vi "UHR-Fleezers Control (host) -Leonardo 04-2018 V8_Redesign.vi"() -> ()   [LabVIEW 2013]
uses:
  <vilib>/Utility/miscctls.llb/LVMinMaxIncTypeDef.ctl
  <vilib>/Platform/TimedLoop/XDataNode/timing_clust.ctl
  <vilib>/Platform/TimedLoop/XDataNode/nitl_modes.ctl
  <vilib>/Platform/TimedLoop/XDataNode/wakeup.ctl
  <vilib>/userdefined/High Color/nirio_resource_hc.ctl
  <vilib>/Analysis/baseanly.llb/Mean (DBL).vi
  FPGA VIs Alex/Alex subVIs/Downsample1D.vi
  FPGA VIs Alex/Alex subVIs/Integrate1D.vi
  <vilib>/FPGAPlugInAG/PCIe-7852R/niLvFpga_Open_PCIe-7852R.vi
  <vilib>/FPGAPlugInAG/PCIe-7852R/niLvFpga_Reset_PCIe-7852R.vi
  <vilib>/FPGAPlugInAG/PCIe-7852R/niLvFpga_Run_PCIe-7852R.vi
  <vilib>/FPGAPlugInAG/PCIe-7852R/niLvFpga_Close_PCIe-7852R.vi
  <vilib>/Utility/error.llb/Error Cluster From Error Code.vi
  <vilib>/rvi/errors/niLvFpgaAdjustHostInterfaceError.vi
  <vilib>/rvi/interface/common/niFpgaWaitOnOcc.vi
  <vilib>/Utility/inputDevices.llb/mouseAcquire.vi
  downsample 1D array - double.vi
  <vilib>/express/express analysis/Spectral/Block/exnSpectralBlock spectral measurements PSD poly.vi
  <vilib>/express/express analysis/Spectral/Block/exnSpectralBlock spectral measurements PSD WFM.vi
  <vilib>/FPGAPlugInAG/PCIe-7852R/niLvFpga_Abort_PCIe-7852R.vi
  openfpgaref.8.6.ctl
  <vilib>/Platform/TimedLoop/XDataNode/XDataNode.xnode
  <vilib>/rvi/interface/nirviOpenFPGA/nirviOpenFPGA.xnode
  openfpgaref.initrf.ctl
  FPGA Bitfiles/UHR-FleezersInst_FPGATarget_intitializeRF201804.lvbitx
  <vilib>/rvi/interface/nirviMethod/nirviMethod.xnode
  <vilib>/rvi/interface/nirviCloseFPGA/nirviCloseFPGA.xnode
  FPGA Bitfiles/UHR-FleezersInst_FPGATarget_UHR-FleezersCont_IqK95Pvv9lYv5.3.lvbitx
  <vilib>/rvi/interface/nirviReadWriteControl/nirviReadWriteControl.xnode
  <vilib>/express/express analysis/Spectral/XNode/ExpressSpectralMeasurementsBlockNode.xnode
  <vilib>/Platform/TimedLoop/XDataNode/XDNodeRunTimeDep.lvlib
  <vilib>/Analysis/NI_AALBase.lvlib
  <vilib>/rvi/errors/niLvFpgaMergeErrorWithErrorCode.vi
  <vilib>/FPGAPlugInAG/PCIe-7852R/niLvFpga_ConfigureFifo_PCIe-7852R.vi
  NiFpgaLv.dll
  <vilib>/FPGAPlugInAG/PCIe-7852R/niLvFpga_ReadFifo_PCIe-7852R.vi
panel:
  in  "Tab Data Protocols":T1(tab)
  out "Extension":waveform(dbl)(graph)
  in  "Trap Pos. FB ON":bool
  in  "Set SP to Current Frc":bool
  out "Current Trap Delta":dbl=20.03845214843774
  in  "MCL Tracking":bool
  in  "Target Force (pN)":dbl=10.5
  in  "Save ave factor":dbl=1.0
  in  "Step Size (nm) 2":dbl=0.34
  in  "N Steps":dbl=20.0
  in  "Take Stepping Data":bool
  in  "APD 2 Offset":dbl
  in  "APD 1 Offset":dbl
  out "Mean":dbl=1.039039384389187 caption="Mean (pN)" format="%#_3g"
  in  "Calibration":u16(ring)=2 items=["None", "Position", "Force"]
  out "T1 X":dbl=-1.511158478291593 caption="T1 X (pN)" format="%0.2f"
  out "T2 X":dbl=0.5669202904867809 caption="T2 X (pN)" format="%0.2f"
  out "Difference":dbl=0.9442381878048121 caption="Difference (pN)" format="%.2g"
  out "Data Period (s)":dbl=1.4999999999999999e-05 caption="Trap Data Period (s)" format="%#_6p"
  in  "Tab Action Shortcuts":enum32{"Actions", "Calibration", "Fishing"}(tab)
  in  "Use Full Offset?":bool=TRUE
  in  "Cal/Data Acq. Spot":bool
  out "Fish Status":u16(ring) items=["Off", "Approach", "Wiggle", "Extend", "Tether Found"]
  in  "Toggle AFish":bool
  in  "Offset 2 Set":dbl=2.0
  in  "Offset 1 Set":dbl=1.0
  in  "Cal @ (MHz)":dbl=20.0
  in  "W/ Offset 1":bool=TRUE
  in  "Offset 1 Start (MHz)":dbl=13.0
  in  "W/ Offset 2":bool
  in  "Offset 2 Start (MHz)":dbl=16.0
  in  "Trap 2 Bead Size (nm)":dbl=1000.0
  in  "Trap 1 Bead Size (nm)":dbl=1000.0
  in  "Extend Min F":dbl=1.0
  in  "Extend Min TD":dbl=8.0
  in  "Extend dTD":dbl=5.0
  out "AF Time":u32
  in  "Wiggle time":dbl
  in  "Wiggle TD":dbl=1.0
  in  "Max TD":dbl=15.0
  in  "Min TD":dbl=8.0
  in  "Approach dTD":dbl=-5.0 format="%#_13g"
  in  "Stop All":bool=TRUE
  in  "Tab Control Display":enum32{"Main", "Imaging", "Display All", "FFT"}(tab)
  in  "Clear FX":bool
  out "Force-Extension":cluster{"x":dbl, "y":dbl}[](graph)
  out "Force":waveform(dbl)[](graph)
  out "APD Chart":waveform(dbl)[](graph)
  in  "Ext Offset (nm)":dbl
  in  "Take Green\nLaser Image":bool
  out "APD 2":T2(plugin-control) caption="APD 2 (Cy5)"
  in  "Flip Green Filter":bool
  in  "Set X Only":bool
  in  "Set Y Only":bool
  out "APD 1":T2(plugin-control) caption="APD 1 (Cy3)"
  out "Detection Laser Y":T2(plugin-control)
  out "Pointer Y (V)":dbl=4.0025870540482815 format="%_3g"
  out "Pointer X (V)":dbl=4.635613485356835 format="%_3g"
  in  "Set Confocal Spot":bool
  out "Detection Laser X":T2(plugin-control)
  out "All Signals":waveform(dbl)[](graph)=[{"t0"=timestamp(2751.0000000002074 s since 1904-01-01), "dt"=0.02, "Y"=[0.0, 0.0, 0.0, 0.0, 0.0, 0.0, 0.0, 0.0, 0.0, 0.0, 0.0, 0.0, 0.0, 0.0, 0.0], "attributes"=variant("NI_ChannelName"=variant(string "APD 1"))}, {"t0"=timestamp(2751.0000000002074 s since 1904-01-01), "dt"=0.02, "Y"=[0.0, 0.0, 0.0, 0.0, 0.0, 0.0, 0.0, 0.0, 0.0, 0.0, 0.0, 0.0, 0.0, 0.0, 0.0], "attributes"=variant("NI_ChannelName"=variant(string "APD 2"))}, {"t0"=timestamp(2751.0000000002074 s since 1904-01-01), "dt"=0.15, "Y"=[-0.020049210394969354, -0.02003592505550746], "attributes"=variant("NI_ChannelName"=variant(string "T1 Y"))}, {"t0"=timestamp(2751.0000000002074 s since 1904-01-01), "dt"=0.15, "Y"=[0.03074231675925172, 0.03074526419399293], "attributes"=variant("NI_ChannelName"=variant(string "T1 X"))}, {"t0"=timestamp(2751.0000000002074 s since 1904-01-01), "dt"=0.15, "Y"=[2.9160941496017294, 2.916128360850853], "attributes"=variant("NI_ChannelName"=variant(string "T1 Sum"))}, {"t0"=timestamp(2751.0000000002074 s since 1904-01-01), "dt"=0.15, "Y"=[-0.002644972968316131, -0.002638961391604115], "attributes"=variant("NI_ChannelName"=variant(string "T2 Y"))}, {"t0"=timestamp(2751.0000000002074 s since 1904-01-01), "dt"=0.15, "Y"=[-0.011335016186436862, -0.011341032214389745], "attributes"=variant("NI_ChannelName"=variant(string "T2 X"))}, {"t0"=timestamp(2751.0000000002074 s since 1904-01-01), "dt"=0.15, "Y"=[2.746599475081634, 2.746642933439132], "attributes"=variant("NI_ChannelName"=variant(string "T2 Sum"))}, {"t0"=timestamp(2751.0000000002074 s since 1904-01-01), "dt"=0.15, "Y"=[-0.526083166086966, -0.5261552546492463], "attributes"=variant("NI_ChannelName"=variant(string "T1 FB X"))}, {"t0"=timestamp(2751.0000000002074 s since 1904-01-01), "dt"=0.15, "Y"=[3.0920304879909737, 3.0920243537705665], "attributes"=variant("NI_ChannelName"=variant(string "T2 FB Sum"))}, {"t0"=timestamp(2751.0000000002074 s since 1904-01-01), "dt"=0.15, "Y"=[-0.7128125059590501, -0.7128388598091219], "attributes"=variant("NI_ChannelName"=variant(string "T2 FB X"))}, {"t0"=timestamp(2751.0000000002074 s since 1904-01-01), "dt"=0.15, "Y"=[2.9122738731040343, 2.91227808465834], "attributes"=variant("NI_ChannelName"=variant(string "T2 FB Sum"))}, {"t0"=timestamp(2751.0000000002074 s since 1904-01-01), "dt"=0.15, "Y"=[-0.0023344523453474137, -0.002339854121524665], "attributes"=variant("NI_ChannelName"=variant(string "PSD Y"))}, {"t0"=timestamp(2751.0000000002074 s since 1904-01-01), "dt"=0.15, "Y"=[-0.0026477858821374683, -0.002642139957884409], "attributes"=variant("NI_ChannelName"=variant(string "PSD X"))}, {"t0"=timestamp(2751.0000000002074 s since 1904-01-01), "dt"=0.15, "Y"=[0.014415417950986964, 0.014429639576402777], "attributes"=variant("NI_ChannelName"=variant(string "PSD Sum"))}]
  in  "Signals to Plot":i32(listbox)=9
  out "Trap Disp. Freq. (Hz)":dbl=6.666666666666667 caption="Freq. (Hz)" format="%#_6p"
  out "Display Period (s)":dbl=0.15 caption="Period (s)" format="%#_6p"
  in  "Trap Disp. Downsample":i32=10000 caption="Downsample" max=20000
  in  "APD Disp. Scale":dbl=0.1 caption="Scale (Divide,\nfor above plot only)"
  in  "APD Disp. dSamp":i32=2 caption="Integrate" min=1 max=30 step=1
  out "APD Display Freq. (Hz)":dbl=50.0 caption="Freq. (Hz)"
  out "APD Display Period (s)":dbl=0.02 caption="Period (s)"
  out "FFT 1":cluster{"f0":dbl, "df":dbl, "magnitude":dbl[]}[](graph)=[{"f0"=0.0, "df"=16.666666666666668, "magnitude"=[-331.1367572010275, -79.05506245821404, -86.61411242440559, -88.4728176091699, -90.3181253945935, -94.12566333707997, -92.52740723119955, -94.92192587982518, -99.60936585245742, -96.87568627870715, -94.02570383337763, -83.8058550151726, -97.57441397235512, -101.59968530846606, -101.523049255742, -103.35038532190343, -101.58594091014982, -102.96098031851216, -91.39759462745924, -103.75019963279499, -104.45030075054324, -103.04245334279298, -104.0720279134107, -106.06482372394834, -103.69131867828104, -104.40395035115309, -105.96420043276396, -107.6735556337804, -106.673030006608, -107.34889066208132, -108.05626565233933, -106.25659018850432, -105.29934513380842, -105.43096056709592, -108.3728498841465, -106.0555440144992, -105.78001282181421, -107.48741857324953, -108.67624970548897, -105.39976667156175, -105.91413119232612, -109.4222808198164, -107.0898971593174, -107.91164191890915, -108.26032038855709, -107.58332347164534, -108.23559688234297, -108.01271040303237, -107.66511723652701, -106.51901583170391, -109.27249501469946, -108.55647681594805, -107.93499259231463, -107.05068166453935, -109.13641475410455, -109.29679733781423, -108.19360835527803, -109.57747591546632, -109.58364591011674, -110.47061433372711, -109.8144340420426, -108.79067462293897, -107.54887553357234, -107.99559866705923, -108.85023923652685, -109.68733225238618, -108.51101278437793, -108.51620475114115, -108.22212402200637, -104.63726950302143, -110.2989919678048, -107.61796444414897, -108.68882962798736, -104.79193983043893, -103.59504263746938, -93.64633660288543, -101.9191640501395, -105.73717393151816, -108.92572458793902, -107.43962662800902, -107.79595323081325, -107.0923101993207, -108.17603277205289, -107.87074270713183, -109.20899066381877, -108.61832060412445, -109.10072003106593, -105.76480632823524, -108.60877649218978, -109.67541158970121, -110.2286232768028, -109.84952155309578, -109.33772024076384, -109.95251642394683, -110.14777282585466, -109.13825677905699, -110.05989365698167, -109.39359990189426, -110.56255614635295, -109.66477183197163, -108.9397158528824, -110.26529907650465, -109.20049464984628, -108.20183857013548, -109.09752250184418, -108.00440442238454, -108.35465963524055, -111.16774134451799, -110.34812550238405, -108.94506763426756, -108.72845542102493, -109.41512344014713, -112.44661664432377, -110.35437330889101, -111.32939440655925, -109.42989530434981, -110.98084669076195, -111.92160561143541, -108.57755551751093, -111.40042616180912, -110.15284955891853, -112.21455132279115, -111.40787773511747, -108.82949641635288, -110.13442122547907, -111.42229298204664, -112.06314940885191, -110.6015308813694, -109.51144097251623, -111.15989713761475, -110.25535755335385, -109.65868178057926, -110.51649885452997, -109.77194745285269, -108.4234206864394, -109.50892632093968, -109.46471287444389, -107.92241289271415, -109.72283805386196, -108.63426821579918, -110.37316681536255, -111.09713996884652, -110.32903619589223, -105.32012665515045, -107.36858557554393, -108.00382215905725, -110.06430686942338, -108.81666625979916, -110.01277074453823, -110.94194741225512, -109.65934609082873, -107.80979136006962, -112.81333866824724, -111.61474300955487, -109.83998277184975, -109.45953946904639, -109.79640584952526, -108.19172301667324, -109.28894656674316, -107.61471301278785, -108.83814006090513, -109.08866847726084, -108.20250571862371, -107.96222236861584, -107.03811197900873, -108.93533000393974, -107.74482548035408, -110.79811544577694, -111.1387476496877, -107.42970105883512, -109.18442281176472, -108.73546184641192, -108.71800246690864, -108.51945944378063, -108.06825856571285, -107.27210712368412, -108.12304695877637, -107.84933283677306, -109.73682373154998, -109.32284761503395, -109.31328817453769, -106.68762108642842, -109.79203616876461, -109.9020278896408, -110.27080024357275, -108.54152101558762, -111.00464391726017, -112.42244020766577, -110.82707315747889, -111.00344011890857, -109.90461839395674, -109.42877207451863, -109.73549298167016, -111.67494793393293, -108.85799077901427, -108.5348443278263, -109.803781083881, -108.30644755543659, -108.5079527456017, -111.2055351312823, -108.53089994340155, -108.01739789012176, -108.70360662855235, -107.95873456794631, -109.58297170693093, -108.9372401694271, -110.15921663527153, -109.22399119911955, -110.89883651739237, -108.92840112258382, -110.0545300523626, -109.05961065387005, -109.45831398589371, -108.61239387653227, -110.13001256174265, -108.80060224137931, -109.46327400696283, -108.0177965824709, -109.29727944627197, -110.3237255895986, -109.03258262543821, -110.97880178489321, -109.70034895077919, -111.16405638194153, -109.17324451464711, -109.65698250854277, -108.96750235822178, -112.00534231585624, -108.69274607723942, -108.98110446396657, -108.40723795464795, -111.44459094807324, -111.74799245277113, -111.1601960491512, -108.92048232753773, -110.30506377784799, -111.33145973979093, -110.91850998672503, -110.33684985776448, -108.90206518366908, -109.28458878227542, -108.98773986023751, -110.85813863075646, -109.00041591105906, -110.84543686681204, -109.84382395806176, -109.69722434763266, -108.50915601095721, -107.80829925826895, -110.59736107582401, -109.75377770317087, -109.3992084496136, -110.51151565846742, -112.49753959826434, -109.7299632589479, -109.54070743868353, -109.90314341132164, -111.05974202976806, -109.03766862152392, -109.46667095459878, -109.52800799036197, -111.3163121356807, -110.07817134522178, -108.69251657453547, -109.40472158898045, -109.71400709815576, -110.60534468715097, -109.46937396724682, -107.70342491418788, -109.86331122597839, -108.64971387994616, -110.90117371097081, -108.34928840565928, -110.04172889660904, -111.52979926554961, -110.34759300823305, -109.62712781837159, -109.24131154553284, -110.23196152450447, -108.68509612326807, -108.0246905483419, -106.61876139289784, -101.5519630114271, -80.57695480953835, -102.03744443354402, -107.1449217193017, -110.0695213407169, -106.61597783999268, -110.79221011808191, -109.58974545931426, -109.1149802216988, -109.20993813088597, -109.63768480465863, -110.10428394219181, -109.08445084271477, -108.83472375362581, -109.69508502050168, -108.05588796178941, -110.62586360101581, -109.95315261676905, -107.52208264977473, -108.80708007514875, -110.43484881098874, -110.45942171588936, -107.83804717866751, -109.98973910294193, -109.3496496054193, -108.425252911127, -110.94579264380809, -108.54181722177951, -108.67696070083541, -108.4150202151644, -109.24973583101504, -112.0454922608961, -111.29046597340738, -110.75018248960077, -109.38326363603683, -109.2033340336957, -109.45076170874889, -109.52878049853727, -109.32340869724774, -110.98123395128233, -110.75736340635505, -109.7218385823809, -107.97422606064993, -109.77313701758703, -110.95948744392717, -110.08996774172691, -108.51011830110778, -109.78063140243836, -110.65996628628228, -109.83684298615616, -110.33329049188029, -110.13755118968292, -110.3717925645783, -108.55302219178951, -106.86811628734195, -108.6302156589162, -108.75341391045045, -108.32589578384841, -108.70061474734084, -112.30742263527534, -109.16842570592085, -109.29767035534508, -108.87829025017463, -108.2255616391397, -108.4316108616088, -108.82995906929271, -110.40135575415563, -109.51623498946435, -109.79409808792403, -107.03832759632121, -108.36534528684132, -109.72010868372905, -107.90933028179892, -106.95643597294047, -111.29929166165778, -110.23001135794706, -108.98838015381585, -109.79115357104436, -108.18627479511115, -108.14988122174307, -109.12074063466532, -109.41904850488358, -111.40409873721113, -108.83156790193294, -108.77032248953847, -108.88363158686694, -108.47515048290681, -105.94172147874599, -109.38146940214403, -109.21277078848794, -108.11309390545507, -110.70840012427504, -109.5504457849329, -109.52330684534209, -110.06776026911132, -108.21949434182314, -111.21266686269992, -108.78581501170974, -108.43115799297222, -109.63260325780062, -109.84070220619535, -109.72041980780126, -110.29615941882527, -110.60316734262464, -108.79165446414692, -110.95840439895592, -109.64926233107009, -109.16526769544322, -108.65292362430982, -109.56113898129935, -109.85693046339026, -108.92316027325207, -109.79492493553914, -109.38157962945887, -110.24545136266825, -109.30031463492487, -109.0795429936869, -111.4091719525013, -108.63499083917162, -108.43863465339358, -109.23207864880891, -111.21947487191643, -109.24525201480154, -109.56842406077318, -109.46711940800672, -111.91389548262572, -108.15655736690546, -108.71882059966947, -111.26328503478568, -110.95027143873176, -108.4853106242357, -110.36902802777546, -109.9314203579182, -108.77686164101732, -108.71871020068312, -111.04829661168574, -109.95072655339462, -109.88221342875462, -109.53241732756136, -108.2625005404823, -108.00677030040697, -110.19659317581693, -108.93858924796267, -109.46817875483995, -110.78063992017232, -111.11066570318451, -110.78774336696706, -109.19199744617812, -108.54914256407436, -109.28414960420909, -110.64143585101183, -110.5855350821307, -109.47578632252726, -108.89705360836223, -109.89214013612292, -107.93271261027171, -109.32631601340563, -108.60274611341092, -109.40110159872573, -110.889237682208, -110.01391165813328, -109.99747108785071, -108.65542819213674, -110.37211847668736, -110.44656500845738, -110.8128133834973, -108.8909299260433, -110.19551227077532, -111.37647266643523, -110.83802189730321, -109.98519377913681, -110.52378970770522, -108.16970420057817, -110.70974729773344, -110.76836765494402, -110.26884275594577, -109.22041044268806, -109.87809744746195, -107.76823252107832, -109.12119474042969, -110.28066108731146, -108.55000033509207, -110.18152097767907, -110.73030521152278, -111.49470908029893, -110.2320929919509, -110.03370979233021, -109.79181668155233, -108.6673501209991, -109.86695766650877, -107.88926518046961, -110.95525003776572, -109.18130359755742, -110.42618009658618, -107.90341931158893, -111.44736855661769, -110.72634267386593, -109.29945988519303, -107.67889101961411, -108.81148059987765, -109.13375212757057, -109.8122873383549, -109.80176697684155, -109.96342275204768, -109.90406635707086, -108.75674342748256, -110.12362902701081, -109.82151095527837, -108.62543344241836, -110.09171852771195, -110.21434637862887, -109.97254504855631, -109.27043209093468, -111.35149588204125, -110.12399876776051, -111.65983675538546, -109.28788875768564, -110.86554069990251, -111.26990906470603, -108.60956517491746, -111.49613890850938, -111.79685722966795, -109.26269485364045, -110.38555615546439, -109.40641023162068, -110.966136593156, -108.78892524584494, -110.29340727375603, -111.44032043281035, -109.95212021173755, -109.79233511584334, -112.41184021118175, -109.73687851881148, -108.65493879781806, -110.76132988919045, -108.43230346094671, -110.32968175895853, -110.29890782023821, -108.77609076424456, -110.3298662333555, -109.47734504217333, -108.2677295732245, -109.21234363352882, -107.83278941978479, -108.85136784424789, -108.43241251530755, -109.76609391460555, -108.53204373005357, -110.9660641972934, -110.3152512161094, -110.72570499399905, -109.23877906286317, -111.72407743101837, -109.20311421918561, -108.06021800233717, -109.29288625761943, -108.78395253409145, -111.85250172876302, -108.78827588901797, -109.79775055719482, -109.12089297455859, -109.49896359356035, -110.34432647103819, -107.94700097960238, -109.30489238477631, -108.89170290869342, -108.82574563272509, -110.11024077194833, -107.37946433552314, -109.60167933458756, -107.80625057819019, -110.11489057210264, -107.35436859378505, -105.69819484613895, -109.11280625683739, -109.27770293057978, -107.7053735252589, -109.75022444894368, -109.3310543596577, -107.87683693707739, -108.19931495338068, -109.26462246191564, -106.71885779297867, -100.00018022217961, -92.54434511397295, -107.20472143807373, -107.39203415155283, -110.04461177268398, -108.48860496315312, -109.0057168110333, -108.37627790492552, -108.4108380728248, -109.65509454313073, -109.64243000632982, -97.04219069306761, -109.0928856629964, -107.9760697315632, -107.52611064047497, -108.87702814778996, -109.08437599027614, -110.70097118837974, -109.00969860961283, -110.38275386163214, -110.0699155421545, -106.91498895181175, -106.22178738309017, -109.36827866896039, -107.59953130968307, -109.19516217272808, -108.31502495393616, -109.384158926223, -107.11670654202719, -108.09436312738853, -110.14559230873704, -109.84997663447679, -107.83465335309926, -108.60947100624459, -108.9932479423645, -109.17174810371898, -108.79457339828916, -109.40909327982367, -109.6328723628302, -109.51081854476179, -107.63054408568418, -109.63728404010122, -108.51163794839918, -107.55002282725216, -108.97796212764939, -107.24648164623483, -112.21470452291085, -108.74294024554423, -109.62070777514892, -108.05768666239368, -109.8224946685739, -109.34575507446003, -108.53536952609525, -109.60789300457671, -107.56681538208278, -109.22777325016398, -108.79047910308894, -110.10332477250668, -108.00206387955672, -108.45604004720035, -109.00645795765472, -109.81039564269616, -108.92785144634745, -108.3978471520567, -107.94411095685999, -110.53486519304262, -108.8773780319227, -109.03345093296107, -107.30746693745031, -108.54277704832029, -108.77629108166091, -108.91111762599647, -107.74965195880401, -109.97375370738439, -109.76326492689246, -107.91717581777407, -109.0730556927617, -107.66804873204664, -110.40438871064791, -108.05794247751498, -108.80206615156494, -107.51329354700796, -108.83687012994949, -107.57713176895379, -107.94774159581414, -109.41894615439651, -107.10869425078764, -110.51480854078629, -108.92221367099775, -109.91358786461535, -110.1744263092835, -109.30795472883494, -107.91359710691006, -109.77888185049835, -109.52060975706438, -108.66686651982212, -108.71041801553639, -110.13619546359467, -108.87957097273856, -109.72150387215271, -109.00776068810654, -109.70251113927438, -110.75769213896399, -108.53234896741436, -109.69439526582246, -110.15412541604617, -108.25183374628219, -107.97402569656481, -110.34920156998648, -108.45106995186384, -108.82031145748209, -111.38690005057539, -107.01968459818563, -110.3044500039584, -110.8755481852125, -111.08915057663255, -107.94824988655199, -110.21669144934839, -109.90539774633154, -109.58985438756767, -110.12258796623348, -109.41689951612143, -109.31128210476795, -109.00258476567323, -109.11093063041056, -108.83347064311234, -108.32685287566952, -109.44770946560935, -108.40145063144861, -109.68448193892085, -108.76525439243828, -107.62837139034596, -107.39300298848994, -109.36993934990318, -109.2465218489418, -106.66307369796812, -110.15891092764934, -109.57151745419041, -108.92425698310808, -109.8036704717834, -108.79751146756549, -109.25926431818017, -108.46260574057584, -109.1967554647261, -110.63319560262356, -109.02343067385144, -111.22073171487528, -109.4731095097105, -109.69335000085164, -109.48782989577005, -107.95204227683271, -108.19468255763758, -111.36195112053247, -109.55696116543685, -110.3130767640534, -108.9621824253354, -109.99735074896789, -109.20198058456344, -108.12100614259485, -111.27227490807289, -110.09248554008288, -109.14395535060149, -110.80882692379708, -109.22632926901655, -108.64497210802793, -111.00030482190711, -111.1317849358033, -107.43140429257826, -107.9783302193555, -109.2639893652291, -108.97008485446163, -108.66556668859064, -108.12995785876932, -109.73001061107855, -108.09691302413727, -110.68391499215569, -112.78583642012705, -108.7093037763389, -110.67868795924797, -109.0190959349128, -108.36247198231372, -109.82829353258869, -108.24916379311045, -109.84154533905823, -108.55470160833775, -109.75438989348815, -108.82865632118325, -107.63622268162582, -111.00943492886312, -110.81824358463759, -109.46028423652966, -107.52479398900992, -108.99087806823736, -109.94494831750349, -110.26788355564504, -109.8954055022304, -106.9478122391182, -108.91705388158901, -107.76095584490312, -109.28456723055147, -109.7982307261767, -108.98552661346622, -109.98937979783426, -110.57907422426224, -108.68113463944836, -108.06257240208589, -110.0707224529617, -109.19515280354733, -109.35868842818849, -110.37311467065695, -109.0404734478992, -108.16686395270187, -108.61859220485148, -109.19986437876149, -108.19707189725302, -110.06564239663074, -108.87850403465154, -110.63824157544798, -107.36918104067212, -108.7008736325543, -110.9359398265406, -111.08529123080929, -108.44209934821818, -109.79529621208783, -108.38917887958179, -108.169117639508, -109.24332926356216, -110.50584058811704, -109.63592524002665, -109.32261039377495, -109.16720880524552, -109.3084314664462, -109.5812223978583, -107.70213196487856, -108.0557884982431, -110.67058020007828, -111.68459781023608, -109.66270627185824, -110.52536245663693, -109.70208409132103, -108.78645420809342, -109.23122088059863, -109.24601474121832, -111.25604763816514, -109.50225851581177, -107.32434217163818, -109.28548556764925, -107.59972621660836, -110.46928774723048, -109.25950101547609, -110.32016453935465, -107.78482761561703, -107.89462895091089, -107.51366154391481, -108.08036891159172, -109.53371809947035, -101.2452927166745, -109.32763325689056, -107.52166868423687, -109.89648659445174, -109.11350200980485, -109.81336712738089, -110.02799517445062, -108.02767143538516, -107.97850220501483, -109.50772934896838, -109.31069875721964, -108.49991657749598, -105.60880911233095, -109.79128597340213, -106.91084537903113, -107.84880087118997, -109.63628170511824, -109.03203967193224, -110.64186113413658, -110.98027990365594, -112.33841002907062, -111.01793075565425, -108.58025797022215, -110.4259296883756, -110.38643255981424, -108.93051671115133, -110.97544177116494, -108.63883100482677, -108.37581711765226, -108.90240163126536, -107.94688047875466, -109.9482937437732, -110.09097112364414, -110.09805032265376, -111.44307114024532, -109.15483789122554, -110.9713708217832, -107.8548737634672, -111.41418477109195, -109.45699779859628, -97.03595099331734, -109.16746744169623, -109.66209204485918, -112.57048704774604, -109.73989735035725, -108.16252575067017, -110.7546980664636, -108.91536673403449, -109.20509151422344, -111.0260632167785, -109.62924582406518, -110.45466277291722, -110.2973970018937, -109.67550222925419, -108.84481022020094, -107.23686414357573, -111.79004633370906, -109.85453094194085, -109.45617270081004, -110.73920606732504, -108.90879956851099, -109.67774425528265, -109.4745715721361, -110.18080454693559, -109.26079184315502, -109.41692499885505, -109.02240975088358, -107.80833423058168, -109.32657361431549, -107.87138278655101, -110.910364670719, -109.70067156846706, -108.55301754282077, -109.4243252157005, -109.77567725161107, -107.83737232063925, -110.36509412773016, -109.6371048811367, -109.49430894422814, -108.55509251499753, -108.03996302911446, -110.4385715838736, -110.08864436068788, -109.48922484379962, -109.90865554258562, -109.7491963238264, -110.04796094537969, -107.413043439116, -108.54229076126079, -108.2522516728666, -109.75464941327974, -110.26795832300996, -109.28073673851144, -108.62990200974927, -109.89408067552287, -109.09160284731726, -109.90740624925795, -109.92534708896517, -109.79578862362752, -109.97278346890566, -107.80679350393824, -112.81728446281548, -108.09689504419987, -109.89549991422173, -108.43930976031248, -109.95153099843282, -108.18277483720716, -111.89607792605433, -109.52567003805, -109.17125106979698, -109.64300739407085, -108.21045178846524, -109.64036472149706, -109.02324448538845, -109.039163008889, -110.41006510134076, -109.50289952116489, -110.4732620447796, -110.08777181504614, -110.15589511434341, -109.55705089158471, -109.2547682932589, -110.86823885471617, -109.96330502176939, -109.85995369810554, -110.63211290903473, -112.08007783432191, -110.24725218052279, -107.62861148917592, -110.08691795849435, -108.89793794632287, -111.07702220466341, -109.46946126482341, -109.19747345337464, -110.70018609416007, -109.66366205691908, -110.78032312133551, -108.05724200456513, -108.195661625627, -110.90724508408255, -110.08307674771669, -110.76863516643007, -110.46620425061583, -109.16986788877276, -109.61921294239114, -108.51159432329543, -109.96308336765689, -107.38178944242856, -111.95930944846394, -109.3329826827624, -109.59119636368249, -108.83148571828912, -110.46194288788257, -105.87694286145472, -107.985886302892, -109.2975019660806, -111.05138725716857, -109.60005889204612, -110.92871351729086, -110.73480546964537, -108.41587420326718, -109.84275465824477, -108.8249071047676, -107.65358887817105, -108.3254150042995, -111.47362100321767, -112.7287536850025, -108.8217125660507, -109.50232320231771, -110.29587061625348, -109.30644535112089, -107.69178032077258, -110.84522325672016, -109.3735891463141, -109.12506388923123, -109.65582307934665, -111.11427272192576, -112.19827973435466, -109.11306367925813, -108.19203577968261, -107.89831568266465, -108.85805249169313, -109.51100049661844, -111.71546684086955, -109.53880495724334, -107.07739286222231, -110.66836728754211, -111.5415170557177, -110.16051267940297, -110.6107546662698, -111.36389129556191, -107.77888179117923, -110.34160392509817, -109.61287125994414, -110.23791773883013, -111.00669159903549, -110.97165069538953, -109.43965413392434, -110.6813161690388, -110.31441293654314, -111.96129906273796, -108.15998218707462, -110.08095912053633, -109.41084567452768, -109.28774416263552, -110.80159950384204, -110.41956747809755, -108.85005186267244, -107.9069227847757, -108.84249369063123, -109.92569208845894, -109.34109797584448, -109.41334788055491, -108.76462023086997, -108.22069272136177, -107.0786679601274, -108.30206755098202, -108.57613406368954, -110.83330887636482, -111.93966942736989, -109.76373713473264, -108.25782074884941, -108.16490627215555, -109.93351470267982, -110.75525684428368, -108.22814762283093, -109.73442331991602, -107.53145627482685, -108.27195221226805, -110.33032779278457, -109.48951857415828, -108.12599093700939, -107.97627415508097, -108.81426859968796, -111.21764717894752, -109.80856212352333, -110.92658779118501, -109.71551885834796, -110.38682741010847, -108.87671328341361, -109.68368600774755, -108.35359806351899, -111.7519400010676, -109.89407081573103, -108.24301180922755, -110.00646944788126, -108.6685299083706, -107.52856885980722, -111.7622363038509, -111.0025144494897, -108.64719599357296, -110.62968467177518, -108.821509935539, -107.94915453463719, -111.53070432277694, -109.87282048586256, -110.71167589371663, -109.79225006081626, -109.96203471712074, -110.29921092232489, -110.10644439440416, -111.28815007382043, -111.19165661703703, -108.46024117100558, -110.22528296512183, -110.32184972386672, -110.05120383416072, -109.78792549362107, -109.00355659956696, -108.85989369286315, -113.00899556732638, -110.91756826567867, -111.25016866167897, -111.84225040552181, -110.54451635944174, -110.72722829912917, -109.60759702177283, -110.49362602516815, -108.74419542915284, -110.3379671069179, -109.66259088220754, -110.45956400953156, -109.13956157147233, -109.27130155486806, -110.83015602667983, -109.17970724944131, -109.09662765889193, -108.0447366108107, -108.9536269357457, -110.35663108940085, -108.73418835472056, -113.42965806805827, -111.81270536656905, -110.06155590173537, -108.76582224646269, -106.7488061675813, -108.5700320158723, -111.11038264410035, -110.41435767488723, -109.12763443489911, -109.30517580756394, -111.61251165371237, -109.8116632664339, -109.36845864976851, -109.00390009629231, -110.54359197165573, -109.52629258465976, -110.75932197632896, -109.50903215359567, -107.42652056246085, -107.81146496533543, -103.22224383145215, -108.53803076819163, -109.78623360072066, -109.66306634612869, -110.80245829141279, -111.87835085452016, -102.27372781471168, -111.27763038431458, -108.45838423437681, -108.79077917058028, -109.31951755762685, -110.05415097017186, -109.5535934823387, -111.62732254641111, -110.73478247119641, -109.9468722686683, -110.39698367573979, -109.30612942398305, -109.7578384694043, -109.34817295524313, -105.56944757301993, -110.1940418750125, -109.27076023513962, -111.03491935225027, -112.2980497521063, -110.65725497955563, -109.0567530102422, -110.31700596563523, -109.64508026365678, -109.6190471404421, -110.52566833759428, -109.68595899227789, -109.7431160985074, -110.4798230300751, -109.45506977604765, -110.69504157940786, -110.63067849573177, -108.06456949500138, -107.99354148885966, -108.11349194720599, -109.15944121207349, -110.61766925164031, -110.14145801314527, -110.67420842201165, -111.91532881806512, -112.15901550030345, -109.94774413630104, -109.2819568305201, -110.94623189179737, -110.17685430287735, -110.39082916961016, -109.53953238698966, -110.76940623620611, -109.89327922318515, -109.10275695043765, -110.21445972656734, -110.58968777252528, -110.57016757660259, -109.59208496373341, -109.07946946465374, -109.10762003745964, -110.36892993974607, -109.81864495218393, -112.12972189864566, -109.26185849434863, -111.56305819991357, -111.36019621828058, -110.3397604159226, -109.58675612753163, -110.58041217474447, -106.34739062044932, -108.6722699609389, -110.03906060709869, -109.16794717548382, -109.65012481802809, -109.35377624077988, -110.51889143862303, -110.03397458059777, -110.7981307056636, -110.56653507062292, -107.61367005067231, -109.99279736988825, -111.79875182878175, -108.60382315996031, -109.71381533228038, -108.60388131505613, -107.0933685540362, -107.86037690830757, -108.40980028847238, -108.83869602763895, -110.76921375395764, -109.96766364716046, -110.8256171465781, -110.13805084291067, -108.5349140035878, -110.57158437465219, -110.8920694413417, -108.71646695477324, -108.33274238445665, -108.96152108305608, -111.03750932994224, -109.48915027983756, -110.29725207211165, -110.79527247268442, -109.47969936716117, -109.79306701834035, -110.16840035577498, -110.29840230783668, -109.15306387075587, -110.72651274964761, -109.08881658764956, -110.8349724030761, -110.64653625576447, -111.40392562616867, -109.94581588927414, -108.85136340231294, -109.77228546607624, -111.48297395390018, -109.7334001251941, -109.30537415590783, -109.63937411233408, -109.69785848648013, -109.3523781030017, -112.04667421182404, -111.56311816195343, -108.18548447362308, -110.63388993686104, -111.39768634137992, -109.87157345395542, -108.6734208287271, -109.46213300216168, -111.75774769437145, -110.10245994173216, -109.52385139033495, -110.96513097775451, -111.8709319163154, -111.54948269614047, -110.29760900080463, -108.52168175904663, -111.09033925738258, -111.14752744054172, -108.83074523709202, -109.05704141259113, -111.74377805749482, -109.57200906899736, -108.84121318623825, -110.86657990204343, -109.54363603755047, -110.89448416316372, -109.58965570570145, -110.21012263847972, -110.4063470702923, -109.5021950342969, -110.33648801598177, -110.90551031296536, -109.69205870504638, -109.8648503154861, -110.28183391384131, -109.65970942950766, -108.43615680946908, -111.11790511866548, -110.89043476451553, -113.64898442872548, -113.08004494963895, -110.81525412051718, -113.91009875719509, -110.95802128672312, -110.40944585634135, -110.33464695414992, -109.98984645778987, -110.18795067005652, -110.62364351231234, -110.44029833291248, -109.01598585569788, -110.95430216511514, -109.77987141110621, -108.54452361812068, -111.41780266439777, -110.47172771858405, -109.06084635984516, -109.30794593246578, -108.8764083815745, -108.18222749506985, -110.31330487887435, -109.04176821738014, -108.8558386035048, -109.47888284507395, -110.01459604573937, -110.48596659065309, -112.6781342298378, -109.85522803775775, -109.0569534499285, -109.08991286548698, -110.89485727880403, -109.18715778948663, -111.50381433568144, -111.3545424730884, -110.07710926239977, -111.99977850157067, -109.47444853853723, -109.81605328527645, -110.74995213151195, -112.56834665925544, -108.52052472391404, -110.89121213995557, -112.02004142355113, -108.66413739656008, -111.10053848695652, -110.41241079991636, -111.80152991764473, -110.21746151515111, -110.63265128607344, -109.483042128511, -112.78639954059729, -109.47114195846122, -109.23309637902875, -108.97133643967169, -110.08909147812822, -111.01105271457081, -111.18602432128249, -110.04633990216801, -109.53453538673071, -108.81939452082017, -111.13486114285661, -111.65877073200598, -111.63763706753498, -112.14107810664572, -113.6231865196724, -109.31743865878806, -109.18551713085722, -108.74951309653638, -109.28206426212142, -112.36687029711229, -110.10933061193728, -111.29501093502684, -108.19021080564794, -109.34497312126749, -110.37228033937312, -108.63277512903049, -110.61033993911002, -111.2975761598062, -111.49780004751436, -109.91019436685814, -109.32789992989028, -111.4482538110117, -110.1538439123475, -110.66347034043578, -110.05055133068794, -108.53002033538341, -111.7522199783972, -113.49108651193104, -108.03793940563418, -110.07108694011555, -110.83958739865201, -109.62805629409038, -112.69637731014087, -109.57996950503268, -110.104850643722, -108.83376203949506, -108.69400304840181, -110.59434352922563, -110.69121011800921, -110.18694553784364, -111.90598571547098, -110.30230802494223, -109.66810649416752, -112.6017099000434, -111.00296745333219, -110.64462650261785, -111.4775358707403, -111.98753241268494, -112.26574909791167, -112.04796822399412, -110.65853064447325, -109.6623218025264, -109.40559579075378, -110.42174451813142, -109.18991987957241, -111.02050178263048, -112.77950487440032, -110.42443751566815, -111.35440372400903, -108.5263524245987, -105.07498063939795, -107.15444425741984, -110.4508720018025, -110.25163264819463, -111.1383261104107, -109.91171620173931, -110.52200560606038, -110.5299174299573, -109.34628087255733, -110.26101817411786, -109.65071853372183, -109.66953335961068, -110.83590602054682, -110.980546313788, -109.4110066989163, -111.47223607390256, -110.00281523859483, -109.4088722967626, -109.00401922839337, -109.59655302543185, -109.7359970854586, -111.46016206343049, -110.23478747568004, -109.29441275295858, -109.82941912510167, -110.43088525283673, -108.21649744751299, -108.70220592702613, -105.2334473604296, -110.60620657984927, -107.97533820921146, -110.7664079806058, -110.56406610911355, -111.76465470250328, -108.84172809688911, -111.03661078143631, -109.85351980370237, -110.70091167176791, -109.52380717508088, -108.4356492672842, -112.25498760397127, -110.69648730540193, -110.36748838594507, -109.99090797924349, -111.2678642544111, -110.42541694325627, -111.4575545259775, -109.3211175669008, -112.7465573314208, -109.56208667784249, -111.59733497772172, -109.42295730962105, -108.55804089331346, -108.71397903286748, -110.09188290952392, -108.90810063278326, -110.31333217069538, -109.69794714542728, -109.06210020835357, -112.42465112160288, -111.74630553904855, -109.99304310093493, -108.93867687355595, -113.1669287525049, -109.09193568851137, -109.27500368450697, -108.99643325722404, -110.53962759110647, -111.2052088429852, -110.05855563908841, -110.30763723153481, -110.03411001268613, -109.6161415052669, -110.6304714466923, -110.17116005754627, -109.0753171640551, -110.92564270851628, -109.60831770517053, -110.25913363817017, -107.76644895378317, -109.2619309023068, -107.64198246311884, -107.37056168314048, -107.31978563121643, -107.68171928702894, -104.57515288104209, -104.75187637758803, -105.27246893266054, -106.96524396060869, -105.93920355631757, -103.66449995825586, -104.08476660009461, -104.53081578265315, -103.0148493379086, -106.74751670818362, -104.92309629919443, -103.98320340724693, -104.81633219413234, -105.77996356028235, -107.12559309216644, -107.28196039053535, -108.84583578337953, -109.4494696919565, -109.15525441177898, -109.7634811359225, -110.79433338587495, -108.44440079452527, -108.79597700117748, -109.98590735173822, -110.72144284267539, -109.30550753718086, -109.70072152916897, -109.65801130162137, -109.65949265997646, -109.82238573025273, -110.30669821947491, -109.83394128869384, -108.90433312205332, -110.664046708231, -110.39926453734134, -110.37725911098757, -112.12508639032839, -110.26795666332589, -108.98741993218054, -107.76168841100478, -109.82334992872889, -110.83516363498563, -112.60649745671253, -111.1960726449926, -111.03919163866381, -112.05129034965563, -108.83187987662883, -109.57240688505179, -109.32857861150738, -109.54934849013647, -108.29359879300195, -111.5179112931669, -109.52702486426027, -109.95429980789645, -110.7011078611564, -109.43204524997455, -105.56031249677113, -107.70609254346495, -108.78303653454363, -108.11457060956113, -110.44215460317537, -110.78267897406572, -110.33119812901934, -109.34449539666907, -108.82636558484161, -107.1834151347969, -108.83808254322192, -108.2542825327446, -108.80298057862501, -107.59922121598055, -108.9131916496929, -109.51519107961856, -107.7704986323755, -108.79678029009878, -111.13791068210752, -110.402746275919, -111.31702623823912, -108.49812727557243, -110.63723264798182, -109.32890666586829, -110.29721723278237, -111.66560929315017, -111.04227698307153, -111.36927505376269, -112.5203298417673, -109.93967930487354, -110.14533835678606, -110.3868348991775, -110.85413569165249, -108.44519725537315, -107.93391978795047, -109.82778679299085, -109.79311153223738, -109.25261055399044, -111.47738679135526, -111.11775495397512, -108.65898844492045, -110.26505495390529, -111.02017977446526, -110.34817965403467, -107.55161094495372, -110.21667403085983, -112.43970497917284, -110.70535338255132, -110.79438078890512, -109.81809822502822, -108.99167960596515, -106.5556893069368, -97.51736665041192, -105.29926513345109, -108.72453297392224, -108.23203912463346, -109.50324111400698, -110.9939986929772, -108.05367524487318, -108.37339392211176, -109.8553291283933, -110.46179639493138, -112.48795697163695, -111.88145079973545, -110.8678969738583, -110.62677605624849, -111.83824818603244, -109.76798658735359, -109.6654742351465, -112.58543522753767, -110.3406716250781, -109.55013159400883, -108.00481229232405, -109.90793236599207, -111.28597960985334, -110.54144527494444, -110.14704702870655, -111.2652554338908, -110.97520848958668, -108.63647576273343, -110.52472680617548, -113.16137826273847, -109.62457037485827, -109.53869420402964, -110.71399284283449, -108.55435337782664, -108.09492728294455, -112.2373886856363, -110.3693019226993, -111.65116752865308, -111.3223986412311, -109.67734725401074, -111.36420709226297, -109.14293108556625, -110.5982939020188, -110.29596476096043, -112.69847120697035, -108.39052787054206, -109.06205229490357, -110.00045399262885, -110.71775009467346, -110.69530760167493, -112.54144940754935, -109.55755373438097, -107.88943697845929, -109.98578587243783, -110.14202980613851, -110.80051915904802, -109.11327182471621, -109.50637030500913, -109.77023677605327, -109.98552825925917, -110.40235854896, -109.37603004890141, -111.36989177909379, -110.8399811877331, -109.30394670937987, -112.2769814990538, -109.10893172594731, -109.17733972841754, -108.35968166480572, -112.64492569586005, -110.13779257328873, -110.64439690778532, -108.45446935516622, -108.97325006911116, -110.54637968933774, -110.66412364132371, -111.38627695224784, -109.8942998516069, -110.36392017322382, -109.92355133054227, -109.61886697310419, -109.71969465343778, -109.85627196259388, -112.1407808286419, -111.1013489416651, -110.70428953307596, -109.3454280179969, -110.22984684615578, -109.53826801613613, -107.83673208330934, -108.72742563398342, -109.5745872123195, -108.83031823548816, -110.89059911076627, -109.87842545384129, -109.21980161063786, -109.07140273870678, -109.04628915564135, -108.79255665097845, -105.20875397856382, -110.0838008881032, -109.68293832806683, -111.24644641302518, -110.01257579497496, -110.99281477454484, -108.99296184719546, -110.96495665514604, -110.70404386182749, -108.25078498739035, -100.77667501455139, -107.61479263900088, -110.06600976399395, -110.02035637581871, -111.45524052052504, -109.975541184397, -111.07333860975358, -108.4808974233161, -109.59513524582242, -110.74711589861774, -109.50005300854993, -105.23071652566294, -111.81094849223531, -109.0168079712372, -111.89029991620679, -109.90672274216391, -109.30959446424889, -108.23718655264584, -110.10868108588909, -109.21139771899594, -110.33333323577992, -110.25792318324204, -110.67825932924109, -112.33148517950511, -108.9724848367048, -110.78371843797613, -111.40913868573313, -110.2930522718577, -111.9538408094371, -108.63639312641844, -112.4462941079034, -110.40266356498321, -108.66617580940074, -109.44306834729083, -111.08962916641603, -110.52132608161017, -110.53757698855654, -111.5587344449704, -109.77722315102946, -110.40060629757771, -109.45395807961631, -108.77558572395142, -109.0151938598724, -109.80739619986889, -108.9332873172888, -112.49933978358132, -111.28667321897437, -110.40629082858706, -109.9829216820938, -108.85102919990373, -110.84179127037925, -110.27309817549309, -109.88857884367955, -112.24517967927224, -110.23377125710859, -111.26951227953063, -110.09782138347559, -109.77508406986834, -110.55359722398646, -110.09534729906368, -109.96333904888587, -110.29372855476366, -111.36651812163072, -109.97141184588116, -110.16701683369045, -112.8562627359291, -110.66651146857079, -108.78873821095968, -108.59208174618087, -110.31784275318834, -109.43177042415276, -112.80272887161644, -111.79874205007107, -111.08216899537892, -110.73699224045636, -111.04738767291953, -110.43395896705012, -111.62106163510778, -111.32599933330843, -110.29360981749807, -109.66562228449096, -109.21316193790335, -110.06363162177448, -110.54480468587292, -109.31791670875509, -112.65386492377107, -109.91857609999171, -110.57233605624137, -110.7597333064856, -111.49767138733276, -109.36548654843229, -112.34145274183716, -110.52831153822652, -111.55802243871352, -111.81399803046556, -110.17680125962372, -111.23811621944807, -110.48042049674514, -112.43786993562033, -109.56507357271987, -110.67030752598993, -110.86377249100713, -109.06001892813467, -111.37023727930494, -109.52881096984436, -112.95107295160436, -110.49467818026214, -109.29804210589607, -109.89270706931751, -109.46354468058833, -112.10350702955014, -111.06083529077077, -110.49996587015904, -111.1617248913634, -108.84725633199014, -111.42852695852422, -110.01433866707184, -109.11616968390972, -110.76961079765468, -111.80403513904453, -109.84442686379181, -109.65447921666167, -111.3378640555306, -110.8882647652338, -112.58014202075226, -109.67128881545659, -111.73429980763389, -110.82258070774773, -110.71895931098041, -112.5117489008152, -109.16182299471309, -109.71651258790612, -109.7770618808562, -111.94294809571427, -111.1629115541574, -109.57489224865171, -109.8402445779754, -111.17931450307283, -110.09045865447595, -109.23658206733491, -112.54929616847242, -110.5150381158864, -111.32296447909377, -111.64472156295191, -111.65832771066007, -111.03359562742956, -110.85303206770837, -110.80655337650862, -109.3712696310075, -110.57313454785879, -111.18525355670417, -111.67423695430561, -112.00829831274282, -111.08915434609605, -110.3298290221436, -108.68552957386795, -112.11377370993225, -110.80288297661977, -110.33640536217185, -109.5907971201988, -107.9195263775506, -108.50223113159429, -111.91191347156142, -110.29585599512956, -109.50902788911351, -110.76819145749467, -108.86899533416589, -112.09963049260891, -110.13374376572433, -110.15881393584463, -110.87392107947531, -109.18658540731009, -109.72734703956934, -110.18732487568724, -108.76554115185057, -109.94122289815374, -110.39583285609643, -111.09540935727229, -110.6618176357367, -111.6281345666718, -109.69686483639367, -110.31633402076315, -110.61246951748903, -111.73300235294965, -111.34221378834899, -109.46708370903485, -110.70412671997354, -110.7007891485379, -110.31685483435038, -111.03016917417074, -110.94517365625376, -109.46580797053619, -111.20935248224806, -109.20661126636224, -109.50147037097533, -110.14241781654353, -109.8510950344643, -111.3794198224028, -111.28966889207122, -110.43347441663424, -109.86759980279523, -111.92101892013198, -109.31594011390644, -112.92253433794441, -110.74000829597605, -110.3690783911604, -111.9386136764295, -111.04196305034188, -110.41800427558245, -110.94287511448232, -111.66035388807579, -107.53723747644062, -110.68014818358719, -111.86628806511304, -110.12097497430523, -109.69880468221378, -111.4312783987915, -109.18240866486639, -111.45649839248873, -110.1242345454651, -113.75911576151633, -112.71747598882953, -110.9614554157337, -110.92294419716129, -110.87229098694876, -111.09943759113875, -109.48107247947176, -108.62783006742795, -110.8108025857779, -111.63342408317932, -112.0221522906341, -109.96411229549527, -111.29821085030613, -110.04566676239914, -108.41674583097112, -107.50256474992416, -108.68086611003493, -110.3738906060137, -108.86763212826641, -109.81681043446049, -111.04539822346567, -111.73290882980949, -109.75238769150758, -110.55268275367449, -110.48423701377924, -112.1116140908134, -109.53952175199518, -108.538611608547, -111.3788321484912, -110.36378736224961, -110.37712171023523, -109.82150687920334, -109.17046632238393, -105.1169578108227, -110.84067642540583, -112.91626789016587, -111.32030958133453, -108.93375913686056, -112.44450956563915, -111.1596840012794, -110.17380444915341, -109.634859036508, -110.68819277718731, -110.0648098825346, -108.87385575091399, -111.99676414571755, -111.32585405719519, -110.59892045991457, -110.32589048340424, -111.1172696292077, -109.79946399891651, -110.10030723919304, -110.71841081343656, -112.23013150012054, -108.94400401141407, -109.71044551701596, -111.77560214164039, -109.68779520039777, -110.96119601299907, -113.66477058855787, -110.17794649102234, -110.30159876509862, -110.11953836266514]}, ...(2 in all)]
  out "FFT 2":cluster{"f0":dbl, "df":dbl, "magnitude":dbl[]}[](graph)=[{"f0"=0.0, "df"=16.666666666666668, "magnitude"=[-324.19011195451765, -78.1272953812706, -85.85545438627958, -89.30587144190069, -92.90590394398903, -93.63083388385274, -91.8644929119412, -95.26924857401164, -97.0710469181336, -98.01148078956652, -99.33043660296804, -95.58776817681839, -99.9570097527269, -101.45494093095093, -101.51838334751548, -101.00386616525799, -103.01963069818913, -103.20223925731209, -103.53783076500916, -103.48065647812659, -103.97797518531912, -104.58942778240602, -104.46991277190502, -104.59813972158683, -104.56685024229951, -104.69893799348945, -105.05669000016238, -106.17061117835001, -106.43303821862656, -107.39468286383597, -106.2899368267905, -105.7863846168199, -105.17170638885071, -104.53818172761852, -106.70340956723133, -106.55444321137247, -106.67654843051936, -107.79888413750199, -107.86424326005849, -106.09722609215336, -107.71648639013972, -107.79500725395155, -106.17330953637067, -105.43663624517525, -108.04970689199158, -109.92106271611999, -106.2505251183406, -110.60221373795562, -107.11377887451098, -108.4126937286195, -108.37794745021417, -113.22457316369011, -106.38281814065472, -107.55385617652075, -108.93026538982782, -106.19334142366085, -108.90462602264525, -107.63084712174981, -109.12192537022624, -107.90627042480016, -109.44472079190832, -108.91731458372392, -105.74102972706788, -105.74407510394178, -107.5989477192235, -106.2838630137392, -107.46190542725505, -107.38881299750702, -109.08024783239452, -104.97871836903269, -106.65424712290651, -107.04966019632134, -106.16202578092883, -102.98374199247179, -99.1568704142098, -87.07383781389657, -96.41471411313154, -102.65176579899618, -107.65674867775193, -102.85397890306213, -107.58658613411464, -104.79044898833125, -106.65282019869865, -108.65027966345534, -109.46169054950127, -108.69969979291741, -110.4048706652988, -108.81020193837274, -109.42808902484134, -108.85398463561398, -108.3849716744813, -109.1844457168716, -109.32787859535676, -111.01992124870878, -106.64843449415699, -108.9926343573667, -111.59837822080355, -110.57121677672183, -111.17280164669164, -110.68901970586144, -111.69013245592781, -109.90200577018311, -109.3554172126163, -110.7515368822992, -109.2863324212524, -109.66209701262974, -108.50795548698007, -110.58126481096504, -112.36093896766921, -109.78612141282203, -108.85120530917233, -109.91424431080952, -109.84698632196245, -110.93960894966105, -109.77214706089354, -110.30762971422381, -108.77791302937449, -110.79522659679036, -108.47242514643455, -111.20629758187835, -109.05996769621125, -111.13574821570619, -107.79388178889101, -111.5768481279296, -110.52058839597171, -111.58729762739313, -108.99000864386126, -111.6585121505227, -110.50715371958135, -108.87151956974363, -110.30486244367107, -108.32392040018144, -108.1769507919999, -110.43198471512189, -109.81454097966842, -110.26717009815644, -110.82924135076777, -110.34103661156989, -110.0692667126265, -109.34555682020833, -109.1694484721415, -109.9940980324044, -110.81940616215803, -108.21162003366862, -107.97087538330561, -107.55312461506225, -110.60339321606872, -110.09004629292225, -109.05860430198882, -113.1412749514818, -109.81628200948371, -108.62343219429849, -109.48172424209761, -110.85978755785311, -109.47778611557064, -108.81728552967951, -107.47864241666747, -107.61735128422292, -109.62511618983821, -110.32417726356636, -108.24287897478176, -108.60460879530194, -110.2181558494026, -107.95550802888957, -110.80234484950323, -111.09955733353904, -109.43923052503506, -108.98949130235951, -110.05778199870154, -110.36224432927585, -108.13523430027999, -110.681114579241, -110.49106131529867, -108.73493328004297, -110.07663907252234, -109.9968931372618, -112.10715231091008, -108.80994125105168, -111.63774865669372, -111.54355694032755, -111.64024217585788, -109.34986300492378, -108.88053713185408, -111.14370830146245, -111.17327416167232, -110.36311492990576, -109.99414559884396, -112.96912007380595, -111.43191437097785, -111.71327312809349, -108.77202323682606, -110.25970374932486, -112.59574277180732, -109.77247894866957, -110.09219852365874, -111.7197662726775, -109.85454092697009, -110.06789440397942, -110.38055758638309, -111.04251386932805, -111.54279434240568, -109.74385329575985, -110.98924544863415, -111.17898077762852, -110.98364252730245, -110.75024385843372, -109.24766708578407, -109.67753987004863, -110.6537235844391, -111.84436313010086, -109.12654337292446, -109.65519521121124, -111.1845162935778, -110.5009101465602, -110.22980642268818, -110.88540043278346, -110.29249073109453, -108.80459864528464, -107.49372141121728, -108.50353962704821, -110.00730069533373, -112.012876492648, -109.01283702976382, -109.07442203290057, -108.2961442983685, -111.60962842680907, -108.84312815413224, -108.6276642979969, -108.75132871638827, -109.30004903844721, -107.20359872252604, -109.12175943862074, -110.43914247337625, -109.55954680842791, -110.37116786618797, -108.55907813251434, -110.19249995041955, -106.95269845697632, -111.07027929458712, -110.1073996792702, -110.61729280468039, -109.6419175310234, -109.47995019876329, -109.66602827275211, -110.01953864498805, -108.45989120418268, -109.79778555296474, -109.94663827736616, -109.52410616839379, -110.58014441463794, -110.09182359045897, -111.0487262011397, -110.49609187214915, -110.6114701312941, -111.17752423063314, -109.74965389041003, -108.58973724447526, -108.84292130035902, -108.90689510645983, -110.69840140049361, -111.30494362640982, -111.00224390075273, -110.50848328538423, -111.59232911931113, -109.30826761863756, -108.44510893127558, -109.63744704504391, -108.95037574307332, -111.36486409910674, -112.74508631930381, -111.03952454593811, -110.57133212903979, -110.59969855145111, -108.25570461975128, -110.44617635200193, -110.32190307214704, -110.95204704643322, -112.0595421753479, -110.45342552693265, -112.50183987758867, -110.08217804938009, -108.90353583389084, -107.02032313792242, -88.3334978919524, -107.92027625495886, -109.83148570028482, -110.30427997450572, -110.92855407802753, -109.67404674397338, -111.03606345823586, -110.58277018943096, -109.77692362669393, -109.39170901729935, -110.20711662408928, -109.41601946806779, -110.34213214925832, -111.2283900972803, -111.51682597931386, -110.47069117801351, -110.93808974285523, -111.11277478000933, -112.50698886748012, -112.12918507523611, -110.46316790252011, -109.9387334819968, -109.78723249688426, -107.13037722044297, -108.16132376075751, -109.07255491017162, -108.85068428558272, -110.28038153100799, -107.77611023481016, -110.69754506886444, -110.09495581837979, -109.21214884561816, -112.62718526248648, -109.22048725312992, -109.17793923163308, -110.87372121410577, -109.71902632604333, -112.61041177225496, -109.6374750969677, -110.74738952366951, -108.93404661877067, -109.84938675700889, -112.25316361679832, -110.30788094875312, -109.26929069321925, -111.20853536783942, -110.05212566057608, -111.72448131932816, -111.55474439772887, -111.81988954424324, -108.44452452934028, -109.21897824914645, -109.55634869894358, -111.36318572800242, -110.05777399011298, -109.64458567712875, -108.73315084760529, -108.93332091319675, -108.4816455312154, -108.80120578498936, -108.1804470361839, -109.7177707524778, -109.31977709844544, -109.33603116022124, -111.46120546572519, -111.7480378245176, -109.17907150677627, -110.47970652472505, -109.73718750984082, -109.7935026884937, -110.40458408612054, -110.91781389491092, -108.39352075861481, -108.27512197925346, -109.59155075404814, -110.40183121737397, -109.25423373270381, -108.37769008625712, -107.91335995938509, -109.5576520703013, -107.27392145737491, -110.98592762117059, -108.41809950647861, -111.48163889400448, -109.70961684769624, -109.22952568656495, -109.76504719131209, -108.86928627177666, -107.97855299877004, -109.8412204399902, -109.6690048999326, -112.28329030175193, -111.54977099314607, -109.55689540119126, -107.93716711232997, -109.84247640855929, -111.5098351445789, -109.14317615215809, -110.28319116384824, -110.57901069942578, -107.2890252845352, -109.66754569546274, -110.15708115946433, -108.83782190109405, -111.60783857760667, -111.46884385151185, -109.21985333366634, -109.63605494317056, -110.87999187262697, -112.26992029775087, -111.05491095860552, -109.22795442529183, -108.99135781712076, -110.46475190704264, -109.35746113713218, -109.29125989270668, -107.40922407684049, -109.24391685563656, -110.41554602144217, -110.68952735085914, -110.62457364102458, -110.39856310555466, -108.84256124354566, -110.01614601335088, -109.8071306678428, -110.2804500736802, -108.76205061238203, -110.3962440297242, -108.98253716257014, -109.32990745926702, -111.17276766165281, -110.41113652364085, -110.36616199963426, -112.09767002991742, -108.43599666470733, -110.91876588140981, -109.05329272502944, -107.07198690769708, -108.72934463903034, -108.6666471996132, -108.97529973794413, -109.68895260146817, -109.2658844652487, -109.75690097249196, -109.38585024123027, -110.17593039468063, -107.87223111061134, -108.15261097418302, -110.09277437980633, -110.8665497655964, -108.43061614348413, -110.3052458526819, -109.22446919161898, -110.51909692711594, -110.06620699121913, -109.53439413051383, -110.31952463872884, -111.4732125902982, -110.41443606663168, -109.9579358088152, -109.930778061577, -108.5473214465574, -109.34719220288939, -109.16964653934396, -110.04824158176345, -109.42616539603762, -108.3556027482992, -110.62331917617789, -111.3652147859356, -110.12362012120938, -110.13175448595814, -111.20110099151856, -111.50643914621541, -108.11659117128028, -111.06037600347967, -109.03822892917451, -108.25678204604324, -110.82608024151122, -109.15887945314851, -109.88255674562845, -111.18322672526185, -110.95836040044516, -107.91535345885436, -110.66285812468733, -109.61906549925033, -109.58059721670746, -109.65198009505977, -109.65950565672951, -108.95264505276342, -109.23343669003113, -110.74308548011575, -106.39170014998685, -109.61471203101753, -108.24258770956924, -109.84609566640096, -107.83834185503922, -108.93052854090027, -107.55568820082641, -109.758551082242, -110.65892780872205, -111.99907420485852, -110.71043004141137, -110.62257237494617, -109.15610413532767, -106.87403836327807, -108.19175324576331, -110.27819583792918, -110.23918003777561, -108.29703377268754, -110.07182881114713, -109.60256111108491, -111.00394752430006, -110.30750337485472, -108.78309624082331, -109.24103013025798, -108.76979253891403, -109.91618737478264, -108.83915940855513, -110.92536150834754, -109.72250903746432, -108.96533939688658, -111.08949280651164, -109.20335070860871, -109.37826578362439, -109.77953166722301, -110.1867310744785, -110.07114559821346, -110.7003631567182, -107.86455899696074, -108.94113264174617, -109.35999427135138, -109.33627364788704, -108.96588828808375, -109.08716536982254, -108.73575375369026, -109.47770132070654, -109.83726171472907, -110.73516506891792, -110.56827134787686, -107.65667508354096, -109.30200115708924, -109.28406803847896, -110.55374624323233, -111.2017766725333, -108.50851279608973, -109.79494403619485, -109.08320018013063, -110.21850624918747, -108.4652936555984, -108.74837610538873, -108.81326140648238, -108.83830180036702, -108.785270477003, -110.01845876259073, -108.76030368637825, -108.57879884880157, -110.6610608456059, -108.74669367794318, -111.55956030460833, -110.22906685783455, -110.48411613865359, -109.48060880085136, -112.77556331479562, -108.2676071206087, -108.8571136162698, -108.56944905160177, -109.16406757131058, -111.42259299295839, -108.25216316582294, -110.48487127684025, -109.69532331373831, -108.13992755196784, -109.2987762526628, -109.82536192480795, -111.28650061088359, -109.12820736404241, -109.37960655471406, -108.96014976926716, -107.97535047619023, -112.31953123574708, -109.06198330523004, -107.52722515967098, -107.31555373665437, -99.89671790804692, -107.44442600896275, -110.6549218761941, -108.02265794322076, -109.63582761762919, -110.00574746987859, -109.51565124961209, -109.3550083591902, -110.4541529175301, -107.85799722437162, -105.1197113090786, -110.25038075579738, -110.39710812865657, -109.3618876098789, -107.6131301952152, -109.21529527621463, -108.7995754403799, -108.48347353145697, -106.45678488065816, -109.60427918561142, -110.81194387812535, -109.52215044127382, -109.88751598659705, -109.30205143590227, -110.74984456751768, -109.03952092986351, -110.69170786328897, -110.39236248162467, -108.65456161733339, -107.60439764386904, -109.97367926606955, -110.2754359970249, -108.81546418006434, -106.99691398176165, -108.42047325825182, -107.24499915944605, -109.28116135603187, -108.70650358781573, -108.05516916105047, -107.20893100196241, -112.07029265690055, -109.38099990478445, -111.53461820465232, -108.11312509555277, -108.76714028655223, -109.89565008459624, -107.71879172001115, -108.08434857420214, -108.79142773619792, -107.25153085963885, -110.05595039449301, -109.31604222314259, -109.94405791565286, -109.04715370361387, -108.89278831045846, -108.84682466376424, -110.0067927716526, -107.63768959294084, -108.98109382020348, -111.4720219575084, -110.76023788797733, -108.78599647633777, -106.59726674064618, -108.66715709719243, -107.99134359630926, -110.11396713841884, -107.21091759882775, -108.08576824949941, -108.80217666857972, -111.72949572713338, -107.33126296136014, -107.33731660097102, -108.04470462977443, -109.42963925921418, -111.03517778720736, -109.55293581015796, -107.99948151285162, -106.59480934999681, -107.63777243313498, -108.96490626068824, -108.8948210299064, -108.30870516747477, -109.13612869658097, -109.59971429402015, -110.2571461001396, -108.7655464686992, -109.81144209568883, -109.80796806645141, -109.20948481699544, -108.68653880881129, -109.26329796696166, -109.22428132233863, -110.12571678351438, -109.14615461144786, -107.08261621308327, -109.11338327144382, -107.75421565039201, -107.45291780756361, -109.00477000647248, -107.41031480478154, -109.98948062864928, -107.45953654921264, -106.37522884807879, -107.7786128523167, -108.03610987358499, -108.05926797128022, -108.59400205554164, -109.89620453365603, -109.03811240487515, -109.96909236705363, -109.28212981785472, -109.6772152101994, -108.26493868190678, -110.55558039199732, -106.6252818398841, -110.19075011176416, -109.56520012524705, -109.8023423576176, -111.2697570480663, -108.26752571816566, -112.00337375484828, -109.85709226796116, -109.36922081321148, -108.8424844298318, -111.2512302139209, -110.61775974680471, -110.22501328999012, -107.76874906708105, -110.71023653476604, -109.4025656165291, -107.66667684986125, -107.59759854092948, -107.94763263251238, -107.3888591871119, -108.62692803125044, -109.18012867988286, -107.78662871481455, -108.5072814073944, -109.50348958982907, -109.95177634938378, -107.78756251182895, -108.03865042797304, -110.1814993556385, -109.34937567548833, -109.52162025123161, -109.50819015441117, -108.20953105254624, -110.52154040214435, -109.3324404469266, -109.2696617050831, -109.54675609195674, -108.5940367000989, -109.40184828664549, -108.2518305610941, -108.55972691669434, -109.03647225394408, -108.48166656251695, -107.42023429066523, -109.42453054302521, -110.09532345960083, -108.78315822119662, -109.97508586102265, -108.22687406536997, -109.17110028890058, -110.15390449992647, -107.88577458651508, -108.28851074361447, -108.52030295163331, -110.03496861709483, -109.40014319167584, -107.73048113044877, -108.17571683963915, -110.34839852994926, -108.55894048192191, -108.74107339998285, -111.17734138993401, -110.22946440841412, -109.45511941802884, -108.0657300641843, -109.33797363184166, -106.95974095511333, -107.93068343723691, -109.78867669512647, -107.2087297624043, -109.542665021243, -110.05035859052961, -110.30235238883523, -109.20586170783808, -109.2796396673401, -109.14260673746566, -108.22019460542734, -109.99011886871159, -109.89103038547285, -110.36964772493243, -108.62340319923602, -109.06779821699769, -109.21830861066148, -107.7402395759509, -107.7178850938205, -113.45665085929117, -109.24039191621704, -109.30387033426037, -107.61849760982835, -109.41430582703529, -109.11482836392241, -111.89328423764577, -111.84653367963301, -109.00674896486915, -109.84488648739638, -109.41914760797953, -108.53442910169935, -109.66883322968232, -107.68762956301386, -109.82583101109167, -107.83405397804887, -108.78052031141966, -107.37842078941692, -105.40843158543845, -108.81430898189338, -109.57374640194516, -109.41111270322058, -108.82621700188898, -110.2552502368822, -110.23903890097205, -110.52171662278697, -108.21249857906324, -109.97268479379733, -108.20088823960992, -108.85682002802234, -110.11642849164285, -109.94087886999255, -111.63180946270296, -108.20899499456195, -106.73341567332112, -109.90003508676807, -110.14688274481229, -109.62259307329889, -107.57811196819495, -106.88584597822792, -109.16132624528932, -109.78677836397806, -108.59319344451784, -108.55877448618652, -109.46883711353044, -108.47309455543844, -108.09487065732198, -109.82219079158135, -109.63780237877428, -109.28348848877269, -107.62893405379826, -109.46986737961593, -108.03089712610223, -110.3931917410696, -106.06970126043262, -109.41866550703786, -105.31710372440419, -109.20218082282653, -108.28467118008108, -108.80026326744611, -107.40729224715713, -111.07322915141532, -107.1057186510818, -107.98286374205958, -108.51298722989311, -108.69632670891366, -107.96509231988331, -108.15882223414738, -106.85862416470376, -109.70705792539056, -108.64519930633055, -106.78708421443504, -109.43552377900174, -109.4474526498122, -109.10135248755788, -111.43316642580763, -109.33457343739448, -110.23547887071898, -108.95690647379442, -109.21159903769149, -108.12969562680841, -110.82751409340537, -108.55724349027832, -109.8796329603075, -108.50369978374582, -107.43145467247209, -108.60003323209516, -108.77155705999647, -109.33806063660796, -108.37500858898439, -109.65641721611547, -109.81905873737344, -108.03483220769625, -110.48028107566635, -108.60527372219985, -109.28768201151478, -99.8804125587218, -108.8913334544964, -108.23534920737794, -111.07646463287153, -108.59029790589766, -110.3405916586831, -107.66387718565608, -108.73793152614131, -110.61440166477816, -108.76211382544581, -110.23236978486065, -109.10669297094852, -109.15247609779597, -109.00539004923506, -110.14424353412238, -110.55445060661157, -109.48721312920799, -108.17040942305823, -108.77592227268228, -108.77130256578067, -107.82494496098512, -109.57266989523707, -108.75767497229612, -108.13688624150026, -107.8280716764963, -105.676279602552, -107.6370316684844, -109.73508547021689, -109.25365178573009, -108.86767843317584, -109.70969944273735, -108.91917504090888, -109.97734866522867, -112.17308993943783, -110.28356299479682, -110.7927103729386, -110.30837645846702, -107.56364161860179, -109.50188349731121, -109.36065627483853, -109.75389877587511, -109.81713476007774, -108.14524057525358, -109.43832376796216, -110.89342891210596, -108.15657882822792, -106.84106061627887, -107.83091759905821, -108.61794662682962, -109.57142366843581, -109.85402645528154, -110.12877022469837, -109.19414429724044, -110.56168468006764, -108.74720588273881, -107.90448559921305, -108.54421401507743, -105.06700039841249, -109.17937358052484, -108.94317576365822, -107.79410219455083, -109.24955437598658, -108.23334395173994, -108.98759227946937, -107.05986359444529, -107.20956512998849, -109.00295831471958, -109.43119556916457, -108.93348410522628, -108.99932477701081, -106.6448790859128, -109.06877251308666, -107.67053918439544, -109.15052780608639, -110.16878033319385, -106.55101141640301, -108.02811045752685, -111.52173447126572, -110.16854119242062, -110.93164036911654, -111.25979320890855, -108.82629030379024, -108.52004501839738, -107.09697056562636, -108.94233383169858, -107.37962568194772, -109.1239201710643, -108.93949898577122, -110.62573772949195, -110.09592372075662, -107.56136391005947, -110.45600430869621, -108.79481000016084, -109.41462449554598, -109.30248158488335, -108.70735295493108, -109.9174743694956, -109.94232543385962, -110.71725446170196, -110.0346196158573, -110.34814317845934, -110.6651078322521, -107.55409880424479, -108.71734776861287, -109.50902203986271, -110.40207542979611, -108.7847687630861, -111.10599488129682, -109.30824728923263, -108.20134064331717, -110.55959112431609, -107.77099734327174, -110.23862843385446, -108.48520797666865, -108.54205896654946, -107.79288769037599, -109.84022250170581, -108.02758364115576, -109.35132492327935, -108.87009749667932, -109.86905123364855, -109.19826752168308, -106.835240323691, -109.37910022114056, -110.80633973102931, -109.12703823829597, -111.07432699570984, -111.8064506085314, -110.09349947650527, -108.66467295777367, -108.75119108236053, -112.63983351316729, -110.90940743670113, -110.27973159222081, -109.57141664526549, -108.61645363771719, -109.31742355616147, -109.5839599160637, -110.01188998365383, -110.01923429741011, -108.94779759137936, -108.26169431000017, -109.24553201026085, -109.95709526422822, -110.68677343596859, -108.7678734483002, -110.47090469179284, -110.31604700116512, -110.10256600741997, -109.76634647265719, -110.8830805828562, -109.94609564072982, -109.20662382740542, -108.12492970530919, -110.5274435478767, -108.02351960398035, -110.6264936805739, -107.14559226383577, -109.13821777857531, -111.05324489472586, -110.15190797512811, -107.96366234783144, -110.03950681967147, -109.17476300510336, -110.41251816187909, -111.39219865477246, -111.32530426869943, -109.97369363558423, -108.98666403063845, -109.62049358645565, -109.58130494498671, -111.72738873188874, -110.39825891106616, -108.57430325757545, -111.28625510212446, -108.77421250595326, -109.75025415031793, -109.51948456745635, -108.82129398637998, -109.81362137198361, -107.86292494316123, -107.49318292857053, -109.66948564589373, -109.54288390056654, -107.99912445612077, -110.3497559614379, -108.00549349666127, -110.01361420523357, -108.4977916421456, -109.67078387286976, -109.85678367732866, -112.01237658746248, -108.4855625950998, -110.84880875737286, -110.9178674382154, -110.44187536727453, -108.75076921971127, -110.04946286646651, -109.99780941000827, -110.14242932305507, -109.56343773672316, -109.6278993388131, -108.77419573790174, -109.10543670530926, -109.7801848627463, -110.30733124104881, -113.13440550301436, -109.32709134514755, -109.74136656933283, -110.01525283266193, -109.43924662938396, -110.25325289253, -107.75460576671303, -110.60057027395933, -110.71458404922404, -110.15788509050662, -110.69167485018224, -110.96006652476157, -111.01156633983031, -111.6058448010008, -109.51364005052672, -109.76058205940885, -108.43421621088261, -109.47973949170208, -109.25533250208288, -109.47422603921065, -111.36411644613841, -107.27566171102698, -110.45098686173688, -109.93589296291184, -109.03803734663714, -110.53118128434016, -110.2408872254969, -110.0532234862915, -109.94185495614619, -110.2662004220774, -109.51094016962288, -108.5210104215432, -108.13691752270934, -110.18460088390265, -108.32609309150783, -109.89652230508281, -109.80923900768477, -109.01917388968883, -110.01248300968739, -109.43415605440147, -108.09823485138017, -107.40637725320931, -109.40632232658412, -111.97981999127656, -111.16609811629485, -111.64500793960192, -110.99793748693381, -109.55531276386903, -110.2535662621666, -108.17429802469516, -109.09425673355422, -110.23187110421917, -110.55358397926925, -109.93461124753053, -109.55604345832225, -109.44569510408274, -109.72185151080762, -109.52963702944834, -109.2303630328152, -109.74819502244243, -109.3932530349457, -109.17096788339686, -110.46153727064616, -113.1073731246639, -109.43753070459397, -108.13332547768168, -109.42294574929969, -108.45798401969856, -110.29453435046327, -112.66249403705643, -108.78314667434937, -105.9634478773668, -109.14327524669528, -108.50645190860273, -100.81571594994128, -104.4482859840643, -110.68926237051092, -109.12362553230196, -109.45234390564677, -107.91461416156068, -110.67788819353727, -110.05744935668449, -111.78333392154664, -106.83628914455993, -110.11115457346548, -109.13434608275826, -110.80006861194663, -110.35323502651462, -112.29149906501372, -109.01656376530778, -109.30871662948859, -109.79736315392456, -109.17848983603582, -108.09752397056482, -111.6039030763455, -109.27008844877828, -110.84475733314184, -109.72393917557073, -111.31060762894991, -110.78858793807466, -107.12841545099752, -109.54510865218204, -105.2805426080281, -106.28514149354733, -109.50656759582803, -110.14700878401054, -110.49737016725709, -109.19811547071924, -109.92527399676051, -110.7961615015146, -109.7447227818197, -109.49432012009893, -108.714081576733, -110.09766801550917, -109.08448507943001, -110.36154838733857, -109.86328656267403, -109.21144237434696, -112.4145136888034, -108.57567151011159, -109.66748589540896, -109.72985837578446, -109.29989238126763, -109.85868902806475, -111.01778182304162, -111.23625326328558, -110.01270868104203, -109.27067928081415, -109.71171312410247, -109.28697459293629, -110.67868067201007, -110.91353786857455, -111.21479955051575, -109.11315965407708, -109.40418681804496, -107.80511819596003, -107.37201025889816, -111.81969609169838, -109.89875624306032, -110.29328043898657, -109.74853280072202, -111.39527865400605, -109.47746221101964, -111.75141177452517, -109.31325306583483, -109.30117448911659, -109.3997781364162, -109.45356931295724, -109.60585285774386, -111.33951689512735, -107.74187210470228, -109.62706021606415, -108.72139655505221, -109.79552836110567, -110.64354037499807, -110.96138240913136, -110.02215059889615, -110.92978442698893, -110.0620778287114, -110.85019647293322, -111.77397403227091, -109.81257196800128, -109.15643451383403, -110.72777566469594, -108.7463769025616, -109.80959395914073, -111.24500986151126, -110.48863498350322, -110.30863780110901, -109.79331354195703, -110.34087081762074, -109.45183222569266, -109.6440990067103, -111.15034876658994, -112.14912485578341, -111.8886180186196, -110.57054820211916, -111.07556239924551, -110.5872832735073, -110.28912501038172, -108.91501133754849, -111.44575118962761, -109.90799859177967, -109.74421995550023, -108.70941446115883, -110.28822893097275, -109.70039554000401, -110.33701797570251, -110.79445894683306, -109.57694314608153, -108.816904416038, -109.66517126767175, -109.39501469321644, -110.85775022889956, -109.3689402795614, -112.09107318723095, -110.67985626248422, -110.32971146814747, -112.08166943494875, -109.93955548712543, -109.31722953035252, -110.2062913031861, -108.22565380081006, -110.680898028151, -111.95386604441454, -110.83354130587097, -108.5873626748948, -111.97536144124408, -109.23944159551515, -111.57859477689586, -110.80135186615524, -110.4800953731021, -110.14040729648133, -109.25873050390551, -108.87000960474569, -110.97091597211167, -110.15787270199012, -111.62434537618091, -108.5421625277294, -110.42258666403919, -110.96896115868603, -108.98253068925274, -109.54245055160168, -110.28051096122468, -109.48060498658319, -109.77618362117276, -111.64513838754992, -111.13945484239875, -110.18094280356001, -110.43757222770748, -110.81588360154201, -110.11656805555333, -108.47936291282355, -109.16476249859961, -109.3549985917136, -110.77753190334253, -111.46065694661178, -110.40387985996301, -109.95673803226478, -111.58660981285446, -108.59894875229345, -109.37333363882607, -110.26849699991793, -109.30500469266264, -109.23789020998296, -110.82000706486865, -109.25927538839868, -111.03285659417519, -111.08899832832414, -110.69361682858042, -109.45187168573815, -109.9614018482838, -109.70209527974106, -112.11903952100165, -109.59713611623246, -110.70292028698111, -110.12743849746808, -110.63315585514292, -108.60450276298175, -109.32832664986026, -109.99753023477764, -109.46644696130294, -109.1781290160558, -111.58830180575129, -111.67229040267557, -111.3750024136205, -108.33616679452298, -109.99797067800029, -110.50892429124391, -108.66074740829372, -111.17094662568759, -109.87538933985836, -109.152526628291, -110.44623159817101, -110.21603106403009, -110.64376935639365, -109.36897426842583, -108.67303022227141, -109.89327693080823, -111.50442955563923, -111.37532237834381, -109.38132821290205, -109.73509680539144, -110.53918379735906, -111.22869870340647, -109.39977573957616, -110.3674665334106, -110.5366125953241, -109.99025356764304, -109.97300035646616, -109.87631077033762, -109.64608829594286, -113.02486102973394, -108.26250283140733, -109.62234918138763, -111.18766216512655, -110.33666026406992, -110.5808115327039, -108.2971671321189, -110.10964334161903, -110.61254021379767, -109.89852549557533, -110.16562049054073, -109.41433790018287, -111.2453823439446, -110.45554802599901, -113.11454453784393, -110.7333866145056, -110.00858191882439, -108.54745315874294, -110.08430415376903, -111.9006972727596, -110.3031506154679, -110.26331790366497, -109.36797925566673, -109.04860552478912, -111.83514212681175, -111.38960737633833, -109.01429665187288, -110.96404839103826, -108.95488871107163, -109.09652004914592, -111.884304581971, -110.57566691021339, -111.95113404442795, -110.13677174050159, -108.10078686353354, -107.69442565416006, -112.42676605669463, -109.12681161784135, -109.23120766087519, -110.57649395555585, -110.22143082743162, -108.40065951773644, -109.46923168308618, -111.39095086729745, -110.46375658526013, -111.45145283328486, -112.22610823637353, -110.61090190564383, -112.22250292674809, -111.7379343196361, -110.18530386733481, -108.93867365671692, -111.89304844956082, -109.06146134986984, -110.98405731832798, -109.76366821333497, -108.08326795663608, -109.95041147835065, -112.94140614324155, -111.79814935135965, -108.07337559063119, -109.13733403265212, -111.74906646037496, -111.12228668433455, -110.02899450462209, -110.22237716929811, -109.0224776891049, -110.18135850497721, -113.32516073881047, -111.3576490243877, -110.60510094465171, -109.6935518470342, -110.36313473154901, -111.95933240129618, -109.49625308071019, -109.18827910216122, -110.54311407822692, -108.4811035913567, -112.81280225723607, -108.86530665787413, -110.85796435061886, -110.40059714639627, -108.19250716343407, -108.96956521802292, -108.61281798886506, -109.78061525370413, -111.58885511891798, -109.06279169160345, -111.43043988466789, -111.63169336321079, -109.54702536206447, -109.62860636296405, -109.47865811135546, -108.02265793654806, -109.97461304995515, -110.72549884050886, -111.57309413919933, -110.03317891949746, -110.39570411598524, -110.27606115470397, -110.63294457306095, -110.71821689302902, -110.38076268941819, -111.51223508887897, -110.40703572670697, -112.24933273737743, -109.74954300082398, -108.46020292937696, -111.05315219575881, -110.38635148390118, -109.58268303790976, -112.34211536832117, -108.45894118755307, -108.96463982695337, -110.56040438523046, -110.67803313671729, -111.07349872375121, -110.42184162876096, -111.82081126435692, -108.85923651136297, -112.57723799596502, -113.65690874668172, -112.62314325834605, -110.70357529341362, -110.959925221544, -111.26336183001875, -108.1350700630152, -107.94545932312926, -111.17610778209841, -110.20386728310686, -108.55646511121591, -109.8400922569145, -111.73466587035968, -110.47272877573613, -108.33011124048193, -107.93042857580332, -108.60928277989103, -109.25240966798974, -108.96403833602028, -106.94222615757475, -109.37086694261907, -106.72743097285155, -109.03160193412796, -107.3549903889451, -106.8543848510082, -107.83503929060929, -106.30745467433752, -108.36915807168845, -107.13065938379303, -107.84769200880969, -106.08004345082777, -108.15244601930225, -108.37254117816573, -106.57863034819223, -108.1283698227614, -108.19776505569902, -107.58283412238643, -108.17365133196301, -108.6794309781181, -107.91552140588759, -111.60122989270022, -107.04360635941174, -111.55535949001795, -109.39870426166594, -109.55937904851662, -111.81389508925734, -109.88957041098786, -110.84764586896561, -110.59130246272693, -111.15944135223884, -110.19496154041607, -111.51861903129362, -110.74798816525838, -111.37312965175558, -110.10842817220238, -110.73198099204856, -111.36708667993291, -110.30840247819665, -110.11744489669044, -110.55237850846444, -108.2073528237766, -112.70750856801911, -110.99917956040802, -109.84949484779976, -111.3403161887679, -110.08924435263565, -110.17749213365616, -112.10849123224503, -110.94270741299202, -109.29350963424746, -110.33477486966507, -112.19620157705627, -111.45484078395934, -111.86858843505124, -110.22491147345858, -108.96177661263177, -108.67862820579893, -107.55155410582937, -108.27984439169573, -108.72682528077233, -110.64231212183269, -109.32873093119183, -112.98564364754564, -110.78933114228725, -108.50921025910479, -107.91087245586935, -112.57350030929283, -111.75871577457525, -108.42095298945462, -112.31266064114303, -110.1295657579673, -109.67444664474456, -110.33749884929306, -109.16098218724147, -109.63554874360221, -109.15892392675141, -111.90580809179818, -108.81196712336858, -111.42223552606656, -109.90571484965518, -109.99739812086352, -111.64103850263211, -111.31463957090885, -110.61247447444549, -110.20960333715526, -110.1707327818923, -109.70412636554525, -110.97278093107532, -110.24386747740314, -109.81378546061525, -110.83784085086458, -109.77357954318757, -111.22663832948885, -111.14563050139252, -110.87152231402447, -110.34246044319893, -109.97174570657546, -110.23599592972218, -111.08206161770731, -110.0073315341242, -111.11748366902188, -112.04005964728601, -109.81290191679287, -109.68543639040858, -112.01143296194752, -110.13641850530031, -108.19348942447623, -109.7534468948808, -109.36697824644176, -97.56454580435337, -104.97829040517887, -108.1539132982256, -110.048991273122, -107.46172505860011, -110.49269280640675, -109.94209901400029, -109.38576869679022, -111.43699124347364, -110.89973083498887, -111.2994445418276, -109.25144782032437, -113.25676258473536, -110.82078737428088, -109.97779571182073, -113.36294799183014, -111.38584551238931, -112.17267897274873, -108.56430946159155, -112.06841286528645, -110.36822473102735, -109.54758527532016, -110.48190506674653, -110.03535695860182, -109.3951469796576, -112.41910682256774, -111.38124138857238, -109.37850389100952, -111.65544568836181, -111.55876881606889, -109.3029209617236, -109.20030046194076, -108.82610577621037, -110.53329453526098, -109.96090595542142, -109.67834229432077, -110.62303603007352, -109.8388817181171, -109.22430039793213, -108.92749786663613, -110.05794249283548, -109.58534943218437, -110.50493887507297, -109.96373022997366, -111.0645036323456, -111.28501675364454, -109.77386932343008, -108.8952247140968, -110.09242801628717, -112.90943444063141, -110.72299296247249, -109.39094335967056, -110.95165384057718, -109.59809519359453, -110.4978602309597, -109.67109981692639, -111.2489619905986, -110.0937750887109, -109.76771021128954, -108.32976315018955, -111.3058145792439, -111.09464974601362, -110.99797900696136, -109.174315000222, -109.630351559617, -110.26289147175856, -110.22688407202517, -109.96748050100612, -112.13247633583758, -110.59994952890855, -110.93023020153811, -109.22457750926695, -110.26162558926984, -110.09713110375579, -111.73858994918328, -109.78183160058515, -109.7603471824367, -110.96016892586911, -111.23309626937036, -109.83093663960678, -114.05354944347246, -111.58202863059464, -110.42281828744524, -110.9521484732059, -112.5120328206343, -111.614891937737, -109.84428787405484, -111.61119567831453, -110.43095563229411, -111.71833448430398, -110.01132196809407, -109.37558169247951, -109.14091380022785, -110.42663661754088, -110.3598013572826, -109.78207135281417, -109.94058843992468, -109.88210328447205, -108.6217811850147, -107.17834387173707, -110.6447226986756, -111.10704778101115, -111.24396771977769, -110.47849395539598, -110.75150631628034, -109.67662689396347, -109.23145032835053, -108.83780193265358, -109.43468321661163, -102.22521103859944, -106.90009867479111, -108.91580608784525, -109.58671397003187, -110.56692028436989, -108.75103142680105, -111.00795573084157, -110.75039085328763, -109.48222099288613, -111.8621134816908, -110.26507966786443, -108.885924716389, -109.30841399453053, -112.3188631425597, -111.05677697153163, -108.8268571902449, -109.63028152237679, -114.82339015806369, -107.03435216376964, -111.34847692589166, -109.61354114874855, -112.32687758049907, -109.59816404231358, -111.64248480241805, -111.84075757907273, -110.44017657636552, -110.15181635726277, -111.93813663582833, -109.11826378836209, -109.99779889778326, -109.927119030584, -109.4389650887841, -111.52448814187727, -111.38736268499642, -110.51920914917922, -108.64230614681055, -108.90307263595304, -110.57246891832371, -109.65575340646116, -109.80359672370373, -108.83368585528197, -111.09385004343437, -108.83430005497769, -112.37784208819113, -109.50005381621696, -109.67421750136593, -111.39664088797532, -109.70867599669316, -109.52498993629875, -111.12341349673187, -110.0484037026941, -109.55138667646308, -111.06614422098669, -109.4785941493091, -110.25724082617013, -110.93950616855716, -110.53487953881397, -111.45722057988401, -110.32393446412904, -110.34361936710438, -108.6610336097813, -109.53631603696368, -108.06930707969195, -107.68056561368934, -108.73860971027449, -108.87111384617579, -108.40433837098611, -110.55999576884835, -106.83832061167207, -108.28786975902513, -109.18482905697472, -107.81071696594883, -107.91047268802457, -108.79613111673706, -111.05361322310213, -109.97897453479862, -109.12920563729425, -111.20538391490288, -109.26286135293664, -111.31400407177502, -109.92167984752287, -110.70854322826071, -108.59406515713611, -109.69371333227458, -109.36664873267313, -110.35521729513704, -110.40667924006368, -112.0181844636846, -111.01529188207431, -110.59246505728431, -109.95068312717868, -110.75807466894047, -109.58596443762707, -111.12127793384956, -109.59041634463125, -111.56255571372793, -110.43405578864342, -108.39660324329928, -111.1420710307505, -113.64788483868595, -111.67645688353934, -111.36878760365944, -109.68523694561108, -110.11608766310304, -109.25670490330123, -110.73546181099229, -111.77855039399805, -107.9662794718261, -109.67483334602832, -109.891258579519, -110.24757768183042, -109.50202895993814, -110.07763831916637, -109.96891925839451, -110.97268925927641, -109.31698133827767, -112.27933593506792, -110.36206721075725, -109.47379463718867, -110.27836850941338, -110.63738280998388, -111.3611682777485, -110.72689155959884, -111.55480904927032, -111.16689658479412, -110.35555645743601, -111.56609319131051, -110.88279459952174, -114.73607246523177, -109.95813757295693, -107.64639932425493, -111.26486783320321, -112.03946356928121, -111.8915972448334, -110.35245920812773, -110.83155104803564, -110.67437747473863, -110.9959682920065, -110.7815352345103, -111.13722283763049, -112.54797265493127, -110.06894780898469, -111.65186554925783, -111.83545188116254, -110.65894756123697, -108.48458025065264, -112.43760714427981, -114.1368408201927, -110.40065777895025, -110.1066998945526, -108.60654239598591, -110.5716060205154, -110.74257357180736, -111.1136089342442, -111.53539811075092, -113.2559601458872, -109.2003227548348, -110.42285840441025, -111.4086884998834, -111.61503050693868, -110.8194303494779, -108.9701587059964, -112.58521089509063, -110.10873915265242, -112.43440038319561, -110.03468788439882, -111.57896603236308, -110.21939233582523, -109.03614470500777, -110.11738923539659, -109.55359574898291, -110.416473622654, -109.4626868574157, -111.17164025076731, -110.3579689035081, -109.04338716157822, -112.36157114517567, -109.32125615922843, -112.71105693789394, -110.11019129547768, -108.96439402555632, -111.107663418839, -111.48306369859839, -110.9317530461794, -107.98628540532181, -111.1636972328743, -110.47837837583148, -109.04649309175733, -110.27110334963734, -111.35803630614352, -110.77259078859605, -111.46352820533895, -111.16789261049541, -109.2376344776325, -111.6795794983659, -111.74292205167644, -109.40835022991612, -111.02163652600731, -108.79482078001607, -110.6718658416566, -111.08747067599332, -112.15383726791498, -109.47049126158717, -109.061574046483, -111.23993049318979, -111.02521156588335, -109.46012868444186, -110.13918914826291, -112.08180381836377, -110.61929875223015, -111.4424805369965, -111.43420275069585, -109.71347556238717, -110.24726273025648, -109.7860268673935, -109.94126895018422, -111.41948668868926, -108.90555991781676, -110.81242861886172, -109.65007052722677, -112.12672329335953, -110.01123170946096, -111.13980448279096, -113.92013682657084, -108.6000853867411, -110.66793592761913, -110.61237681642844, -110.00839105230496, -109.38083187034974, -109.46119372195675, -110.3708067287448, -108.55518656223285, -113.33935987443276, -111.92184778392033, -111.80820718236087, -107.36852757311246, -109.51077803361602, -110.066791721019, -108.756710558672, -107.91391289865918, -110.72851430959301, -111.39074956442978, -112.928843679455, -109.87348280521556, -112.21371750380071, -110.82495902297394, -109.94006136010094, -110.58757785050143, -110.2790091349881, -111.43884888223081, -108.09540986530712, -109.63783244641691, -110.19577975613292, -110.01690033746098, -112.75938920157155, -109.27158857362184, -111.19519821680541, -110.14381902425255, -110.45955291199236, -111.55660330002316, -110.75604254261134, -111.02122553784838, -111.6490091060193, -110.93362819419399, -110.49033159684308, -110.70789549836027, -110.41991882034145, -110.0264093421208, -109.18432746063652, -110.15292268755287, -112.40733942236504, -111.32869665965416, -110.95418667871114, -111.14291568823575, -111.75555369152653, -112.98146297069803, -109.73870744292117, -111.33806139459435, -110.18838799491355, -112.60408243005732, -110.26112648646833, -110.58257045107274, -109.75155437454112]}, ...(2 in all)]
  in  "FFT 1 Choice 1":u16(ring) items=["T1 Y", "T1 X", "T1 Sum", "T2 Y", "T2 X", "T2 Sum", "T1 FB X", "T1 FB Sum", "T2 FB X", "T2 FB Sum", "PSD Y", "PSD X", "PSD Y Sum", "none"]
  in  "FFT 2 Choice 1":u16(ring)=3 items=["T1 Y", "T1 X", "T1 Sum", "T2 Y", "T2 X", "T2 Sum", "T1 FB X", "T1 FB Sum", "T2 FB X", "T2 FB Sum", "PSD Y", "PSD X", "PSD Y Sum", "none"]
  in  "FFT 1 Choice 2":u16(ring)=1 items=["T1 Y", "T1 X", "T1 Sum", "T2 Y", "T2 X", "T2 Sum", "T1 FB X", "T1 FB Sum", "T2 FB X", "T2 FB Sum", "PSD Y", "PSD X", "PSD Y Sum", "none"]
  in  "FFT 2 Choice 2":u16(ring)=4 items=["T1 Y", "T1 X", "T1 Sum", "T2 Y", "T2 X", "T2 Sum", "T1 FB X", "T1 FB Sum", "T2 FB X", "T2 FB Sum", "PSD Y", "PSD X", "PSD Y Sum", "none"]
  in  "Reset FFT":bool
  in  "# Spectra to Ave.":dbl=25.0
  out "Ave. Time (s)":dbl=1.5
  in  "Tab Green FB":T3(tab)
  in  "Feedback \noverload":bool
  in  "Shunt 2":bool
  in  "Capture Exp":bool
  in  "Capture Bottom":bool
  in  "VISA Clear":bool
  in  "Scale factor":dbl=0.5
  in  "Scale intensities (Q)":bool
  in  "Read Cal":bool
  in  "Confocal Linescan":bool
  in  "Confocal Image":bool
  in  "T1 offX (V)":dbl=0.044 format="%#_2g"
  in  "T1 kaX (pN/nm)":dbl=0.1608167093260824 min=0.0 step=0.001 format="%#_2g"
  out "Time (s)":dbl=40.5
  out "Total Time (s)":dbl=60.0
  in  "Start Saving":bool
  in  "Cal sets":u32=50 min=1 step=1
  in  "Comment":string="testing confocal setup"
  out "Calibrating...":bool
  in  "Trap 2 (R)":bool=TRUE
  in  "Trap 1 (E)":bool=TRUE
  in  "Save Calibration":bool
  in  "N sets to save":u32=200 caption="N Sets"
  in  "Save N Sets":bool
  out "Save file name":path=path "I:/Data/160525/160525_043.dat"
  in  "Save ave N":i32=500 caption="Avg N"
  out "Saving...":bool
  in  "Stop Saving":bool
  out "Progress":u16(slide) scale=0.0..100.0
  out "MouseMove Trap":bool
  out "Buffer Status":dbl(slide) scale=0.0..1.0
  out "Overflow (data lost)":bool
  in  "Reset":bool
  out "Data Rate (Hz)":dbl=66666.66666666667 caption="Trap Data Rate (Hz)" format="%#_3p"
  out "Save Data Rate (Hz)":dbl=133.33333333333334 caption="Rate (Hz)" format="%#_3p"
  in  "T1 alX (nm/V)":dbl=701.8425766517444 step=10.0 format="%#_3g"
  in  "T2 alX (nm/V)":dbl=806.869454518421 step=10.0 format="%#_3g"
  in  "T2 kaX (pN/nm)":dbl=0.13871102209446912 min=0.0 step=0.001 format="%#_2g"
  in  "T2 offX (V)":dbl=-0.016 format="%#_2g"
  in  "BD 1 Frq 2 (MHz)":dbl=90.0 caption="T2 X (MHz)" min=60.0 max=90.0 step=1.0 format="%#_6p"
  in  "MCL Y":dbl(slide)=4.669617603076266 caption="Confocal Y (V)" min=0.0 max=10.0 step=0.01 scale=0.0..10.0 scale format="%_1f"
  in  "MCL X":dbl(slide)=3.742542191839351 caption="Confocal X (V)" min=0.0 max=10.0 step=0.01 scale=0.0..10.0 scale format="%_1f"
  in  "Trap Raster":bool
  out "Raster Scanning...":bool
  in  "Trap Delta (MHz)":dbl(slide)=20.0 step=1.0 scale=8.0..20.0
  in  "Trap Powers (V)":cluster{"Set 1":dbl, "Set 2":dbl}={"Set 1"=5.0, "Set 2"=5.0}
  in  "Index":dbl=43.0 caption="Save File Index" min=1.0 step=1.0
  in  "BD 1 Frq 1 (MHz)":dbl=70.0 caption="T1 X (MHz)" min=60.0 max=90.0 step=1.0 format="%#_6p"
  in  "Goto Top":bool
  in  "Capture Top":bool
  out "X Pos":string="-0.85624\r\n"
  out "Y Pos":string="0.27735\r\n"
  out "Z Pos Pos":string="0.05734\r\n"
  out "X Motion":string="1\r\n"
  out "Y Motion":string="1\r\n"
  out "Z motion":string="1\r\n"
  in  "Goto Bottom (F7)":bool
  in  "Goto Exp (F8)":bool
  in  "Inject Main":bool caption="Inject Pump 3"
  in  "Shunt 1":bool
  in  "Inject Bottom":bool
  in  "Scan Range (nm)":dbl=1683.3000000000002
  in  "Green Laser":bool
  in  "Current (%)":dbl=10.0 min=0.0 max=100.0 step=1.0
  in  "Green laser mode":enum32{"Laser ON", "Laser OFF", "Interlace"}(radio)
  in  "Symmetric?":bool
  in  "Locations":string[][](array[string])=[["N.D.\r\n", "N.D.\r\n", "N.D.\r\n"], ["N.D.\r\n", "N.D.\r\n", "N.D.\r\n"], ["N.D.\r\n", "N.D.\r\n", "N.D.\r\n"], ["N.D.\r\n", "N.D.\r\n", "N.D.\r\n"]]
  out "PD Sum":dbl
  in  "Inject Top":bool caption="Inject Pump 1"
  in  "APD Integration Time (s)":dbl=0.01 caption="APD Int. Time (s)"
  in  "APD Gate":enum32{"ON", "OFF", "Interlace"}(radio)=enum."Interlace"
  in  "ESP ZR-Limit":string="0.09900"
  in  "ESP ZL-Limit":string="-0.09900"
  in  "Sym. Mid (MHz)":dbl=78.0
  in  "Asym. T2 (MHz)":dbl=85.0
  in  "MouseMove Speed":cluster{"Horizontal":dbl, "Vertical":dbl}={"Horizontal"=-0.075, "Vertical"=0.01}
  out "MouseX":i32
  in  "Load parameters":bool
  in  "Saved AOD Raster Scan Parameter Sets":T4(array[cluster])=[{"Scan Range AOD (nm) 2"=500.0, "Step Size AOD (nm) 2"=1.0, "Scan Speed AOD (nm/s) 2"=100.0, "Number of scans (AOD) 2"=1, "Label"="offset curve"}, {"Scan Range AOD (nm) 2"=1000.0, "Step Size AOD (nm) 2"=1.0, "Scan Speed AOD (nm/s) 2"=100.0, "Number of scans (AOD) 2"=1, "Label"="hp raster check"}, {"Scan Range AOD (nm) 2"=6.8, "Step Size AOD (nm) 2"=0.34, "Scan Speed AOD (nm/s) 2"=0.34, "Number of scans (AOD) 2"=1, "Label"="3.4 kbp - 1 bp steps"}]
  in  "Start MCL Scan":bool
  out "MCL Scanning":bool
  out "MCL Scan I":u64=2
  in  "Abort MCL Scan":bool
  out "Actual MCL Inc (V)":dbl=0.14099551377910702
  out "Cycles/step (MCL)":u64=2000 caption="Cycles/step" format="%.0p"
  out "Data points/scans (MCL)":dbl=4800.0 caption="Data points/scan"
  out "MCL Scan N Sets":dbl=160.0 caption="MCL Scan N sets"
  out "Desired Scan Incr (V)":dbl=0.14102564102564102
  out "Desired incr (int)":dbl=462.098717948718
  in  "Save Data (MCL)":bool=TRUE caption="Save Data"
  in  "Center Scan":bool=TRUE
  in  "Continuous MCL Scanning":bool caption="Cont. Scanning"
  in  "Restart DMA? (MCL)":bool=TRUE caption="Restart DMA?"
  in  "Scan Range (V)":dbl=3.5
  in  "N APD Samp/step":i32=3
  in  "Scan steps (x)":u64=40
  in  "Number of scans (MCL)":u64=1 caption="Scans"
  out "Initial Y":dbl=2.5691326639606933
  out "Initial X":dbl=1.6310662274449115
  in  "2D or 1D Scan":bool=TRUE
  in  "Fast Scan Dir":bool=TRUE
  in  "Scan lines (y)":u64=20
  out "MCL Scan Time (s)":dbl=48.0
  out "Reset MCL after scan":bool
  out "Zero MCL x position":dbl=5.6547922360429315
  out "Zero T1 position":dbl=70.0
  in  "Tracking factor":dbl=-0.45
  out "Current MCL (V)":dbl=5.657514378627918
  in  "Tab IR Control":T5(tab)=enum."Trap Raster"
  out "Total Counts (ticks)":u32=600
  in  "Trap ON/OFF X or Y Amp?":bool=TRUE
  in  "Trap 1 ON":bool=TRUE
  in  "Number Interlace Sets":u8=3 min=1 max=3
  in  "DIO count 3 (ticks)":u32=200
  in  "DIO count 2 (ticks)":u32=200
  in  "DIO count 1 (ticks)":u32=200
  in  "BD 2 Amp 3 (%)":dbl min=0.0 max=75.0 step=1.0
  in  "BD 2 Amp 2 (%)":dbl min=0.0 max=75.0 step=1.0
  in  "BD 2 Amp 1 (%)":dbl min=0.0 max=75.0 step=1.0
  in  "BD 1 Amp 3 (%)":dbl min=0.0 max=75.0 step=1.0
  in  "BD 1 Amp 2 (%)":dbl=42.0 min=0.0 max=75.0 step=1.0
  in  "BD 1 Amp 1 (%)":dbl=40.0 min=0.0 max=75.0 step=1.0
  in  "BD 2 Frq 3 (MHz)":dbl=26.0 min=60.0 max=90.0 step=1.0 format="%#_6p"
  in  "BD 1 Frq 3 (MHz)":dbl=70.0 min=60.0 max=90.0 step=1.0 format="%#_6p"
  in  "BD 2 Frq 2 (MHz)":dbl=26.0 min=60.0 max=90.0 step=1.0 format="%#_6p"
  in  "BD 2 Frq 1 (MHz)":dbl=26.0 min=60.0 max=90.0 step=1.0 format="%#_6p"
  in  "Not-Interlacing Set":enum32{"Set 1", "Set 2", "Set 3"}(radio)
  in  "Interlace":bool=TRUE
  in  "Trap 2 ON":bool=TRUE
  in  "Trap 3 ON":bool
  in  "Freq or Amp switch first":bool=TRUE
  in  "Swap F1 and F2":bool
  in  "Amp switch delay":u16=4
  in  "Freq switch delay":u16=9
  in  "Next trap write delay (ticks)":u16
  in  "Phase offset method":u8=3
  in  "Phase increment trap 1":fxp<+/-,64,32>
  in  "Phase increment trap 2":fxp<+/-,64,32>
  in  "RF phase reset before cycles":bool
  in  "Raster to target force?":bool
  in  "Raster target force (pN)":dbl=10.0
  in  "MCL Step Increment (V_int)":dbl=3.0
  out "Time to Finish All (min)":dbl=0.666 format="%#_2p"
  in  "Scan Speed (nm/s)":dbl=100.0
  in  "Step Size (nm)":dbl=1.0
  in  "MCL/AOM Scale Tweak":dbl=1.0
  in  "MCL Step Position Ratio":dbl=0.5
  in  "Move MCL Also?":bool
  out "Save index":dbl=43.0
  out "Final delta (MHz)":dbl=30.0
  out "Initial delta (MHz)":dbl=20.0
  out "Scan Range (MHz)":dbl=-10.0
  in  "Restart DMA? (AOD)":bool=TRUE caption="Restart DMA?"
  out "Time/Scan (s) (AOD)":dbl=19.98 format="%#_2p"
  in  "Save scans":bool=TRUE
  out "AOD Scan I":u64=2 caption="Scan I"
  in  "Continuous AOD Scanning":bool caption="Continuous Scanning"
  in  "Abort AOD Scan":bool caption="Abort Scan"
  in  "Scan BD":bool=TRUE
  out "Cycles/step (AOD)":u64=666 format="%.3p"
  in  "N F/B Scans (AOD)":u16=1 min=1
  out "Scan steps (AOD)":u64=2000
  out "Scan Step (MHz)":dbl=-0.0050025012506253125
  out "AOD Scanning":bool caption="Scanning"
  in  "Start AOD Scan":bool caption="Start Scan"
  out "Trap Raster N Sets":dbl=133.2
  out "Progress 2":u16(slide) caption="Progress" scale=0.0..100.0
  in  "Abort save 2":bool caption="Abort save"
  out "Trap 2 amp.":dbl
  out "Trap 1 amp.":dbl
  in  "PID gains":T6={"proportional gain (Kc)"=0, "integral gain (Kc*Ts/Ti)"=5, "derivative gain (Kc*Td/Ts)"=0}
  in  "All FB On/Off":bool
  in  "AI2 to Setpoint":cluster{"Set 1":bool, "Set 2":bool}
  out "AI2 (V)":cluster{"Set 1":dbl, "Set 2":dbl}={"Set 1"=3.087557603686636, "Set 2"=2.914212469862972}
  in  "Reset Feedback":cluster{"Set 1":bool, "Set 2":bool}
  in  "Feedback On/Off":cluster{"Set 1":bool, "Set 2":bool}={"Set 1"=TRUE, "Set 2"=TRUE}
  in  "Auto read offset\ncorrection":bool=TRUE
  in  "Negate Diff?":bool
  in  "Diff. FB.":bool=TRUE
  in  "Dynamic Force FB":bool=TRUE
  in  "Reset Trap Pos. FB":bool
  in  "Tab FFB Settings":enum32{"Main Setting", "Details"}(tab)
  in  "Use Offset in FFB?":bool=TRUE
  in  "Setpoint correction\noffset file":path
  in  "Negate offset difference":bool
  out "B factor":dbl=0.9916156324677038
  in  "Trap Pos FB Int Count":u16=100
  in  "Trap Pos. FB Gains":T7={"proportional gain (Kc)"=20.0, "integral gain (Kc*Ts/Ti)"=3.0, "derivative gain (Kc*Td/Ts)"=0.0} {"proportional gain (Kc)" format="%.11g"; "integral gain (Kc*Ts/Ti)" format="%.11g"; "derivative gain (Kc*Td/Ts)" format="%.11g"}
  in  "Read setpoint correction":bool
  in  "Trap Pos. FB Offset Factor":i64
  in  "Trap Pos FB Negate Action":bool=TRUE
  in  "Trap Pos. FB Mult Factor":i64=8388608
  in  "Trap Pos. AI1 X Pre-scale":u16
  in  "Trap Pos. FB Range":T8={"output high"=0.999969482421875, "output low"=-1.0}
  out "Trap Pos FB Int Signal":fxp<+/-,24,9>=42.09515380859375 format="%.18g"
  out "Trap Pos FB Int-Norm Signal":fxp<+/-,16,1>=0.042083740234375 format="%.16g"
  in  "Set SP Using...":bool
  in  "Trap Pos FB Monitor\nT1 or T2":bool
  out "Trap X AI1 (DMA)":T9={"Set 1"=0.030731201171875, "Set 2"=-0.0113525390625}
  out "Trap Pos FB Action":i64=-32767
  in  "Setpoint offset\nCorrection values":dbl[](array[numeric])=[0.024496601698410773, 0.024671186719617436, 0.024845771740824106, 0.025020356762030765, 0.02519494178323743, 0.025369526804444095, 0.025544111825650764, 0.025718696846857424, 0.025893281868064093, 0.026067866889270756, 0.026242451910477423, 0.026417036931684082, 0.02659162195289075, 0.026766206974097418, 0.02694079199530408, 0.027115377016510744, 0.027289962037717407, 0.027464547058924076, 0.02763913208013074, 0.027813717101337402, 0.027988302122544065, 0.02816288714375073, 0.028337472164957394, 0.02851205718616406, 0.028686642207370723, 0.028861227228577393, 0.02903581224978405, 0.029210397270990722, 0.029384982292197385, 0.02955956731340405, 0.02973415233461071, 0.029908737355817377, 0.030083322377024047, 0.03025790739823071, 0.030432492419437372, 0.030607077440644035, 0.0307816624618507, 0.030956247483057368, 0.03113083250426403, 0.0313054175254707, 0.03148000254667736, 0.03165458756788402, 0.03182917258909068, 0.03200375761029735, 0.032178342631504014, 0.03235292765271068, 0.03252751267391735, 0.03270209769512401, 0.03287668271633068, 0.033051267737537346, 0.033225852758744005, 0.03340043777995067, 0.03357502280115733, 0.033749607822364, 0.033924192843570664, 0.03409877786477733, 0.034273362885983996, 0.034447947907190656, 0.03462253292839732, 0.03479711794960398, 0.03497170297081065, 0.035146287992017314, 0.03532087301322398, 0.035495458034430646, 0.035670043055637306, 0.03584462807684397, 0.036019213098050645, 0.036193798119257305, 0.03636838314046397, 0.03654296816167063, 0.0367175531828773, 0.03689213820408396, 0.03706672322529063, 0.037241308246497296, 0.037415893267703955, 0.03759047828891062, 0.03776506331011729, 0.03793964833132395, 0.03811423335253061, 0.03828881837373728, 0.038463403394943946, 0.038637988416150605, 0.03881257343735727, 0.03898715845856393, 0.0391617434797706, 0.03933632850097726, 0.03951091352218393, 0.039685498543390596, 0.03986008356459726, 0.04003466858580393, 0.040209253607010595, 0.040383838628217254, 0.04055842364942392, 0.04073300867063058, 0.040907593691837246, 0.04108217871304391, 0.04125676373425058, 0.041431348755457245, 0.0416059337766639, 0.041780518797870564, 0.04195510381907723, 0.042129688840283896, 0.04230427386149057, 0.04247885888269723, 0.042653443903903895, 0.04282802892511056, 0.04300261394631722, 0.04317719896752389, 0.043351783988730554, 0.04352636900993721, 0.04370095403114388, 0.043875539052350546, 0.04405012407355721, 0.04422470909476388, 0.04439929411597054, 0.044573879137177204, 0.04474846415838387, 0.044923049179590537, 0.045097634200797196, 0.04527221922200386, 0.04544680424321053, 0.045621389264417195, 0.04579597428562386, 0.04597055930683052, 0.04614514432803718, 0.046319729349243846, 0.04649431437045051, 0.04666889939165718, 0.046843484412863845, 0.04701806943407051, 0.04719256456184452, 0.04736536676840916, 0.04753446267808822, 0.047696991448649737, 0.04784953848765512, 0.04799284096907562, 0.048127712917801824, 0.048257934523222495, 0.04838705366421733, 0.04851995197559876, 0.04865949840047511, 0.04880178465045004, 0.0489357994772595, 0.04905304538798107, 0.0491519464532862, 0.049234486275402736, 0.04930263064515607, 0.04935733149089569, 0.04939552771001872, 0.04941451823245213, 0.04941830757306315, 0.049410747020732684, 0.049392795273013504, 0.049367258833286985, 0.049339629147657244, 0.049311849604908836, 0.04928407006216041, 0.049256290519411994, 0.04922851097666357, 0.04920073143391515, 0.04917295189116673, 0.04914517234841831, 0.049117392805669895, 0.049089613262921473, 0.04906183372017306, 0.04903405417742463, 0.04900627463467622, 0.0489784950919278, 0.048950715549179374, 0.04892293600643097, 0.04889515646368254, 0.048867376920934125, 0.0488395973781857, 0.04881181783543728, 0.04878403829268886, 0.04875625874994044, 0.048728479207192026, 0.0487006996644436, 0.04867292012169519, 0.04864514057894676, 0.04861736103619835, 0.048589581493449926, 0.048561801950701505, 0.04853402240795309, 0.04850624286520466, 0.04847846332245625, 0.04845068377970783, 0.04842290423695941, 0.048395124694210985, 0.04836734515146257, 0.04833956560871415, 0.04831178606596573, 0.048284006523217314, 0.048256226980468886, 0.04822844743772048, 0.04820066789497206, 0.048172888352223636, 0.048145108809475215, 0.048117329266726794, 0.04808954972397837, 0.04806177018122996, 0.048033990638481544, 0.048006211095733116, 0.0479784315529847, 0.04795065201023628, 0.04792287246748786, 0.04789509292473944, 0.04786731338199102, 0.0478395338392426, 0.04781175429649418, 0.04778397475374576, 0.047756195210997346, 0.047728415668248925, 0.047700636125500503, 0.04767285658275208, 0.04764507704000366, 0.04761729749725524, 0.047589517954506826, 0.047561738411758404, 0.04753395886900998, 0.04750617932626157, 0.04747839978351315, 0.047450620240764727, 0.047422840698016305, 0.047395061155267884, 0.04736728161251948, 0.047339502069771056, 0.047311722527022634, 0.04728394298427421, 0.04725616344152579, 0.04722838389877737, 0.047200604356028956, 0.047172824813280535, 0.047145045270532114, 0.0471172657277837, 0.04708948618503528, 0.04706170664228686, 0.047033927099538436, 0.047006147556790015, 0.0469783680140416, 0.04695058847129318, 0.04692280892854476, 0.046895029385796344, 0.04686724984304792, 0.0468394703002995, 0.04681169075755108, 0.04678391121480266, 0.04675613167205424, 0.046728352129305824, 0.0467005725865574, 0.04667279304380899, 0.04664501350106057, 0.046617233958312146, 0.046589454415563725, 0.046561674872815303, 0.04653389533006689, 0.046506115787318475, 0.046478336244570054, 0.04645055670182163, 0.04642277715907321, 0.04639499761632479, 0.04636721807357637, 0.046339438530827955, 0.04631165898807953, 0.04628387944533112, 0.0462560999025827, 0.04622832035983428, 0.046200540817085856, 0.046172761274337434, 0.04614498173158901, 0.04611720218884059, 0.04608942264609218, 0.046061643103343757, 0.04603386356059534, 0.04600608401784692, 0.0459783044750985, 0.04595052493235008, 0.04592274538960166, 0.045894965846853236, 0.045867186304104815, 0.0458394067613564, 0.045811627218607986, 0.045783847675859565, 0.045756068133111144, 0.04572828859036272, 0.0457005090476143, 0.04567272950486588, 0.04564494996211747, 0.04561717041936905, 0.04558939087662063, 0.04556161133387221, 0.04553383179112379, 0.04550605224837537, 0.045478272705626946, 0.045450493162878525, 0.04542271362013011, 0.045394934077381696, 0.045367154534633275, 0.045339374991884854, 0.04531159544913643, 0.04528381590638801, 0.04525603636363959, 0.04522825682089117, 0.045200477278142755, 0.045172697735394333, 0.04514491819264592, 0.0451171386498975, 0.04508935910714908, 0.045061579564400656, 0.045033800021652234, 0.04500602047890381, 0.04497824093615539, 0.044950461393406985, 0.04492268185065856, 0.04489490230791014, 0.04486712276516172, 0.0448393432224133, 0.04481156367966488, 0.044783784136916464, 0.04475600459416805, 0.04472822505141963, 0.04470044550867121, 0.044672665965922786, 0.044644886423174365, 0.044617106880425944, 0.04458932733767752, 0.04456154779492911, 0.044533768252180694, 0.04450598870943227, 0.04447820916668385, 0.04445042962393543, 0.04442265008118701, 0.04439487053843859, 0.04436709099569017, 0.04433931145294175, 0.04431153191019333, 0.04428375236744492, 0.044255972824696496, 0.044228193281948075, 0.044200413739199654, 0.04417263419645123, 0.04414485465370281, 0.0441170751109544, 0.04408929556820598, 0.04406151602545756, 0.04403373648270914, 0.04400595693996072, 0.0439781773972123, 0.043950397854463884, 0.04392261831171546, 0.04389483876896704, 0.04386705922621863, 0.043839279683470206, 0.043811500140721785, 0.04378372059797336, 0.04375594105522494, 0.04372816151247652, 0.04370038196972811, 0.04367260242697968, 0.043644822884231264, 0.04361704334148285, 0.04358926379873443, 0.04356148425598601, 0.043533704713237587, 0.043505925170489165, 0.04347814562774075, 0.04345036608499233, 0.043422586542243916, 0.043394806999495494, 0.04336702745674707, 0.04333924791399865, 0.04331146837125023, 0.043283688828501816, 0.0432559092857534, 0.04322812974300498, 0.04320035020025656, 0.04317257065750814, 0.04314479111475972, 0.043117011572011296, 0.04308923202926288, 0.04306145248651446, 0.04303367294376604, 0.043005893401017625, 0.0429781138582692, 0.04295033431552078, 0.04292255477277236, 0.04289477523002394, 0.04286699568727552, 0.0428392161445271, 0.042811436601778684, 0.04278365705903027, 0.04275587751628185, 0.04272809797353343, 0.042700318430785006, 0.042672538888036585, 0.042644759345288163, 0.04261697980253975, 0.04258920025979133, 0.04256142071704291, 0.04253364117429449, 0.04250586163154607, 0.04247808208879765, 0.04245030254604923, 0.04242252300330081, 0.042394743460552387, 0.04236696391780398, 0.04233918437505556, 0.04231140483230714, 0.042283625289558716, 0.042255845746810294, 0.04222806620406188, 0.04220028666131346, 0.04217250711856504, 0.042144727575816616, 0.0421169480330682, 0.04208916849031978, 0.04206138894757136, 0.04203360940482294, 0.04200582986207452, 0.0419780503193261, 0.041950270776577675, 0.04192249123382926, 0.041894711691080846, 0.041866932148332425, 0.041839152605584004, 0.04181137306283558, 0.04178359352008716, 0.04175581397733874, 0.04172803443459032, 0.0417002548918419, 0.04167247534909349, 0.04164469580634507, 0.04161691626359665, 0.04158913672084823, 0.041561357178099806, 0.0415335776353514, 0.04150579809260298, 0.041478018549854556, 0.041450239007106135, 0.041422459464357714, 0.04139467992160929, 0.04136690037886087, 0.04133912083611246, 0.04131134129336403, 0.04128356175061562, 0.04125578220786719, 0.04122800266511878, 0.04120022312237036, 0.04117244357962194, 0.041144664036873516, 0.041116884494125094, 0.04108910495137668, 0.04106132540862826, 0.04103354586587984, 0.041005766323131417, 0.040977986780383, 0.04095020723763458, 0.04092242769488616, 0.04089464815213774, 0.04086686860938932, 0.0408390890666409, 0.04081130952389249, 0.04078352998114407, 0.040755750438395646, 0.040727970895647225, 0.040700191352898804, 0.04067241181015039, 0.040644632267401976, 0.04061685272465355, 0.04058907318190513, 0.04056129363915671, 0.04053351409640829, 0.04050573455365987, 0.04047795501091145, 0.040450175468163034, 0.04042239592541461, 0.0403946163826662, 0.04036683683991778, 0.04033905729716935, 0.040311277754420935, 0.040283498211672514, 0.0402557186689241, 0.04022793912617567, 0.04020015958342725, 0.040172380040678836, 0.04014460049793042, 0.040116820955182, 0.04008904141243358, 0.04006126186968516, 0.04003348232693674, 0.04000570278418832, 0.03997792324143991, 0.03995014369869149, 0.039922364155943066, 0.039894584613194645, 0.03986680507044622, 0.0398390255276978, 0.03981124598494939, 0.03978346644220096, 0.039755686899452546]
  out "Offset file step size":dbl=0.1
  in  "N El. to Ave.":i32=10000
  in  "Trap Pos. FB Out Scale 2^n":u8=23 caption="Action Scale"
  out "FFB AvgX":T10={"Trap 1"=0.030792236328125, "Trap 2"=-0.011322021484375}
  in  "Trap Pos FB SP":fxp<+/-,16,1>=0.231353759765625 caption="Manual FFB Setpoint"
  out "Actual setpoint":fxp<+/-,16,1> format="%.16g"
  in  "Tab Control":T11(tab)
  in  "- phase (AI1)":bool
  in  "+ phase (AI1)":bool
  out "Counts/DMA":dbl=12000000.0 format="%#_6p"
  out "Trap Sets":u32=2
  out "FPGA Averaging":bool
  out "DMA Update Period (s)":dbl=0.3
  out "Ave. Period (s)":dbl=5e-06 format="%#_6p"
  in  "FPGA Ave.":dbl=1.0 min=1.0 step=1.0
  in  "Sets to FIFO (Traps)":T12={"Set 1"=TRUE, "Set 2"=TRUE, "Set 3"=FALSE}
  in  "N Acq Sets (Traps + Fl.)":i16=3
  in  "Detector Type":string(combo)="UCB Fleezers 052511"
  in  "Trap AI FIFO Depth":u32=340000 format="%.0p"
  out "# Samples/channel":u32=40000 format="%.0p"
  in  "AI Count (ticks)":u32=200
  out "AI rate (Hz)":dbl=200000.0 format="%#_6p"
  in  "Initial Phase Adjustment (AI1)":i16=185
  out "Late Counter (AI1)":u8
  out "Relative phase (AI1)":i16
  in  "Phase adj. (AI1)":i16
  out "Trap FIFO El. Left":u32 format="%.0p"
  out "Trap FIFO El/Read":u32=320000 format="%.0p"
  in  "# Samples/trap":u32=20000 format="%.0p"
  out "AI labels":string[](array[string])=["T1 Y", "T1 X", "T1 Sum", "T2 Y", "T2 X", "T2 Sum", "T1 FB X", "T2 FB Sum", "T2 FB X", "T2 FB Sum", "PSD Y", "PSD X", "PSD Sum"]
  in  "Green int current ON count adj":u32=150
  in  "GI Frequency, OFF count":u32=450 min=1 step=1
  in  "GI Frequency, ON count":u32=150 min=1 step=1
  out "GI Late Counter 2":u16
  in  "Phase adj. (GI) 2":i16=20
  out "GI relative phase 2":i16
  in  "+ phase (GI) 2":bool
  in  "Initial Phase Adjustment (GI) 2":i16=-100
  in  "- phase (GI) 2":bool
  in  "- phase (GI)":bool
  in  "Initial Phase Adjustment (GI)":i16=4
  in  "+ phase (GI)":bool
  out "GI relative phase":i16
  in  "Phase adj. (GI)":i16=5
  out "GI Late Counter":u8
  in  "Invert GI":bool
  out "MCL Late Counter":u8
  in  "- phase (MCL)":bool
  in  "+ phase (MCL)":bool
  in  "Update Count (MCL)":u32=600
  in  "Initial Phase Adj. (MCL)":i16 caption="Initial Phase Adj."
  out "Relative Phase (MCL)":i16 caption="Relative Phase"
  in  "Phase adjust (MCL)":i16 caption="Phase adjust"
  in  "Green FB On/Off":bool
  in  "Green FB Gains":T6={"proportional gain (Kc)"=10, "integral gain (Kc*Ts/Ti)"=5, "derivative gain (Kc*Td/Ts)"=0}
  in  "Initial Phase Adjustment (Green FB)":i16=50
  in  "Phase adj. (Green FB)":i16=10
  in  "- phase (Green FB)":bool
  in  "+ phase (Green FB)":bool
  out "Relative phase (Green FB)":i16
  out "Green FB Signals (V)":cluster{"Y":dbl, "X":dbl, "Sum":dbl}={"Y"=-0.999969482421875, "X"=1.0, "Sum"=-10.00030518509476}
  in  "Green FB Setpoint (mV)":dbl=100.0
  in  "Green FB Count":u32=600
  in  "Trap Position FIFO Depth":u32=300000 format="%.0p"
  out "TPos FIFO El Left":u32=171
  out "TPos FIFO El/Read":u32=120000 format="%.0p"
  out "Trap AI FIFO Timeout":u16
  out "Trap Pos FIFO Timeout":u16
  in  "APD FIFO Depth (requires restart)":u32=300000 format="%.0p"
  in  "- phase (APD 2 Gate)":bool
  in  "+ phase (APD 2 Gate)":bool
  out "APD FIFO El/Read":u32=60
  out "APD Samples/FIFO Acq.":dbl=30.0
  in  "APD Gate ON Count":u32=150 caption="Gate ON Count"
  in  "APD Gate OFF Count":u32=450 caption="Gate OFF Count"
  in  "Invert APD Gate":bool caption="Invert Gate"
  in  "Initial Phase Adjustment (APD Acq)":i16
  in  "Phase Adj. (APD Acq)":i16=20
  out "APD Acq Relative Phase":i16
  out "APD Acq Late Counter":u16
  in  "+ phase (APD Acq)":bool
  in  "- phase (APD Acq)":bool
  out "APD FIFO El Left":u32
  in  "Initial Phase Adjustment (APD 1 Gate)":i16=50
  in  "Phase Adj. (APD 1 Gate)":i16=20
  out "APD 1 Gate Relative Phase":i16
  in  "+ phase (APD 1 Gate)":bool
  in  "- phase (APD 1 Gate)":bool
  out "APD 1 Gate Late Counter":u8
  in  "Initial Phase Adjustment (APD 2 Gate)":i16=45
  in  "Phase Adj. (APD 2 Gate)":i16=20
  out "APD 2 Gate Relative Phase":i16
  out "APD 2 Gate Late Counter":u8
  in  "Read Lateness and Rel Phase":bool
  in  "AOM X Cal (nm/MHz)":dbl=160.0
  in  "MCL X Cal (nm/V)":dbl=1174.0
  out "X RF Amp Limits (%)":T13={"Minimum"=0.0, "Maximum"=75.0, "Increment"=1.0}
  out "X RF Freq Limits (MHz)":T13={"Minimum"=60.0, "Maximum"=90.0, "Increment"=1.0}
  out "Y RF Frequency Limits (MHz)":T13={"Minimum"=60.0, "Maximum"=90.0, "Increment"=1.0}
  out "Y RF Amplitude Limits (%)":T13={"Minimum"=0.0, "Maximum"=75.0, "Increment"=1.0}
  in  "Delay to Interlace (s)":dbl
  in  "Delayed Interlace Start":bool
  in  "Cal read wait (s)":u32=5
  in  "Save TPos":bool=TRUE
  in  "Save APD":bool=TRUE
  in  "Activate Joystick":bool
  in  "ESP Port":refnum<visa-resource-name>="COM4"
  in  "APD 2 AO Mult.":i16=1 min=1
  in  "APD 1 AO Mult.":i16=1 min=1
  in  "Offset Values":T14={"Trap 1X offset"=array[500 elements], "Trap 2X offset"=array[500 elements]}
  in  "Init Valve?":bool=TRUE
  in  "NoStage?":bool
  out "Error Events":errorcluster
  out "Error Stage":errorcluster
  out "FPGA error out":errorcluster
  out "Read cal error":errorcluster
  # "Hidden Controls"
  # "Trap Display:"
  # "APD Display:"
  # "originally 10k"
  # "Select the chamber to go to"
  # "MCL Tracking Options"
  # "X"
  # "2D"
  # "Y"
  # "1D"
  # "X"
  # "Y"
  # "Trap interlacing RF phase control\n\n0 = no phase control\n1 = offset increments each trap cycle by values below\n2 = offset increment increases by increment factor each cycle\n3 = random phase (no parameters set)"
  # "X"
  # "Y"
  # "DON'T TURN ON\nUNTIL YOU CLOSE\nTHE LOOP"
  # "FPGA\nreading"
  # "DMA\ntransfer"
  # "(Samples/trap x Trap Sets)"
  # "(Samples/channel x\n8 if averaging (8 channels)\n4 if no averaging)"
  # "Trap 1"
  # "Trap 2"
  # "Flour./Trap 3"
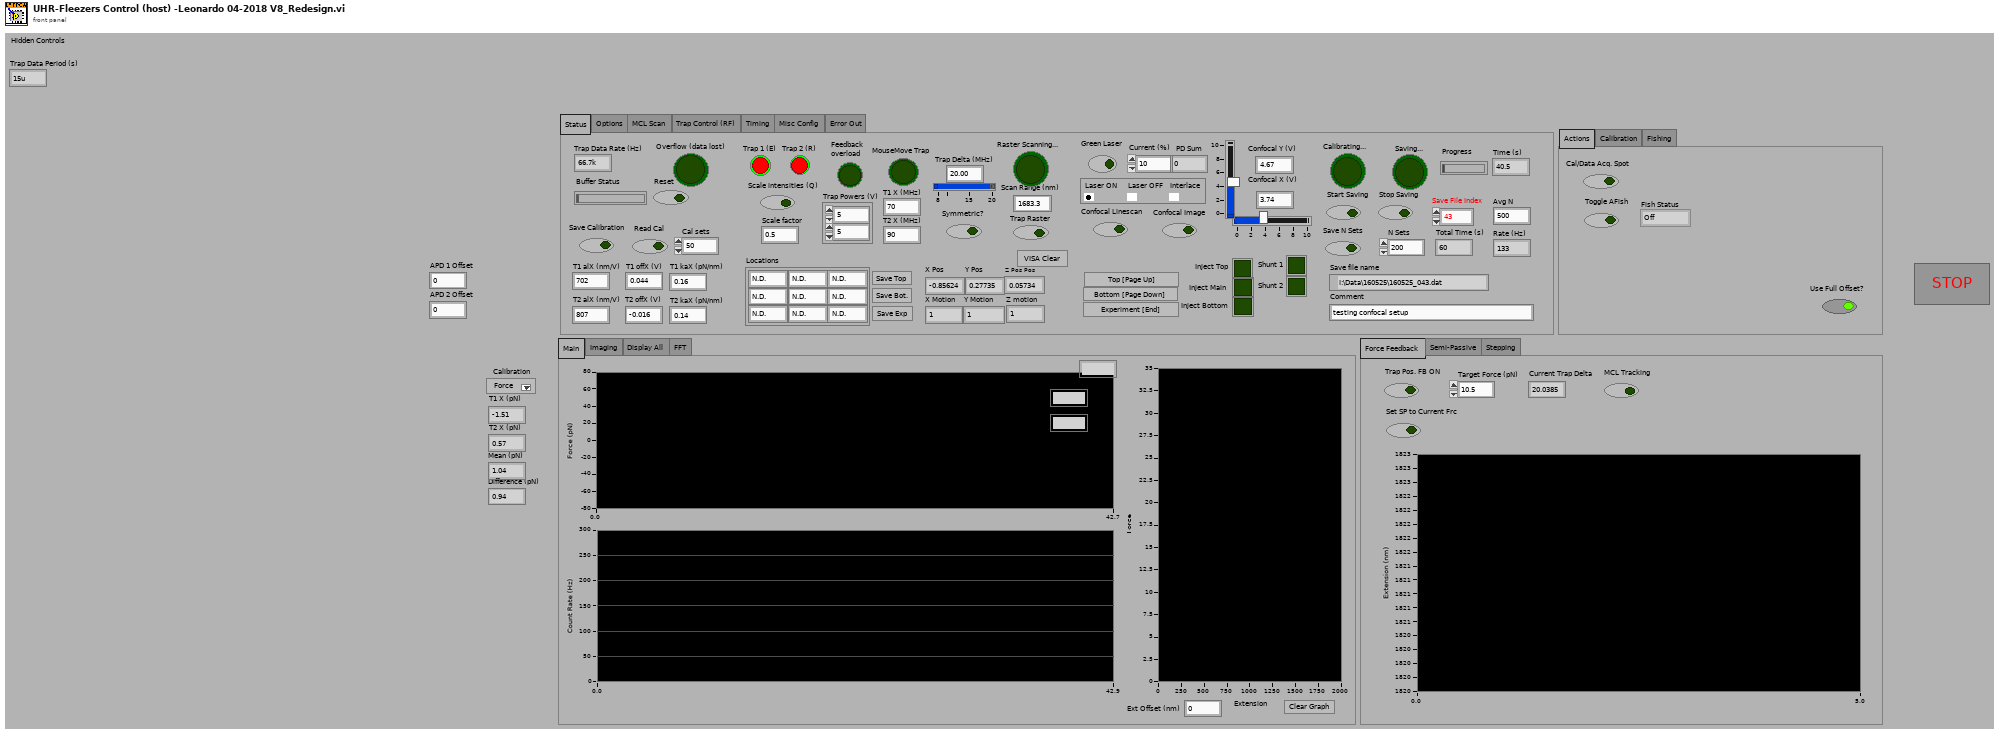
[diagram p1: front panel]
types:
  T1 = enum32{"Force Feedback", "Semi-Passive", "Stepping"}
  T2 = typedef "IMAQ Image.ctl" = refnum<image>
  T3 = enum32{"Status", "Options", "MCL Scan", "Trap Control (RF)", "Timing", "Misc Config", "Error Out"}
  T4 = cluster{"Scan Range AOD (nm) 2":dbl, "Step Size AOD (nm) 2":dbl, "Scan Speed AOD (nm/s) 2":dbl, "Number of scans (AOD) 2":u16, "Label":string}[]
  T5 = enum32{"RF Amp/Frq", "RF Phase", "Trap Raster", "Intensity Feedback", "Force Feedback"}
  T6 = cluster{"proportional gain (Kc)":i16, "integral gain (Kc*Ts/Ti)":i16, "derivative gain (Kc*Td/Ts)":i16}
  T7 = cluster{"proportional gain (Kc)":fxp<+/-,16,8>, "integral gain (Kc*Ts/Ti)":fxp<+/-,16,8>, "derivative gain (Kc*Td/Ts)":fxp<+/-,16,8>}
  T8 = cluster{"output high":fxp<+/-,16,1>, "output low":fxp<+/-,16,1>}
  T9 = cluster{"Set 1":fxp<+/-,16,1>, "Set 2":fxp<+/-,16,1>}
  T10 = cluster{"Trap 1":fxp<+/-,16,1>, "Trap 2":fxp<+/-,16,1>}
  T11 = enum32{"Trap", "Green", "Green FB", "TPos", "APD"}
  T12 = cluster{"Set 1":bool, "Set 2":bool, "Set 3":bool}
  T13 = typedef "LVMinMaxIncTypeDef.ctl" = cluster{"Minimum":dbl, "Maximum":dbl, "Increment":dbl}
  T14 = cluster{"Trap 1X offset":dbl[], "Trap 2X offset":dbl[]}
  T15 = typedef "Image Type" = u32
  T16 = typedef "nirio_resource_hc.ctl" = tag
  T17 = typedef "openfpgaref.initrf.ctl" = refnum<k20>
  T18 = typedef "openfpgaref.8.6.ctl" = refnum<k20>
  T19 = enum16{"CONNECT", "INITIALIZE VALVES", "DISCONNECT", "MOVE VALVE"}
  T20 = cluster{"New Image":T2, "New Image":T2, "New Image":T2, "New Image":T2}
  T21 = typedef "XDNodeRunTimeDep.lvlib/timing_clust.ctl" = cluster{"Expected End [f-1]":u64, "Actual End [f-1]":u64, "Finished Late? [f-1]":bool, "Expected End [i-1]":u64, "Actual End [i-1]":u64, "Finished Late? [i-1]":bool, "Expected Start [i]":u64, "Actual Start [i]":u64, "Expected Start [f]":u64, "Actual Start [f]":u64, "Source Name":string, "Structure Name":string, "Period":i64, "Deadline":i64, "Offset":i64, "Start":i64, "Priority":i32, "Timeout":i32, "Mode":T22, "Wakeup Reason":T23, "Error":errorcluster, "Source Type":string, "Secondary Source Type":string, "Global End Time":u64, "Global Start Time":u64, "Frame Duration":u64, "Iteration Duration":u64, "Assigned CPU":i32, "I/O Scan Engine Mode":u32}
  T22 = typedef "XDNodeRunTimeDep.lvlib/nitl_modes.ctl" = enum32{"No Change", "Process missed periods, maintain original phase", "Discard missed periods, maintain original phase", "Process missed periods, ignore original phase", "Discard missed periods, ignore original phase"}
  T23 = typedef "XDNodeRunTimeDep.lvlib/wakeup.ctl" = enum32{"Normal", "Aborted", "Asynchronous wakeup", "Timing source error", "Timed loop error", "Timeout"}
  T24 = enum16{"open", "replace", "create", "open or create", "replace or create", "replace or create with confirmation"}
  T25 = enum16{"big-endian, network order", "native, host order", "little-endian"}
  T26 = cluster{"Scan Range AOD (nm) 2":dbl, "Step Size AOD (nm) 2":dbl, "Scan Speed AOD (nm/s) 2":dbl, "Number of scans (AOD) 2":u16, "Label":string}
  T27 = cluster{"[0]":dbl, "[1]":dbl, "[2]":dbl, "[3]":dbl, "[4]":dbl, "[5]":dbl}
  T28 = cluster{"Diameter (mm)":dbl, "Units":dbl, "Volume":dbl, "Rate":dbl}
  T29 = enum32{"Dual Display (Trap + Fluor.)", "Imaging", "Display All", "FFT"}
  T30 = cluster{"averaging mode":u16, "weighting mode":u16, "number of averages":u32}
  T31 = cluster{"dB On (F)":bool, "unwrap phase (F)":bool, "convert to degree (F)":bool}
  T32 = cluster{"Green FB Ch 0":i16, "Green FB Ch 1":i16, "Green FB Ch 2":i16}
  T33 = cluster{"f0":dbl, "df":dbl, "magnitude":dbl[]}[][]
  T34 = cluster{"Green FB Ch 0":dbl, "Green FB Ch 1":dbl, "Green FB Ch 2":dbl}
  T35 = cluster{"Label.Text":string, "Label.Text":string, "Label.Text":string, "Label.Text":string, "Label.Text":string}
  T36 = cluster{"Horizontal":i32, "Vertical":i32, "Scrolling":i32}
  T37 = typedef "LVPoint32TypeDef.ctl" = cluster{"Horizontal":i32, "Vertical":i32}
  T38 = cluster{"Left":i32, "Top":i32, "Width":u32, "Height":u32}
  T39 = cluster{"Left":i32, "Top":i32, "Width":u32, "Height":u32}[]
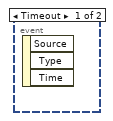
[diagram p2: hidden frame]
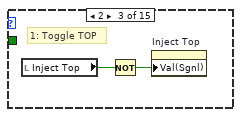
[diagram p6: hidden frame]
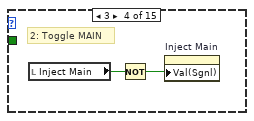
[diagram p7: hidden frame]
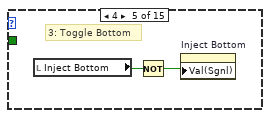
[diagram p8: hidden frame]
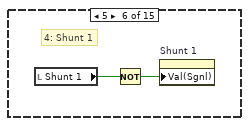
[diagram p9: hidden frame]
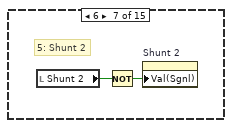
[diagram p10: hidden frame]
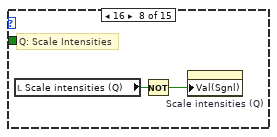
[diagram p11: hidden frame]
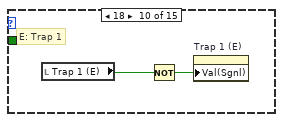
[diagram p13: hidden frame]
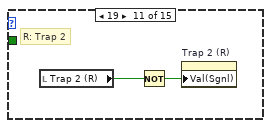
[diagram p14: hidden frame]
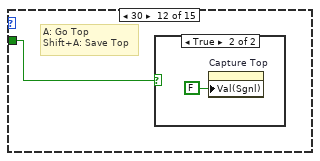
[diagram p15: hidden frame]
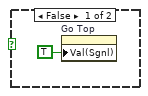
[diagram p16: hidden frame]
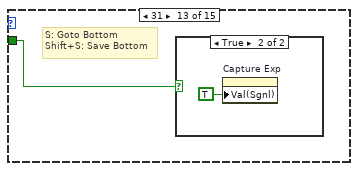
[diagram p17: hidden frame]
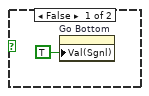
[diagram p18: hidden frame]
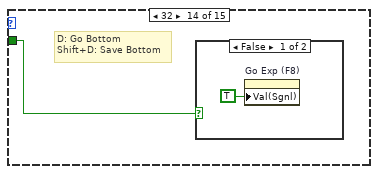
[diagram p19: hidden frame]
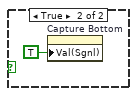
[diagram p20: hidden frame]
diagram:
  w10 = u16 0 items=["Off", "Approach", "Wiggle", "Extend", "Tether Found"] ("Fish Status")
  w74 = T15 2 items=["Grayscale (U8)", "Grayscale (I16)", "Grayscale (SGL)", "Complex (CSG)", "RGB (U32)", "HSL (U32)", "RGB (U64)", "Grayscale (U16)"] ("Image Type")
  w193 = 10.0 ("y")
  w192 = 32767.0 ("y")
  w208 = 6.0  # clock mult.
  w209 = 49152000.0  # TCXO frequ.
  # "~Do stuff on close~\nMove stage to 000\nCollect, display errors\nTurn off FPGA\nFlip green filter\nSave Locations"
  # "Orphaned Controls"
  n1 = flat-sequence "FPGA bitfile init" {
    tunnel: [w244] -> w30
    tunnel: w30 -> [w255]
    tunnel: [w249] -> w140
    tunnel: [w248] -> w124
    frame #0 {
      w244 = T16 "RIO0" ("resource name")
      n2 = xnode "Open FPGA VI Reference"("resource name"=w244) -> ("FPGA VI Reference Out"=w247:T17)  [unwired: 1 in, 1 out]
      n3 = xnode "Invoke Method"("FPGA VI Reference In"=w247) -> ("FPGA VI Reference Out"=w246:T17, "error out"=w245:errorcluster)  [unwired: 1 in]
      n4 = xnode "Invoke Method"("FPGA VI Reference In"=w246, "error in"=w245) -> ("FPGA VI Reference Out"=w243:T17, "error out"=w240:errorcluster)  [unwired: 1 in]
      n5 = call "Initialize RF boards - with FPGA init only vi v1_debugalex.vi"("error in"=w240, "FPGA Interface"=w243) -> ("error out"=w241:errorcluster, "FPGA Interface 2"=w242:T17)
      n6 = xnode "Close FPGA VI Reference"("FPGA VI Reference In"=w242, "error in"=w241) -> ()  [unwired: 1 out]
    }
    frame #1 {
      w250 = TRUE
      n7 = xnode "Open FPGA VI Reference"("resource name"=w255) -> ("FPGA VI Reference Out"=w254:T18, "error out"=w253:errorcluster)  [unwired: 1 in]
      n8 = xnode "Invoke Method"("FPGA VI Reference In"=w254, "error in"=w253) -> ("FPGA VI Reference Out"=w252:T18, "error out"=w251:errorcluster)
      n9 = xnode "Read/Write Control"("FPGA VI Reference In"=w252, "error in"=w251, "PMODE"=w250, "RD"=w250) -> ("FPGA VI Reference Out"=w248:T18, "error out"=w249:errorcluster)
      "FPGA error out" <- w249
    }
  }
  n10 = Build Array("DIO count 1 (ticks)", "DIO count 2 (ticks)", "DIO count 3 (ticks)") -> (w116:u32[])
  n11 = Multiply(x="APD Integration Time (s)", y=40000000.0) -> (x*y=w131:dbl)
  n12 = local read "MCL Y"() -> (w187:dbl)
  n13 = local read "MCL X"() -> (w186:dbl)
  n14 = To Unsigned Long Integer(number=w131) -> (unsigned 32bit integer=w130:u32)
  n15 = local read "Dynamic Force FB"() -> (w32:bool)
  n16 = local read "Negate Diff?"() -> (w31:bool)
  n17 = local read "Diff. FB."() -> (w33:bool)
  n18 = local read "Continuous MCL Scanning"() -> (w174:bool)
  n19 = local read "Scan Step (MHz)"() -> (w204:dbl)
  n20 = local read "Fast Scan Dir"() -> (w173:bool)
  n21 = local read "Number of scans (MCL)"() -> (w175:u64)
  n22 = Multiply(x=w187, y=w192) -> (x*y=w189:dbl)
  n23 = Multiply(x=w186, y=w192) -> (x*y=w191:dbl)
  n24 = local read "Trap Powers (V)"() -> (w218:cluster{"Set 1":dbl, "Set 2":dbl})
  n25 = Divide(x=w189, y=w193) -> (x/y=w188:dbl)
  n26 = Divide(x=w191, y=w193) -> (x/y=w190:dbl)
  n27 = flat-sequence "Set RF Freq/Amp Limits" {
    tunnel: w124 -> [w260]
    tunnel: [w260] -> w123
    tunnel: [w257] -> w34
    tunnel: [w259] -> w122
    tunnel: [w256] -> w120
    tunnel: [w258] -> w121
    frame #0 {
      w258 = T13 {"Minimum"=60.0, "Maximum"=90.0, "Increment"=1.0} ("Min Max Inc")
      w256 = T13 {"Minimum"=0.0, "Maximum"=75.0, "Increment"=1.0} ("Data Entry Limits")
      w257 = T13 {"Minimum"=60.0, "Maximum"=90.0, "Increment"=1.0} ("Min Max Inc")
      w259 = T13 {"Minimum"=0.0, "Maximum"=75.0, "Increment"=1.0} ("Data Entry Limits")
      n28 = property on="BD 1 Frq 1 (MHz)" class="DigNum (strict)"("Data Range"=w257) -> ()  [unwired: 2 in, 2 out]
      n29 = property on="BD 1 Frq 2 (MHz)" class="DigNum (strict)"("Data Range"=w257) -> ()  [unwired: 2 in, 2 out]
      n30 = property on="BD 1 Frq 3 (MHz)" class="DigNum (strict)"("Data Range"=w257) -> ()  [unwired: 2 in, 2 out]
      n31 = property on="BD 2 Frq 1 (MHz)" class="DigNum (strict)"("Data Range"=w258) -> ()  [unwired: 2 in, 2 out]
      n32 = property on="BD 2 Frq 2 (MHz)" class="DigNum (strict)"("Data Range"=w258) -> ()  [unwired: 2 in, 2 out]
      n33 = property on="BD 2 Frq 3 (MHz)" class="DigNum (strict)"("Data Range"=w258) -> ()  [unwired: 2 in, 2 out]
      n34 = property on="BD 1 Amp 1 (%)" class="DigNum (strict)"("Data Range"=w259) -> ()  [unwired: 2 in, 2 out]
      n35 = property on="BD 1 Amp 2 (%)" class="DigNum (strict)"("Data Range"=w259) -> ()  [unwired: 2 in, 2 out]
      n36 = property on="BD 1 Amp 3 (%)" class="DigNum (strict)"("Data Range"=w259) -> ()  [unwired: 2 in, 2 out]
      n37 = property on="BD 2 Amp 1 (%)" class="DigNum (strict)"("Data Range"=w256) -> ()  [unwired: 2 in, 2 out]
      n38 = property on="BD 2 Amp 2 (%)" class="DigNum (strict)"("Data Range"=w256) -> ()  [unwired: 2 in, 2 out]
      n39 = property on="BD 2 Amp 3 (%)" class="DigNum (strict)"("Data Range"=w256) -> ()  [unwired: 2 in, 2 out]
      "X RF Freq Limits (MHz)" <- w257
      "X RF Amp Limits (%)" <- w259
      "Y RF Amplitude Limits (%)" <- w256
      "Y RF Frequency Limits (MHz)" <- w258
    }
  }
  n40 = To Word Integer(number=w188) -> (16bit integer=w185:i16)
  n41 = To Word Integer(number=w190) -> (16bit integer=w184:i16)
  n42 = Not(x=w173) -> (.not. x?=w169:bool)
  n43 = local read "Cycles/step (MCL)"() -> (w176:u64)
  n44 = Multiply(x=w204, y=1000.0) -> (x*y=w211:dbl)
  n45 = local write "Trap Pos FIFO Timeout"(u16 0 ("Trap Pos FIFO Timeout")) -> ()
  n46 = local read "Scan steps (x)"() -> (w177:u64)
  n47 = local read "Desired Scan Incr (V)"() -> (w179:dbl)
  n48 = Scale By Power Of 2(n=48, x=w211) -> (x*2^n=w212:dbl)
  n49 = local read "Sets to FIFO (Traps)"() -> (w29:T12)
  n50 = Multiply(x=w209, y=w208) -> (x*y=w207:dbl)
  n51 = Divide(x=w212, y=w207) -> (x/y=w206:dbl)
  n52 = local read "Number Interlace Sets"() -> (w109:u8)
  n53 = Split 1D Array(array=w116, index=w109) -> (first subarray=w118:u32[])  [unwired: 1 out]
  n54 = Add Array Elements(numeric array=w118) -> (sum=w117:u32)
  n55 = property on="AI Count (ticks)" class="DigNum (strict)"("Val(Sgnl)"="AI Count (ticks)") -> ()  [unwired: 2 in, 2 out]
  n56 = local read "# Samples/channel"() -> (w196:u32)
  n57 = To Quad Integer(1:w206) -> (0:w203:i64)
  n58 = local read "Not-Interlacing Set"() -> (w108:enum32{"Set 1", "Set 2", "Set 3"})
  n59 = To Unsigned Byte Integer(number=w108) -> (unsigned 8bit integer=w114:u8)
  n60 = Index Array(array=w116, index=w114) -> (element=w115:u32)
  n61 = local read "Feedback On/Off"() -> (w221:cluster{"Set 1":bool, "Set 2":bool})
  n62 = local read "N F/B Scans (AOD)"() -> (w197:u16)
  n63 = Divide(x=40000000.0, y="AI Count (ticks)") -> (x/y=w166:dbl)
  n64 = Multiply(x=w179, y=32767.0) -> (x*y=w181:dbl)
  n65 = local read "Scan steps (AOD)"() -> (w202:u64)
  n66 = local read "All FB On/Off"() -> (w222:bool)
  n67 = local read "Cycles/step (AOD)"() -> (w201:u64)
  n68 = local write "AI rate (Hz)"(w166) -> ()
  n69 = Divide(x=w181, y=10.0) -> (x/y=w180:dbl)
  n70 = Multiply(x=w202, y=w201) -> (x*y=w200:u64)
  n71 = Multiply(x=3276.7, y=w218) -> (x*y=w217:cluster{"Set 1":dbl, "Set 2":dbl})
  n72 = To Word Integer(number=w180) -> (16bit integer=w178:i16)
  n73 = Multiply(x=w200, y=u64 2) -> (x*y=w198:u64)
  n74 = Divide(x=w166, y="FPGA Ave.") -> (x/y=w167:dbl)
  n75 = To Word Integer(number=w217) -> (16bit integer=w216:cluster{"Set 1":i16, "Set 2":i16})
  n76 = Multiply(x=w198, y=w197) -> (x*y=w195:u64)
  n77 = Divide(x=w195, y=w196) -> (x/y=w194:dbl)
  n78 = Unbundle By Name(w29) -> ("Set 1"=w28:bool, "Set 2"=w27:bool, "Set 3"=w26:bool)
  n79 = Unbundle By Name(w216) -> ("Set 1"=w215:i16, "Set 2"=w214:i16)
  n80 = local read "2D or 1D Scan"() -> (w126:bool)
  n81 = local read "Scan BD"() -> (w213:bool)
  n82 = And(x=w221, y=w222) -> (x .and. y?=w220:cluster{"Set 1":bool, "Set 2":bool})
  n83 = Reciprocal(x=w167) -> (1/x=w168:dbl)
  n84 = local read "N Acq Sets (Traps + Fl.)"() -> (w160:i16)
  n85 = local write "Trap Raster N Sets"(w194) -> ()
  n86 = Unbundle By Name(w220) -> ("Set 1"=w224:bool, "Set 2"=w223:bool)
  n87 = local read "Interlace"() -> (w110:bool)
  n88 = Select(t=w117, s=w110, f=w115) -> (s? t:f=w107:u32)
  n89 = local write "Update Count (MCL)"(w107) -> ()
  n90 = local write "Total Counts (ticks)"(w107) -> ()
  n91 = local write "Ave. Period (s)"(w168) -> ()
  n92 = property on="2D or 1D Scan" class="Bool (strict)"("Val(Sgnl)"=w126) -> ()  [unwired: 2 in, 2 out]
  n93 = xnode "Read/Write Control"("FPGA VI Reference In"=w123, "error in"=w140, "ai count"="AI Count (ticks)", "Interlace ON/OFF"=w110, "Number Interlace Cycles"=w109, "Set 1"=w28, "Set 2"=w27, "Set 3"=w26, "FB On/Off Set 1"=w224, "FB On/Off Set 2"=w223, "Interlace Off Parameters"=w108, "FB Setpoint Set 1"=w215, "FB Setpoint Set 2"=w214, "FB Gains"="PID gains", "FB output range"=cluster{"output high":i16, "output low":i16} {"output high"=3000, "output low"=0} ("FB output range 1"), "Cycles per step"=w201, "Scan BD"=w213, "Number of scans"=w197, "Scan steps"=w202, "Scan freq.  increment"=w203, "AO1 (Y)"=w185, "AO2 (X)"=w184, "Scan freq.  increment (MCL)"=w178, "Scan steps (MCL)"=w177, "Cycles per step (MCL)"=w176, "Number of scans (MCL)"=w175, "MCL count"=w107, "Cont. Scan (MCL)"=w174, "MCL Scan Axis"=w169, "1D or 2D Scan?"=w126, "N of AI1 Int Acq Sets"=w160, "BD 1 Delay (ticks)"="Freq switch delay", "Amp switch delay"="Amp switch delay", "Swap F1 and F2"="Swap F1 and F2", "APD Acq Rate Count"=w130, "APD to FIFO"=FALSE, "APD Gate Operating Mode"="APD Gate", "APD Gate ON Count"="APD Gate ON Count", "APD Gate OFF Count"="APD Gate OFF Count", "Invert APD Gate"="Invert APD Gate", "DIO count 1 (ticks)"="DIO count 1 (ticks)", "DIO count 2 (ticks)"="DIO count 2 (ticks)", "DIO count 3 (ticks)"="DIO count 3 (ticks)", "APD 1 AO scale factor"="APD 1 AO Mult.", "APD 2 AO scale factor"="APD 2 AO Mult.", "Diff FB Measurement?"=w33, "Dynamic Force FB (Ronen)"=w32, "Negate Diff?"=w31, "Next trap write delay (ticks)"="Next trap write delay (ticks)", "Phase offset method"="Phase offset method", "Phase Trap 1"="Phase increment trap 1", "RF phase reset before cycles"="RF phase reset before cycles", "Phase Trap 2"="Phase increment trap 2") -> ("FPGA VI Reference Out"=w102:T18, "error out"=w104:errorcluster)  [unwired: 1 in]
  n94 = local read "Green laser mode"() -> (w106:enum32{"Laser ON", "Laser OFF", "Interlace"})
  n95 = local read "Green Laser"() -> (w105:bool)
  n96 = local read "GI Frequency, OFF count"() -> (w98:u32)
  n97 = local read "GI Frequency, ON count"() -> (w97:u32)
  n98 = Multiply(x="Current (%)", y=655.35) -> (x*y=w89:dbl)
  n99 = local read "Green FB Count"() -> (w96:u32)
  n100 = Multiply(x="Green FB Setpoint (mV)", y=3.2767) -> (x*y=w86:dbl)
  n101 = To Unsigned Word Integer(number=w89) -> (unsigned 16bit integer=w87:u16)
  n102 = local read "Invert GI"() -> (w100:bool)
  n103 = To Word Integer(number=w86) -> (16bit integer=w84:i16)
  n104 = case shown="True" w105 {
    tunnel: w106 -> [_ w262]
    tunnel: [enum32{"Laser ON", "Laser OFF", "Interlace"}."Laser OFF" ("Green laser mode") w262] -> w99
    frame False {
    }
    frame True {
    }
  }
  n105 = local read "Trap Pos. AI1 X Pre-scale"() -> (w58:u16)
  n106 = local read "Trap Pos FB Monitor\nT1 or T2"() -> (w65:bool)
  n107 = local read "Trap Pos FB Int Count"() -> (w55:u16)
  n108 = local read "Trap Pos FB Negate Action"() -> (w64:bool)
  n109 = local read "Trap Pos. FB Offset Factor"() -> (w63:i64)
  n110 = local read "Trap Pos. FB Mult Factor"() -> (w62:i64)
  n111 = local read "Trap Pos. FB Gains"() -> (w60:T7)
  n112 = local read "Trap Pos. FB Range"() -> (w61:T8)
  n113 = xnode "Read/Write Control"("FPGA VI Reference In"=w102, "error in"=w104, "Green interlace ON count 2"=w97, "Green interlace OFF count 2"=w98, "Invert GI 2"=w100, "Operating Mode 2"=w99, "Green FB Gains"="Green FB Gains", "Green FB Setpoint"=w84, "Green FB On/Off"="Green FB On/Off", "Current Out"=w87, "Green int current ON count adj"="Green int current ON count adj", "Green FB Count"=w96, "Operating Mode"=w99, "Green interlace OFF count"=w98, "Green interlace ON count"=w97, "Invert GI"=w100, "Trap Pos FB Monitor T1 or T2"=w65, "Trap Pos FB Negate Action"=w64, "Trap Pos. FB Offset Factor"=w63, "Trap Pos. FB Mult Factor"=w62, "Trap pos. FB Range"=w61, "Trap Pos. FB Gains"=w60, "Force feedback"=FALSE, "AI1 X Scale"=w58, "Trap Pos to FIFO"=TRUE, "Trap Pos FB Int Count"=w55) -> ("FPGA VI Reference Out"=w101:T18, "error out"=w103:errorcluster)
  n114 = xnode "Invoke Method"("FPGA VI Reference In"=w101, "error in"=w103, "Requested Depth"="Trap AI FIFO Depth") -> ("FPGA VI Reference Out"=w68:T18, "error out"=w67:errorcluster)  [unwired: 1 out]
  n115 = xnode "Invoke Method"("FPGA VI Reference In"=w68, "error in"=w67, "Requested Depth"="Trap Position FIFO Depth") -> ("FPGA VI Reference Out"=w16:T18, "error out"=w14:errorcluster)  [unwired: 1 out]
  n116 = xnode "Invoke Method"("FPGA VI Reference In"=w16, "error in"=w14, "Requested Depth"="APD FIFO Depth (requires restart)") -> ("FPGA VI Reference Out"=w15:T18, "error out"=w13:errorcluster)  [unwired: 1 out]
  n117 = xnode "Invoke Method"("FPGA VI Reference In"=w15, "error in"=w13) -> ("FPGA VI Reference Out"=w44:T18, "error out"=w43:errorcluster)  [unwired: 1 in]
  n118 = flat-sequence "Initial FPGA Loop Relative Phase Adjustment" {
    tunnel: w43 -> [w264]
    tunnel: w44 -> [w265]
    tunnel: [w265] -> w48
    tunnel: [w264] -> w47
    tunnel: [w277] -> w146
    tunnel: [w274] -> w144
    tunnel: w48 -> [w276]
    tunnel: w47 -> [w275]
    tunnel: w146 -> [w279]
    tunnel: [w280] -> w145
    tunnel: w144 -> [w280]
    tunnel: [w279] -> w143
    tunnel: w145 -> [w283]
    tunnel: w143 -> [w282]
    tunnel: [w285] -> w142
    tunnel: [w284] -> w141
    tunnel: [w287] -> w42
    tunnel: [w288] -> w45
    tunnel: w142 -> [w288]
    tunnel: w141 -> [w287]
    frame #0 {
      n119 = Wait (ms)(milliseconds to wait=u32 1000) -> ()  [unwired: 1 out]
    }
    frame #1 {
      n120 = xnode "Read/Write Control"("FPGA VI Reference In"=w276, "error in"=w275, "Phase count adjustment"="Initial Phase Adjustment (AI1)", "Phase count adjustment (GI)"="Initial Phase Adjustment (GI)", "Phase count adjustment (MCL)"="Initial Phase Adj. (MCL)", "Phase Count Adjustment (APD Acq)"="Initial Phase Adjustment (APD Acq)", "Phase count adjustment (APD 1 Gate)"="Initial Phase Adjustment (APD 1 Gate)", "Phase count adjustment (APD 2 Gate)"="Initial Phase Adjustment (APD 2 Gate)", "Phase count adjustment (Green FB)"="Initial Phase Adjustment (Green FB)", "Phase count adjustment (GI) 2"="Initial Phase Adjustment (GI) 2") -> ("FPGA VI Reference Out"=w274:T18, "error out"=w277:errorcluster)
    }
    frame #2 {
      n121 = Wait (ms)(milliseconds to wait=u32 1000) -> ()  [unwired: 1 out]
    }
    frame #3 {
      w281 = TRUE
      n122 = xnode "Read/Write Control"("FPGA VI Reference In"=w283, "error in"=w282, "+ phase"=w281, "+ phase (GI)"=w281, "+ phase (MCL)"=w281, "+ phase (APD Acq)"=w281, "+ phase (APD 1 Gate)"=w281, "+ phase (APD 2 Gate)"=w281, "+ phase (Green FB)"=w281, "+ phase (GI) 2"=w281) -> ("FPGA VI Reference Out"=w284:T18, "error out"=w285:errorcluster)
    }
    frame #4 {
      n123 = Wait (ms)(milliseconds to wait=u32 1000) -> ()  [unwired: 1 out]
    }
  }
  n124 = local read "Phase adj. (AI1)"() -> (w172:i16)
  n125 = local read "Phase adj. (GI)"() -> (w171:i16)
  n126 = local read "Phase adjust (MCL)"() -> (w170:i16)
  n127 = local read "Phase adj. (Green FB)"() -> (w119:i16)
  n128 = local read "Phase adj. (GI) 2"() -> (w90:i16)
  n129 = xnode "Read/Write Control"("FPGA VI Reference In"=w42, "error in"=w45, "Phase count adjustment"=w172, "Phase count adjustment (GI)"=w171, "Phase count adjustment (MCL)"=w170, "Phase Count Adjustment (APD Acq)"="Phase Adj. (APD Acq)", "Phase count adjustment (APD 1 Gate)"="Phase Adj. (APD 1 Gate)", "Phase count adjustment (APD 2 Gate)"="Phase Adj. (APD 2 Gate)", "Phase count adjustment (Green FB)"=w119, "Phase count adjustment (GI) 2"=w90) -> ("FPGA VI Reference Out"=w24:T18, "error out"=w23:errorcluster)
  n130 = Unbundle By Name(w34) -> ("Minimum"=w9:dbl, "Maximum"=w7:dbl)
  n131 = call "MHz2uint64.vi"("inMHz"=w9) -> ("outu64"=w8:u64)  [unwired: 4 in]
  n132 = call "MHz2uint64.vi"("inMHz"=w7) -> ("outu64"=w6:u64)  [unwired: 4 in]
  n133 = xnode "Read/Write Control"("FPGA VI Reference In"=w24, "FB Min frequency"=w8, "FB Max Frequency"=w6) -> ()  [unwired: 1 in, 2 out]
  n134 = call "set RF board frequency - interlace.vi"("Board 2 Frequency Limits"=w121, "Board 1 Frequency Limits"=w34, "error in"=w23, "FPGA VI Reference In"=w24, "Board 2 Frequency 3 (MHz)"="BD 2 Frq 3 (MHz)", "Board 1 Frequency 3 (MHz)"="BD 1 Frq 3 (MHz)", "Board 2 Frequency 2 (MHz)"="BD 2 Frq 2 (MHz)", "Board 2 Frequency 1 (MHz)"="BD 2 Frq 1 (MHz)", "Board 1 Frequency 2 (MHz)"="BD 1 Frq 2 (MHz)", "Board 1 Frequency 1  (MHz)"="BD 1 Frq 1 (MHz)") -> ("error out"=w235:errorcluster, "FPGA VI Reference Out"=w236:T18)
  n135 = Subtract(x="BD 1 Frq 1 (MHz)", y="BD 1 Frq 2 (MHz)") -> (x-y=w159:dbl)
  n136 = Subtract(x="BD 2 Frq 1 (MHz)", y="BD 2 Frq 2 (MHz)") -> (x-y=w158:dbl)
  n137 = Square(x=w158) -> (x^2=w156:dbl)
  n138 = Square(x=w159) -> (x^2=w157:dbl)
  n139 = Add(x=w157, y=w156) -> (x+y=w155:dbl)
  n140 = Square Root(x=w155) -> (sqrt(x)=w154:dbl)
  n141 = call "set RF board amplitude - interlace.vi"("Board 2 Amplitude Limits"=w120, "Board 1 Amplitude Limits"=w122, "error in"=w235, "FPGA VI Reference In"=w236, "Board 2 Amplitude 3 (%)"="BD 2 Amp 3 (%)", "Board 1 Amplitude 3 (%)"="BD 1 Amp 3 (%)", "Board 2 Amplitude 2 (%)"="BD 2 Amp 2 (%)", "Board 2 Amplitude 1 (%)"="BD 2 Amp 1 (%)", "Board 1 Amplitude 2 (%)"="BD 1 Amp 2 (%)", "Board 1 Amplitude 1 (%)"="BD 1 Amp 1 (%)") -> ("error out"=w40:errorcluster, "FPGA VI Reference Out"=w41:T18)
  n142 = local write "Trap Delta (MHz)"(w154) -> ()
  n143 = flat-sequence {
    tunnel: w41 -> [w290]
    tunnel: w40 -> [w289]
    tunnel: [w290] -> w228
    tunnel: [w289] -> w227
    tunnel: [w298] -> w226
    tunnel: w228 -> [w298]
    tunnel: [w297] -> w225
    tunnel: w227 -> [w297]
    tunnel: w226 -> [w301]
    tunnel: w225 -> [w300]
    tunnel: [w301] -> w36
    tunnel: [w300] -> w35
    tunnel: [w307] -> w54
    tunnel: [w310] -> w46
    tunnel: w36 -> [w310]
    tunnel: w35 -> [w306]
    frame #0 {
      n144 = local write "Stop All"(FALSE ("Stop All")) -> ()
      n145 = local write "Saving..."(FALSE ("Saving Data")) -> ()
      n146 = local write "Index"(1.0 ("Index")) -> ()
      n147 = local read "Trap 1 (E)"() -> (w291:bool)
      n148 = property on="Trap 1 ON" class="Bool (strict)"("Value"=w291) -> ()  [unwired: 2 in, 2 out]
      "MouseMove Trap" <- FALSE ("Manipulating Trap")
    }
    frame #1 {
      n149 = local read "Trap 2 (R)"() -> (w296:bool)
      n150 = Wait (ms)(milliseconds to wait=u32 50) -> ()  [unwired: 1 out]
      n151 = property on="Trap 2 ON" class="Bool (strict)"("Val(Sgnl)"=w296) -> ()  [unwired: 2 in, 2 out]
    }
    frame #2 {
      n152 = local read "Scan Range (nm)"() -> (w302:dbl)
      n153 = call "Update messages.vi"("Message to add"="UHR-Fleezers ready.", "Old message string"="") -> ()  [unwired: 1 out]
      n154 = property on="Scan Range (nm)" class="DigNum (strict)"("Val(Sgnl)"=w302) -> ()  [unwired: 2 in, 2 out]
    }
    frame #3 {
      n155 = call "hamilton_controller_shunt2.vi"("error in"=w306, "action"=T19."CONNECT") -> ("error out"=w308:errorcluster)  [unwired: 9 in]
      n156 = case shown="True" "Init Valve?" {
        tunnel: w308 -> [w311 w314]
        tunnel: [w311 w313] -> w307
        frame False {
        }
        frame True {
          n157 = local write "Init Valve?"(FALSE ("Reinit Valve?")) -> ()
          n158 = call "hamilton_controller_shunt2.vi"("error in"=w314, "action"=T19."INITIALIZE VALVES") -> ("error out"=w313:errorcluster)  [unwired: 9 in]
        }
      }
    }
  }
  n159 = call "IMAQ Create"("Image Name"="APD 1 Image", "Image Type"=w74) -> ("New Image"=w73:T2)  [unwired: 3 in, 1 out]
  n160 = call "IMAQ Create"("Image Name"="APD 2 Image", "Image Type"=w74) -> ("New Image"=w72:T2)  [unwired: 3 in, 1 out]
  n161 = call "IMAQ Create"("Image Name"="Det. X Image", "Image Type"=w74) -> ("New Image"=w71:T2)  [unwired: 3 in, 1 out]
  n162 = call "IMAQ Create"("Image Name"="Det. Y Image", "Image Type"=w74) -> ("New Image"=w70:T2)  [unwired: 3 in, 1 out]
  n163 = Bundle("New Image"=w73, "New Image"=w72, "New Image"=w71, "New Image"=w70) -> (w69:T20)  [unwired: 1 in]
  n164 = node-c288() -> (w78:T21)  [unwired: 4 in]
  n165 = call <vilib>:"Initialize Mouse.vi"() -> ("device ID"=w1:refnum<k1>)  [unwired: 10 in, 1 out]
  n166 = node-c288(2 ("Processor")) -> (w39:T21)  [unwired: 3 in]
  n167 = node-c288(i64 1 ("Period"), 1 ("Processor")) -> (w162:T21)  [unwired: 2 out]
  n168 = node-c288() -> (w83:T21)
  n169 = case shown="False" "NoStage?" {
    frame False {
      n170 = while "Stage Control" {
        shift-right: [w319] -> w317
        shift-left: errorcluster {"status"=FALSE, "code"=0, "source"=""} ("error out") -> [w318]
        stop <- w320 stop-if-true
        n171 = event shown="[3] \"Goto Bottom (F7)\": Value Change" {
          selector: _ -> [_ _ _ _ _ _ _ _ _ _]
          dyn-events: _ -> [_ _ _ _ _ _ _ _ _ _]
          timeout: 10 -> [_ _ _ _ _ _ _ _ _ _]
          tunnel: [FALSE _ _ _ _ _ _ _ _ TRUE] -> w320
          tunnel: w318 -> [w323 _ _ _ _ _ _ _ _ _]
          tunnel: [w322 _ _ _ _ _ _ _ _ _] -> w319
          event Timeout {
            # "Change the trajectory mode to Jog"
            # "Query and display stage positions"
            # "Setting ESP300 left and right limits for Z-axis, input in mm"
            n172 = event-data() -> ()  [unwired: 1 in, 2 out]
            n173 = Concatenate Strings("1TP;\n2TP;\n3TP;\n1MD?;\n2MD?;\n3MD?" ("Substring"), "\r") -> (w331:string)
            n174 = local read "ESP Port"() -> (w334:refnum<visa-resource-name>)
            n175 = local read "ESP Port"() -> (w341:refnum<visa-resource-name>)
            n176 = VISA Write(VISA resource name=w334, write buffer=w331, error in (no error)=w323) -> (VISA resource name out=w332:refnum<visa-resource-name>, error out=w330:errorcluster)  [unwired: 1 out]
            n177 = Concatenate Strings("3SL" ("Substring"), "ESP ZL-Limit", ";3SR", "ESP ZR-Limit", "\r") -> (w340:string)
            n178 = case shown="True" TRUE ("Case Constant\n(See Context Help)") {
              tunnel: w332 -> [_ w362]
              tunnel: w330 -> [w343 w361]
              tunnel: [w343 w345] -> w322
              frame False {
              }
              frame True {
                w355 = u16 10 items=["1.0"=10, "1.5"=15, "2.0"=20] ("Serial Settings:Stop Bits")
                w356 = u16 0 items=["None", "Odd", "Even", "Mark", "Space"] ("Serial Settings:Parity")
                n179 = property class="Instr"(reference=w362, error in=w361, "Baud"=u32 921600 ("Serial Settings:Baud Rate"), "Data Bits"=u16 8 ("Serial Settings:Data Bits"), "Parity"=w356, "Stop Bits"=w355) -> (reference out=w360:refnum<visa-resource-name>, error out=w359:errorcluster, "Bytes at Port"=w344:u32)
                n180 = Wait (ms)(milliseconds to wait=u32 10) -> ()  [unwired: 1 out]
                n181 = VISA Read(VISA resource name=w360, byte count=w344, error in (no error)=w359) -> (VISA resource name out=w368:refnum<visa-resource-name>, read buffer=→"X Pos":string, error out=w369:errorcluster)  [unwired: 1 out]
                n182 = VISA Read(VISA resource name=w368, byte count=w344, error in (no error)=w369) -> (VISA resource name out=w366:refnum<visa-resource-name>, read buffer=→"Y Pos":string, error out=w367:errorcluster)  [unwired: 1 out]
                n183 = VISA Read(VISA resource name=w366, byte count=w344, error in (no error)=w367) -> (VISA resource name out=w354:refnum<visa-resource-name>, read buffer=→"Z Pos Pos":string, error out=w353:errorcluster)  [unwired: 1 out]
                n184 = VISA Read(VISA resource name=w354, byte count=w344, error in (no error)=w353) -> (VISA resource name out=w350:refnum<visa-resource-name>, read buffer=→"X Motion":string, error out=w351:errorcluster)  [unwired: 1 out]
                n185 = VISA Read(VISA resource name=w350, byte count=w344, error in (no error)=w351) -> (VISA resource name out=w349:refnum<visa-resource-name>, read buffer=→"Y Motion":string, error out=w347:errorcluster)  [unwired: 1 out]
                n186 = VISA Read(VISA resource name=w349, byte count=w344, error in (no error)=w347) -> (read buffer=→"Z motion":string, error out=w345:errorcluster)  [unwired: 2 out]
              }
            }
            n187 = VISA Write(VISA resource name=w341, write buffer=w340) -> ()  [unwired: 1 in, 3 out]
            n188 = local read "ESP Port"() -> (w324:refnum<visa-resource-name>)
            n189 = Concatenate Strings("1TJ3;\n2TJ3;\n3TJ3" ("Substring"), "\r") -> (w325:string)
            n190 = VISA Write(VISA resource name=w324, write buffer=w325) -> ()  [unwired: 1 in, 3 out]
          }
          event "Goto Top": Value Change {
            n191 = event-data() -> ()  [unwired: 1 in, 5 out]
            n192 = local write "Goto Top"(FALSE ("Goto Top (F6)")) -> ()
            n193 = stacked-sequence {
              frame #0 {
                # "stop motions of all axes before going to avoid reversing of direction"
                n194 = local read "ESP Port"() -> (w375:refnum<visa-resource-name>)
                n195 = Concatenate Strings("ST" ("Substring"), "\r") -> (w372:string)
                n196 = VISA Write(VISA resource name=w375, write buffer=w372) -> ()  [unwired: 1 in, 3 out]
              }
              frame #1 {
                n197 = Wait (ms)(milliseconds to wait=u32 50) -> ()  [unwired: 1 out]
              }
              frame #2 {
                # "Change the trajectory mode to Trapezoidal"
                n198 = local read "ESP Port"() -> (w380:refnum<visa-resource-name>)
                n199 = Concatenate Strings("1TJ1;\n2TJ1;\n3TJ1" ("Substring"), "\r") -> (w377:string)
                n200 = VISA Write(VISA resource name=w380, write buffer=w377) -> ()  [unwired: 1 in, 3 out]
              }
              frame #3 {
                # "Go to Top Dispensor"
                n201 = local read "Locations"() -> (w392:string[][])
                n202 = Index Array(array=w392, index (row)=0) -> (element=w388:string[])  [unwired: 1 in]
                n203 = Decimate 1D Array(w388) -> (w386:string[], w384:string[], w382:string[])
                n204 = local read "ESP Port"() -> (w389:refnum<visa-resource-name>)
                n205 = Concatenate Strings("1PA" ("Substring"), w386, "2PA" ("Substring"), w384, "3PA" ("Substring"), w382, "\r") -> (w390:string)
                n206 = VISA Write(VISA resource name=w389, write buffer=w390) -> ()  [unwired: 1 in, 3 out]
              }
              frame #4 {
                n207 = Wait (ms)(milliseconds to wait=u32 100) -> ()  [unwired: 1 out]
              }
              frame #5 {
                # "Change the trajectory mode to Jog"
                n208 = local read "ESP Port"() -> (w397:refnum<visa-resource-name>)
                n209 = Concatenate Strings("1TJ3;\n2TJ3;\n3TJ3" ("Substring"), "\r") -> (w394:string)
                n210 = VISA Write(VISA resource name=w397, write buffer=w394) -> ()  [unwired: 1 in, 3 out]
              }
            }
          }
          event "Goto Exp (F8)": Value Change {
            n211 = event-data() -> ()  [unwired: 1 in, 5 out]
            n212 = local write "Goto Exp (F8)"(FALSE ("Goto Exp (F8)")) -> ()
            n213 = stacked-sequence {
              frame #0 {
                # "stop motions of all axes before going to avoid reversing of direction"
                n214 = local read "ESP Port"() -> (w402:refnum<visa-resource-name>)
                n215 = Concatenate Strings("ST" ("Substring"), "\r") -> (w399:string)
                n216 = VISA Write(VISA resource name=w402, write buffer=w399) -> ()  [unwired: 1 in, 3 out]
              }
              frame #1 {
                n217 = Wait (ms)(milliseconds to wait=u32 50) -> ()  [unwired: 1 out]
              }
              frame #2 {
                # "Change the trajectory mode to Trapezoidal"
                n218 = local read "ESP Port"() -> (w407:refnum<visa-resource-name>)
                n219 = Concatenate Strings("1TJ1;\n2TJ1;\n3TJ1" ("Substring"), "\r") -> (w404:string)
                n220 = VISA Write(VISA resource name=w407, write buffer=w404) -> ()  [unwired: 1 in, 3 out]
              }
              frame #3 {
                # "Go to Experimental"
                n221 = local read "Locations"() -> (w419:string[][])
                n222 = Index Array(array=w419, index (row)=2) -> (element=w415:string[])  [unwired: 1 in]
                n223 = Decimate 1D Array(w415) -> (w413:string[], w411:string[], w409:string[])
                n224 = Concatenate Strings("1PA" ("Substring"), w413, "2PA" ("Substring"), w411, "3PA" ("Substring"), w409, "\r") -> (w417:string)
                n225 = local read "ESP Port"() -> (w416:refnum<visa-resource-name>)
                n226 = VISA Write(VISA resource name=w416, write buffer=w417) -> ()  [unwired: 1 in, 3 out]
              }
              frame #4 {
                n227 = Wait (ms)(milliseconds to wait=u32 200) -> ()  [unwired: 1 out]
              }
              frame #5 {
                # "Change the trajectory mode to Jog"
                n228 = local read "ESP Port"() -> (w421:refnum<visa-resource-name>)
                n229 = Concatenate Strings("1TJ3;\n2TJ3;\n3TJ3" ("Substring"), "\r") -> (w424:string)
                n230 = VISA Write(VISA resource name=w421, write buffer=w424) -> ()  [unwired: 1 in, 3 out]
              }
            }
          }
          event "Goto Bottom (F7)": Value Change {
            n231 = event-data() -> ()  [unwired: 1 in, 5 out]
            n232 = local write "Goto Bottom (F7)"(FALSE ("Goto Bottom (F7)")) -> ()
            n233 = stacked-sequence {
              frame #0 {
                # "stop motions of all axes before going to avoid reversing of direction"
                n234 = local read "ESP Port"() -> (w429:refnum<visa-resource-name>)
                n235 = Concatenate Strings("ST" ("Substring"), "\r") -> (w426:string)
                n236 = VISA Write(VISA resource name=w429, write buffer=w426) -> ()  [unwired: 1 in, 3 out]
              }
              frame #1 {
                n237 = Wait (ms)(milliseconds to wait=u32 50) -> ()  [unwired: 1 out]
              }
              frame #2 {
                # "Change the trajectory mode to Trapezoidal"
                n238 = local read "ESP Port"() -> (w434:refnum<visa-resource-name>)
                n239 = Concatenate Strings("1TJ1;\n2TJ1;\n3TJ1" ("Substring"), "\r") -> (w431:string)
                n240 = VISA Write(VISA resource name=w434, write buffer=w431) -> ()  [unwired: 1 in, 3 out]
              }
              frame #3 {
                # "Go to Bottom Dispensor"
                n241 = local read "Locations"() -> (w446:string[][])
                n242 = Index Array(array=w446, index (row)=1) -> (element=w442:string[])  [unwired: 1 in]
                n243 = Decimate 1D Array(w442) -> (w440:string[], w438:string[], w436:string[])
                n244 = Concatenate Strings("1PA" ("Substring"), w440, "2PA" ("Substring"), w438, "3PA" ("Substring"), w436, "\r") -> (w444:string)
                n245 = local read "ESP Port"() -> (w443:refnum<visa-resource-name>)
                n246 = VISA Write(VISA resource name=w443, write buffer=w444) -> ()  [unwired: 1 in, 3 out]
              }
              frame #4 {
                n247 = Wait (ms)(milliseconds to wait=u32 200) -> ()  [unwired: 1 out]
              }
              frame #5 {
                # "Change the trajectory mode to Jog"
                n248 = local read "ESP Port"() -> (w448:refnum<visa-resource-name>)
                n249 = Concatenate Strings("1TJ3;\n2TJ3;\n3TJ3" ("Substring"), "\r") -> (w451:string)
                n250 = VISA Write(VISA resource name=w448, write buffer=w451) -> ()  [unwired: 1 in, 3 out]
              }
            }
          }
          event "Capture Top": Value Change {
            # "Capture Top Dispensor Location"
            n251 = event-data() -> ()  [unwired: 1 in, 5 out]
            n252 = local write "Capture Top"(FALSE ("Capture Top")) -> ()
            n253 = local read "Z Pos Pos"() -> (w457:string)
            n254 = local read "X Pos"() -> (w459:string)
            n255 = local read "Y Pos"() -> (w458:string)
            n256 = local read "Locations"() -> (w456:string[][])
            n257 = Build Array(w459, w458, w457) -> (w455:string[])
            n258 = Replace Array Subset(array=w456, new element=w455, index (row)=0) -> (w454:string[][])  [unwired: 1 in]
            n259 = local write "Locations"(w454) -> ()
          }
          event "Capture Bottom": Value Change {
            # "Capture Top Dispensor Location"
            n260 = event-data() -> ()  [unwired: 1 in, 5 out]
            n261 = local write "Capture Exp"(FALSE ("Capture Exp")) -> ()
            n262 = local read "Z Pos Pos"() -> (w465:string)
            n263 = local read "X Pos"() -> (w467:string)
            n264 = local read "Y Pos"() -> (w466:string)
            n265 = local read "Locations"() -> (w464:string[][])
            n266 = Build Array(w467, w466, w465) -> (w463:string[])
            n267 = Replace Array Subset(array=w464, new element=w463, index (row)=1) -> (w462:string[][])  [unwired: 1 in]
            n268 = local write "Locations"(w462) -> ()
          }
          event "Capture Exp": Value Change {
            # "Capture Top Dispensor Location"
            n269 = event-data() -> ()  [unwired: 1 in, 5 out]
            n270 = local write "Capture Exp"(FALSE ("Capture Exp")) -> ()
            n271 = local read "Z Pos Pos"() -> (w473:string)
            n272 = local read "X Pos"() -> (w475:string)
            n273 = local read "Y Pos"() -> (w474:string)
            n274 = local read "Locations"() -> (w472:string[][])
            n275 = Build Array(w475, w474, w473) -> (w471:string[])
            n276 = Replace Array Subset(array=w472, new element=w471, index (row)=2) -> (w470:string[][])  [unwired: 1 in]
            n277 = local write "Locations"(w470) -> ()
          }
          event "VISA Clear": Value Change {
            n278 = event-data() -> ()  [unwired: 1 in, 5 out]
            n279 = local read "ESP Port"() -> (w476:refnum<visa-resource-name>)
            n280 = VISA Clear(VISA resource name=w476) -> ()  [unwired: 1 in, 2 out]
          }
          event "Activate Joystick": Value Change {
            # "Change the trajectory mode to Jog"
            n281 = event-data() -> ()  [unwired: 1 in, 5 out]
            n282 = local read "ESP Port"() -> (w477:refnum<visa-resource-name>)
            n283 = Concatenate Strings("1TJ3;\n2TJ3;\n3TJ3" ("Substring"), "\r") -> (w480:string)
            n284 = VISA Write(VISA resource name=w477, write buffer=w480) -> ()  [unwired: 1 in, 3 out]
          }
          event "Stop All": Mouse Down {
            n285 = event-data() -> ()  [unwired: 1 in, 5 out]
          }
        }
      }
      "Error Stage" <- w317
    }
    frame True {
    }
  }
  n286 = timed-loop "Run Scripts, including: stage motion" {
    timing: w78 -> [_]
    timing-out: [_] -> w77
    tunnel: w46 -> [_]
    stop <- w483 stop-if-true
    n287 = node-c288() -> ()  [unwired: 1 in, 1 out]
    n288 = event shown="[1] \"Cal/Data Acq. Spot\": Value Change" {
      selector: _ -> [_ _ _ _ _ _]
      dyn-events: _ -> [_ _ _ _ _ _]
      timeout: 50 -> [_ _ _ _ _ _]
      tunnel: [_ "Cal/Data Acq. Spot" "Take Stepping Data" _ "Take Green\nLaser Image" _] -> _
      tunnel: [_ _ _ _ _ w643] -> w483
      event Timeout {
        n289 = event-data() -> ()  [unwired: 1 in, 2 out]
      }
      event "Cal/Data Acq. Spot": Value Change {
        # "CHANGE FISH FOR TETHER BACK\nTO TRUE VALUE HERE."
        n290 = event-data() -> ()  [unwired: 1 in, 5 out]
        n291 = flat-sequence {
          tunnel: ["Cal @ (MHz)"] -> w486
          tunnel: w486 -> [w498]
          tunnel: w486 -> [w519]
          frame #0 {
            n292 = property on="Trap Delta (MHz)" class="Slide (strict)"("Val(Sgnl)"="Cal @ (MHz)") -> ()  [unwired: 2 in, 2 out]
            n293 = call <vilib>:"Beep.vi"() -> ()  [unwired: 3 in, 9 out]
          }
          frame #1 {
            n294 = local read "Scale intensities (Q)"() -> (w490:bool)
            n295 = case shown="True" w490 {
              frame False {
              }
              frame True {
                n296 = property on="Scale intensities (Q)" class="Bool (strict)"("Val(Sgnl)"=FALSE ("Value (Signaling)")) -> ()  [unwired: 2 in, 2 out]
              }
            }
          }
          frame #2 {
            n297 = Wait (ms)(milliseconds to wait=u32 500) -> ()  [unwired: 1 out]
          }
          frame #3 {
            n298 = property on="Save Calibration" class="Bool (strict)"("Val(Sgnl)"=TRUE ("Value (Signaling)")) -> ()  [unwired: 2 in, 2 out]
          }
          frame #4 {
            n299 = Wait (ms)(milliseconds to wait=u32 4000) -> ()  [unwired: 1 out]
          }
          frame #5 {
            n300 = while {
              stop <- w495 stop-if-true
              n301 = local read "Saving..."() -> (w496:bool)
              n302 = Wait (ms)(milliseconds to wait=u32 100) -> ()  [unwired: 1 out]
              n303 = Not(x=w496) -> (.not. x?=w495:bool)
            }
          }
          frame #6 {
            n304 = case shown="True" "W/ Offset 1" {
              tunnel: w498 -> [_ w500]
              frame False {
              }
              frame True {
                n305 = stacked-sequence {
                  tunnel: w500 -> [_ _ _ _ _ _ _ w517]
                  frame #0 {
                    n306 = Replace Array Subset(array=u32[] [0] ("Index Values"), new element="Offset 1 Set", index=0) -> (w501:u32[])
                    n307 = property on="Saved AOD Raster Scan Parameter Sets" class="Arr (strict)"("Index Values"=w501) -> ()  [unwired: 2 in, 2 out]
                    n308 = property on="Trap Delta (MHz)" class="Slide (strict)"("Val(Sgnl)"="Offset 1 Start (MHz)") -> ()  [unwired: 2 in, 2 out]
                  }
                  frame #1 {
                    n309 = Wait (ms)(milliseconds to wait=u32 200) -> ()  [unwired: 1 out]
                  }
                  frame #2 {
                    n310 = property on="Load parameters" class="Bool (strict)"("Val(Sgnl)"=TRUE ("Value (Signaling)")) -> ()  [unwired: 2 in, 2 out]
                  }
                  frame #3 {
                    n311 = Wait (ms)(milliseconds to wait=u32 200) -> ()  [unwired: 1 out]
                  }
                  frame #4 {
                    n312 = property on="Trap Raster" class="Bool (strict)"("Val(Sgnl)"=TRUE ("Value (Signaling)")) -> ()  [unwired: 2 in, 2 out]
                  }
                  frame #5 {
                    n313 = Wait (ms)(milliseconds to wait=u32 2000) -> ()  [unwired: 1 out]
                  }
                  frame #6 {
                    n314 = while {
                      stop <- w514 stop-if-true
                      n315 = local read "Raster Scanning..."() -> (w516:bool)
                      n316 = local read "Saving..."() -> (w512:bool)
                      n317 = Wait (ms)(milliseconds to wait=u32 100) -> ()  [unwired: 1 out]
                      n318 = Not(x=w512) -> (.not. x?=w511:bool)
                      n319 = Not(x=w516) -> (.not. x?=w513:bool)
                      n320 = And(x=w513, y=w511) -> (x .and. y?=w514:bool)
                    }
                  }
                  frame #7 {
                    n321 = property on="Trap Delta (MHz)" class="Slide (strict)"("Val(Sgnl)"=w517) -> ()  [unwired: 2 in, 2 out]
                  }
                }
              }
            }
          }
          frame #7 {
            n322 = local read "Save ave N"() -> (w518:i32)
            n323 = case shown="True" "W/ Offset 2" {
              tunnel: w519 -> [_ w525]
              tunnel: w518 -> [_ w524]
              frame False {
                n324 = Multiply(x="Cal read wait (s)", y=u32 1000 ("milliseconds to wait")) -> (x*y=w522:u32)
                n325 = Wait (ms)(milliseconds to wait=w522) -> ()  [unwired: 1 out]
              }
              frame True {
                n326 = stacked-sequence {
                  tunnel: w525 -> [_ _ _ _ _ _ _ _ _ w546 _ _]
                  tunnel: w524 -> [_ _ _ _ _ _ _ _ _ w544 _ _]
                  frame #0 {
                    n327 = property on="Save ave N" class="DigNum (strict)"("Val(Sgnl)"=1.0 ("Value (Signaling)")) -> ()  [unwired: 2 in, 2 out]
                  }
                  frame #1 {
                    n328 = Wait (ms)(milliseconds to wait=u32 500) -> ()  [unwired: 1 out]
                  }
                  frame #2 {
                    n329 = property on="Trap Delta (MHz)" class="Slide (strict)"("Val(Sgnl)"="Offset 2 Start (MHz)") -> ()  [unwired: 2 in, 2 out]
                    n330 = Replace Array Subset(array=u32[] [0] ("Index Values"), new element="Offset 2 Set", index=0) -> (w530:u32[])
                    n331 = property on="Saved AOD Raster Scan Parameter Sets" class="Arr (strict)"("Index Values"=w530) -> ()  [unwired: 2 in, 2 out]
                  }
                  frame #3 {
                    n332 = Wait (ms)(milliseconds to wait=u32 500) -> ()  [unwired: 1 out]
                  }
                  frame #4 {
                    n333 = property on="Load parameters" class="Bool (strict)"("Val(Sgnl)"=TRUE ("Value (Signaling)")) -> ()  [unwired: 2 in, 2 out]
                  }
                  frame #5 {
                    n334 = Wait (ms)(milliseconds to wait=u32 500) -> ()  [unwired: 1 out]
                  }
                  frame #6 {
                    n335 = property on="Trap Raster" class="Bool (strict)"("Val(Sgnl)"=TRUE ("Value (Signaling)")) -> ()  [unwired: 2 in, 2 out]
                  }
                  frame #7 {
                    n336 = Wait (ms)(milliseconds to wait=u32 2000) -> ()  [unwired: 1 out]
                  }
                  frame #8 {
                    n337 = while {
                      stop <- w539 stop-if-true
                      n338 = local read "Raster Scanning..."() -> (w542:bool)
                      n339 = local read "Saving..."() -> (w540:bool)
                      n340 = Wait (ms)(milliseconds to wait=u32 100) -> ()  [unwired: 1 out]
                      n341 = Not(x=w540) -> (.not. x?=w538:bool)
                      n342 = Not(x=w542) -> (.not. x?=w541:bool)
                      n343 = And(x=w541, y=w538) -> (x .and. y?=w539:bool)
                    }
                  }
                  frame #9 {
                    n344 = property on="Trap Delta (MHz)" class="Slide (strict)"("Val(Sgnl)"=w546) -> ()  [unwired: 2 in, 2 out]
                    n345 = property on="Saved AOD Raster Scan Parameter Sets" class="Arr (strict)"("Index Values"=u32[] [0]) -> ()  [unwired: 2 in, 2 out]
                    n346 = property on="Save ave N" class="DigNum (strict)"("Val(Sgnl)"=w544) -> ()  [unwired: 2 in, 2 out]
                  }
                  frame #10 {
                    n347 = Wait (ms)(milliseconds to wait=u32 500) -> ()  [unwired: 1 out]
                  }
                  frame #11 {
                    n348 = property on="Load parameters" class="Bool (strict)"("Val(Sgnl)"=TRUE ("Value (Signaling)")) -> ()  [unwired: 2 in, 2 out]
                  }
                }
              }
            }
          }
          frame #8 {
            n349 = property on="Read Cal" class="Bool (strict)"("Val(Sgnl)"=TRUE ("Value (Signaling)")) -> ()  [unwired: 2 in, 2 out]
          }
          frame #9 {
            n350 = Wait (ms)(milliseconds to wait=u32 500) -> ()  [unwired: 1 out]
          }
          frame #10 {
            (unwired) FALSE ("Value (Signaling)")
          }
        }
        n351 = local write "Cal/Data Acq. Spot"(FALSE ("Cal/Data Acq. Spot")) -> ()
      }
      event "Take Stepping Data": Value Change {
        n352 = event-data() -> ()  [unwired: 1 in, 5 out]
        n353 = local read "Save ave N"() -> (w559:i32)
        n354 = flat-sequence {
          tunnel: w559 -> [w561]
          tunnel: [w561] -> w554
          tunnel: [w563] -> w555
          tunnel: w554 -> [w563]
          tunnel: [w565] -> w556
          tunnel: w555 -> [w565]
          tunnel: [w568] -> w557
          tunnel: w556 -> [w568]
          tunnel: [w570] -> w558
          tunnel: w557 -> [w570]
          tunnel: [w572] -> w552
          tunnel: w558 -> [w572]
          tunnel: w552 -> [w575]
          tunnel: [w575] -> w551
          tunnel: w551 -> [w576]
          tunnel: [w576] -> w553
          tunnel: w553 -> [w580]
          frame #0 {
            n355 = property on="Save ave N" class="DigNum (strict)"("Val(Sgnl)"="Save ave factor") -> ()  [unwired: 2 in, 2 out]
          }
          frame #1 {
            n356 = Wait (ms)(milliseconds to wait=u32 100) -> ()  [unwired: 1 out]
          }
          frame #2 {
            n357 = local read "Offset 2 Start (MHz)"() -> (w567:dbl)
            n358 = property on="Saved AOD Raster Scan Parameter Sets" class="Arr (strict)"("Index Values"=u32[] [2]) -> ()  [unwired: 2 in, 2 out]
            n359 = property on="Trap Delta (MHz)" class="Slide (strict)"("Val(Sgnl)"=w567) -> ()  [unwired: 2 in, 2 out]
          }
          frame #3 {
            n360 = property on="Load parameters" class="Bool (strict)"("Val(Sgnl)"=TRUE ("Value (Signaling)")) -> ()  [unwired: 2 in, 2 out]
          }
          frame #4 {
            n361 = Wait (ms)(milliseconds to wait=u32 100) -> ()  [unwired: 1 out]
          }
          frame #5 {
            n362 = property on="Trap Raster" class="Bool (strict)"("Val(Sgnl)"=TRUE ("Value (Signaling)")) -> ()  [unwired: 2 in, 2 out]
          }
          frame #6 {
            n363 = Wait (ms)(milliseconds to wait=u32 1000) -> ()  [unwired: 1 out]
          }
          frame #7 {
            n364 = while {
              stop <- w577 continue-if-true
              n365 = local read "Raster Scanning..."() -> (w579:bool)
              n366 = local read "Saving..."() -> (w578:bool)
              n367 = Or(x=w579, y=w578) -> (x .or. y?=w577:bool)
            }
          }
          frame #8 {
            n368 = property on="Save ave N" class="DigNum (strict)"("Val(Sgnl)"=w580) -> ()  [unwired: 2 in, 2 out]
          }
        }
      }
      event "Step Size (nm) 2": Value Change {
        n369 = event-data() -> ()  [unwired: 1 in, 5 out]
        n370 = flat-sequence {
          frame #0 {
            n371 = property on="Saved AOD Raster Scan Parameter Sets" class="Arr (strict)"("Index Values"=u32[] [1]) -> ()  [unwired: 2 in, 2 out]
          }
          frame #1 {
            n372 = Multiply(x="N Steps", y="Step Size (nm) 2") -> (x*y=w582:dbl)
            n373 = property on="Scan Speed AOD (nm/s) 2" class="DigNum (strict)"("Value"="Step Size (nm) 2") -> ()  [unwired: 2 in, 2 out]
            n374 = property on="Step Size AOD (nm) 2" class="DigNum (strict)"("Value"="Step Size (nm) 2") -> ()  [unwired: 2 in, 2 out]
            n375 = property on="Scan Range AOD (nm) 2" class="DigNum (strict)"("Value"=w582) -> ()  [unwired: 2 in, 2 out]
          }
        }
      }
      event "Take Green\nLaser Image": Value Change {
        n376 = event-data() -> ()  [unwired: 1 in, 5 out]
        n377 = flat-sequence {
          tunnel: [w610] -> w600
          tunnel: [w609] -> w593
          tunnel: [w608] -> w585
          tunnel: [w613] -> w601
          tunnel: w600 -> [w613]
          tunnel: [w612] -> w594
          tunnel: w593 -> [w612]
          tunnel: [w611] -> w586
          tunnel: w585 -> [w611]
          tunnel: [w617] -> w602
          tunnel: w601 -> [w617]
          tunnel: [w616] -> w595
          tunnel: w594 -> [w616]
          tunnel: [w615] -> w587
          tunnel: w586 -> [w615]
          tunnel: [w623] -> w603
          tunnel: w602 -> [w623]
          tunnel: [w622] -> w596
          tunnel: w595 -> [w622]
          tunnel: [w621] -> w588
          tunnel: w587 -> [w621]
          tunnel: [w627] -> w604
          tunnel: w603 -> [w627]
          tunnel: [w626] -> w597
          tunnel: w596 -> [w626]
          tunnel: [w625] -> w589
          tunnel: w588 -> [w625]
          tunnel: [w631] -> w605
          tunnel: w604 -> [w631]
          tunnel: [w630] -> w598
          tunnel: w597 -> [w630]
          tunnel: [w629] -> w590
          tunnel: w589 -> [w629]
          tunnel: [w635] -> w606
          tunnel: w605 -> [w635]
          tunnel: [w634] -> w599
          tunnel: w598 -> [w634]
          tunnel: [w633] -> w591
          tunnel: w590 -> [w633]
          tunnel: w606 -> [w641]
          tunnel: w599 -> [w640]
          tunnel: [w638] -> w592
          tunnel: w591 -> [w638]
          tunnel: w592 -> [w642]
          frame #0 {
            n378 = local read "Green laser mode"() -> (w609:enum32{"Laser ON", "Laser OFF", "Interlace"})
            n379 = local read "Green FB On/Off"() -> (w608:bool)
            n380 = local read "Green Laser"() -> (w610:bool)
          }
          frame #1 {
            n381 = property on="Green FB On/Off" class="Bool (strict)"("Val(Sgnl)"=FALSE ("Value (Signaling)")) -> ()  [unwired: 2 in, 2 out]
          }
          frame #2 {
            n382 = property on="Green Laser" class="Bool (strict)"("Val(Sgnl)"=TRUE ("Value (Signaling)")) -> ()  [unwired: 2 in, 2 out]
            n383 = property on="Flip Green Filter" class="Bool (strict)"("Val(Sgnl)"=TRUE ("Value (Signaling)")) -> ()  [unwired: 2 in, 2 out]
            n384 = property on="Green laser mode" class="RadioBtnsControl (strict)"("Val(Sgnl)"=enum32{"Laser ON", "Laser OFF", "Interlace"}."Laser ON" ("Value (Signaling)")) -> ()  [unwired: 2 in, 2 out]
          }
          frame #3 {
            n385 = Wait (ms)(milliseconds to wait=u32 500) -> ()  [unwired: 1 out]
          }
          frame #4 {
            n386 = property on="Confocal Image" class="Bool (strict)"("Val(Sgnl)"=TRUE ("Value (Signaling)")) -> ()  [unwired: 2 in, 2 out]
          }
          frame #5 {
            n387 = Wait (ms)(milliseconds to wait=u32 2000) -> ()  [unwired: 1 out]
          }
          frame #6 {
            n388 = while {
              stop <- w636 stop-if-true
              n389 = local read "Saving..."() -> (w637:bool)
              n390 = Not(x=w637) -> (.not. x?=w636:bool)
            }
          }
          frame #7 {
            n391 = property on="Flip Green Filter" class="Bool (strict)"("Val(Sgnl)"=TRUE ("Value (Signaling)")) -> ()  [unwired: 2 in, 2 out]
            n392 = property on="Green Laser" class="Bool (strict)"("Val(Sgnl)"=w641) -> ()  [unwired: 2 in, 2 out]
            n393 = property on="Green laser mode" class="RadioBtnsControl (strict)"("Val(Sgnl)"=w640) -> ()  [unwired: 2 in, 2 out]
          }
          frame #8 {
            n394 = property on="Green FB On/Off" class="Bool (strict)"("Val(Sgnl)"=w642) -> ()  [unwired: 2 in, 2 out]
          }
        }
      }
      event "Stop All": Value Change {
        n395 = event-data() -> ()  [unwired: 1 in, 5 out]
        n396 = local read "Stop All"() -> (w643:bool)
      }
    }
    n397 = node-c288() -> ()  [unwired: 1 in, 1 out]
  }
  n398 = timed-loop "Handle Events (Button Presses, etc.)" {
    tunnel: w46 -> [w647]
    shift-right: [w646] -> _
    shift-left: errorcluster {"status"=FALSE, "code"=0, "source"=""} ("error out") -> [w645]
    tunnel: [w644] -> w51
    timing: w39 -> [_]
    timing-out: [_] -> w38
    stop <- w644 stop-if-true
    n399 = event shown="[25] \"Invert APD Gate\", \"APD Gate ON Count\", \"APD Gate OFF Count\", \"APD Gate\", \"APD Integration Time (s)\", \"APD 1 AO Mult.\", \"APD 2 AO Mult.\": Value Change" {
      selector: _ -> [_ _ _ _ _ _ _ _ _ _ _ _ _ _ _ _ _ _ _ _ _ _ _ _ _ _ _ _ _ _ _ _ _ _ _ _ _ _ _ _ _ _ _ _ _ _ _ _ _ _ _ _ _ _ _ _ _]
      dyn-events: _ -> [_ _ _ _ _ _ _ _ _ _ _ _ _ _ _ _ _ _ _ _ _ _ _ _ _ _ _ _ _ _ _ _ _ _ _ _ _ _ _ _ _ _ _ _ _ _ _ _ _ _ _ _ _ _ _ _ _]
      timeout: _ -> [_ _ _ _ _ _ _ _ _ _ _ _ _ _ _ _ _ _ _ _ _ _ _ _ _ _ _ _ _ _ _ _ _ _ _ _ _ _ _ _ _ _ _ _ _ _ _ _ _ _ _ _ _ _ _ _ _]
      tunnel: w647 -> [w691 _ w711 _ w727 w751 _ _ w798 _ _ w842 w848 w852 w857 w893 w911 w918 _ w938 w949 w960 w971 w982 w993 w1011 w1017 w1097 _ w1109 w1147 _ w1214 w1219 w1223 w1234 w1239 w1263 _ w1275 _ _ _ _ _ w1380 w1395 w1410 w1436 w1439 w1443 _ w1460 w1463 _ _ _]
      tunnel: [w690 _ w701 _ _ w750 w763 _ w778 _ _ w841 w844 w851 w854 w892 w909 w917 _ w932 w943 w954 w965 w976 w987 w1009 w1016 w1095 _ w1107 w1145 _ _ w1217 w1221 w1224 w1237 w1261 _ w1273 _ _ _ _ _ w1378 _ _ _ _ _ _ _ _ _ _ _] -> w646
      tunnel: w645 -> [w689 _ w710 _ _ w749 w763 _ w797 _ _ w840 w843 w850 w853 w891 w910 w916 _ w937 w948 w959 w970 w981 w992 w1010 w1015 w1096 _ w1108 w1146 _ _ w1218 w1222 w1233 w1238 w1262 _ w1274 _ _ _ _ _ w1379 w1394 w1409 w1435 w1438 w1442 _ w1459 _ _ _ _]
      tunnel: [_ _ _ _ _ _ w762 _ _ _ _ _ _ _ _ _ _ _ _ _ _ _ _ _ _ _ _ _ _ _ _ _ _ _ _ _ _ _ _ _ _ _ _ _ _ _ _ _ _ _ _ _ _ _ _ _ _] -> w644
      tunnel: [_ _ _ _ _ _ _ _ _ _ _ _ _ _ _ _ _ _ _ _ _ _ _ _ _ _ _ _ _ _ _ _ _ _ _ _ _ _ _ _ _ _ _ _ _ _ _ _ _ _ "Set SP to Current Frc" _ _ _ _ _ _] -> _
      tunnel: [_ _ _ _ _ _ _ "Delayed Interlace Start" _ _ _ _ _ _ _ _ _ _ _ _ _ _ _ _ _ _ _ _ _ _ _ _ _ _ _ _ _ _ _ _ _ _ _ _ _ _ _ _ _ _ _ _ _ _ _ _ _] -> _
      event "AI Count (ticks)", "Sets to FIFO (Traps)", "Save ave N", "FPGA Ave.", "# Samples/channel", "N sets to save": Value Change {
        # "Make sure Save Ave N is a divisor of Samp/Trap , else default to 1"
        # "So that if 'Save ave N' is updated, the AOD scanning code updates too."
        n400 = event-data() -> ()  [unwired: 6 out]
        n401 = local read "AI Count (ticks)"() -> (w674:u32)
        n402 = Unbundle By Name("Sets to FIFO (Traps)") -> ("Set 1"=w659:bool, "Set 2"=w658:bool, "Set 3"=w657:bool)
        n403 = Boolean To (0,1)(Boolean="Sets to FIFO (Traps)") -> (0, 1=w683:cluster{"Set 1":i16, "Set 2":i16, "Set 3":i16})
        n404 = xnode "Read/Write Control"("FPGA VI Reference In"=w691, "error in"=w689, "ai count"=w674, "Set 1"=w659, "Set 2"=w658, "Set 3"=w657, "N of AI1 Int Acq Sets"="N Acq Sets (Traps + Fl.)") -> ("error out"=w690:errorcluster)  [unwired: 1 out]
        n405 = Cluster To Array(cluster=w683) -> (array=w682:i16[])
        n406 = local read "Scan steps (AOD)"() -> (w684:u64)
        n407 = To Unsigned Long Integer(number=w682) -> (unsigned 32bit integer=w664:u32[])
        n408 = Multiply(x=w674, y="N Acq Sets (Traps + Fl.)") -> (x*y=w672:u32)
        n409 = Divide(x=40000000.0, y=w674) -> (x/y=w667:dbl)
        "AI rate (Hz)" <- w667
        n410 = Add Array Elements(numeric array=w664) -> (sum=w675:u32)
        "Trap Sets" <- w675
        n411 = Reciprocal(x=w667) -> (1/x=→"Ave. Period (s)":dbl)
        n412 = property on="Scan steps (AOD)" class="DigNum (strict)"("Val(Sgnl)"=w684) -> ()  [unwired: 2 in, 2 out]
        n413 = local read "Save ave N"() -> (w653:i32)
        n414 = Divide(x=w667, y="N Acq Sets (Traps + Fl.)") -> (x/y=w686:dbl)
        "Data Rate (Hz)" <- w686
        n415 = Reciprocal(x=w686) -> (1/x=→"Data Period (s)":dbl)
        n416 = Quotient & Remainder(x="# Samples/trap", y=w653) -> (x-y*floor(x/y)=w655:u32)  [unwired: 1 out]
        n417 = Equal To 0?(x=w655) -> (x = 0?=w654:bool)
        n418 = Select(t=w653, s=w654, f=1) -> (s? t:f=w651:i32)
        n419 = local read "APD Integration Time (s)"() -> (w650:dbl)
        n420 = Divide(x=w686, y=w651) -> (x/y=→"Save Data Rate (Hz)":dbl)
        n421 = local write "Save ave N"(w651) -> ()
        n422 = Multiply(x=w650, y=40000000.0) -> (x*y=w648:dbl)
        n423 = Multiply(x=w672, y="# Samples/trap") -> (x*y=w671:u32)
        "Counts/DMA" <- w671
        n424 = property on="Trap Disp. Downsample" class="DigNum (strict)"("Maximum"="# Samples/trap") -> ()  [unwired: 2 in, 2 out]
        n425 = Multiply(x=w675, y="# Samples/trap") -> (x*y=w665:u32)
        "# Samples/channel" <- w665
        n426 = Multiply(x=w665, y=u32 8) -> (x*y=→"Trap FIFO El/Read":u32)
        n427 = Multiply(x=w665, y=u32 3) -> (x*y=→"TPos FIFO El/Read":u32)
        n428 = Divide(x=w671, y=w648) -> (x/y=w663:dbl)
        "APD Samples/FIFO Acq." <- w663
        n429 = Divide(x=w671, y=40000000.0) -> (x/y=w669:dbl)
        "DMA Update Period (s)" <- w669
        n430 = Multiply(x=2.0, y=w663) -> (x*y=→"APD FIFO El/Read":dbl)
        n431 = property on="APD Disp. dSamp" class="DigNum (strict)"("Maximum"=w663) -> ()  [unwired: 2 in, 2 out]
        n432 = local read "N sets to save"() -> (w680:u32)
        n433 = Multiply(x=w669, y=w680) -> (x*y=→"Total Time (s)":dbl)
        "FPGA Averaging" <- FALSE ("FPGA Averaging")
      }
      event "Detector Type": Value Change {
        n434 = event-data() -> ()  [unwired: 7 out]
        n435 = local read "AI labels"() -> (w692:string[])
        n436 = Build Array (concatenate)(w692, "none") -> (w693:string[])
        n437 = property on="FFT 1 Choice 1" class="Ring (strict)"("Strings []"=w693) -> ()  [unwired: 2 in, 2 out]
        n438 = property on="FFT 1 Choice 2" class="Ring (strict)"("Strings []"=w693) -> ()  [unwired: 2 in, 2 out]
        n439 = property on="FFT 2 Choice 1" class="Ring (strict)"("Strings []"=w693) -> ()  [unwired: 2 in, 2 out]
        n440 = property on="FFT 2 Choice 2" class="Ring (strict)"("Strings []"=w693) -> ()  [unwired: 2 in, 2 out]
        n441 = Bundle("APD 1", "APD 2") -> (w696:cluster{string, string})  [unwired: 1 out]
        n442 = Cluster To Array(cluster=w696) -> (array=w694:string[])
        n443 = Build Array (concatenate)(w694, w693) -> (w698:string[])
        n444 = Array Size(array=w698) -> (size(s)=w699:i32)
        n445 = property on="Signals to Plot" class="LstBox (strict)"("Item Names"=w698) -> ()  [unwired: 2 in, 2 out]
        n446 = property on="Signals to Plot" class="LstBox (strict)"("Number of Rows"=w699) -> ()  [unwired: 2 in, 2 out]
        n447 = property on="All Signals" class="WFChart (strict)"("LegNumRows"=w699) -> ()  [unwired: 2 in, 2 out]
      }
      event "Phase adj. (AI1)", "+ phase (AI1)", "- phase (AI1)": Value Change {
        n448 = event-data() -> ()  [unwired: 7 out]
        n449 = Negate(x="Phase adj. (AI1)") -> (-x=w708:i16)
        n450 = Select(t=w708, s="- phase (AI1)", f="Phase adj. (AI1)") -> (s? t:f=w707:i16)
        n451 = xnode "Read/Write Control"("FPGA VI Reference In"=w711, "error in"=w710, "Phase count adjustment"=w707) -> ("FPGA VI Reference Out"=w706:T18, "error out"=w705:errorcluster)
        n452 = Or(x="- phase (AI1)", y="+ phase (AI1)") -> (x .or. y?=w702:bool)
        n453 = xnode "Read/Write Control"("FPGA VI Reference In"=w706, "error in"=w705, "+ phase"=w702) -> ("error out"=w701:errorcluster)  [unwired: 1 out]
      }
      event "Signals to Plot": Double Click {
        w715 = u32 9868950 ("Color Box")
        n454 = event-data() -> ("Row"=w717:i32)  [unwired: 9 out]
        n455 = property on="All Signals" class="WFChart (strict)"("Active Plot"=w717) -> (error out=w725:errorcluster)  [unwired: 2 in, 1 out]
        n456 = property on="All Signals" class="WFChart (strict)"(error in=w725) -> (error out=w724:errorcluster, "Plot.Visible?"=w723:bool)  [unwired: 1 in, 1 out]
        n457 = Not(x=w723) -> (.not. x?=w712:bool)
        n458 = property on="All Signals" class="WFChart (strict)"(error in=w724, "Plot.Visible?"=w712) -> (error out=w722:errorcluster)  [unwired: 1 in, 1 out]
        n459 = property on="All Signals" class="WFChart (strict)"(error in=w722) -> (error out=w718:errorcluster, "Plot.Plot Color"=w721:u32)  [unwired: 1 in, 1 out]
        n460 = property on="Signals to Plot" class="LstBox (strict)"(error in=w718, "Active Row"=w717) -> (error out=w716:errorcluster)  [unwired: 1 in, 1 out]
        n461 = Select(t=w721, s=w712, f=u32 0) -> (s? t:f=w719:u32)
        n462 = property on="Signals to Plot" class="LstBox (strict)"(error in=w716, "CellFontColor"=w719, "SelColor"=w715, "CellBG"=w715, "CellFontSize"=u32 20 ("Active Row:Cell Font:Size"), "CellFontBold"=TRUE ("Active Row:Cell Font:Bold")) -> ()  [unwired: 1 in, 2 out]
      }
      event "Dynamic Force FB": Value Change {
        n463 = event-data() -> ()  [unwired: 7 out]
        n464 = xnode "Read/Write Control"("FPGA VI Reference In"=w727, "Dynamic Force FB (Ronen)"="Dynamic Force FB") -> ()  [unwired: 1 in, 2 out]
      }
      event "BD 1 Frq 1 (MHz)", "BD 1 Frq 2 (MHz)", "BD 1 Frq 3 (MHz)", "BD 2 Frq 1 (MHz)", "BD 2 Frq 2 (MHz)", "BD 2 Frq 3 (MHz)", "Trap Delta (MHz)": Value Change {
        # "anytime one of the frequencies is changed, write it to the RF board UNLESS Set 2 is being oscillated. The oscillation\nscript writes the frequencies to the RF board."
        n465 = event-data() -> ("CtlRef"=w748:refnum<vi>)  [unwired: 6 out]
        n466 = control-ref of="Trap Delta (MHz)"() -> (w747:refnum<vi>)
        n467 = Equal?(x=w747, y=w748) -> (x = y?=w746:bool)
        n468 = local read "Symmetric?"() -> (w728:bool)
        n469 = case shown="True" w728 {
          tunnel: ["Asym. T2 (MHz)" w760] -> w732
          tunnel: "Trap Delta (MHz)" -> [w754 w759]
          tunnel: [w753 w756] -> w729
          frame False {
            n470 = Subtract(x="Asym. T2 (MHz)", y=w754) -> (x-y=w753:dbl)
          }
          frame True {
            n471 = Divide(x=w759, y=2) -> (x/y=w757:dbl)
            n472 = Subtract(x="Sym. Mid (MHz)", y=w757) -> (x-y=w756:dbl)
            n473 = Add(x="Sym. Mid (MHz)", y=w757) -> (x+y=w760:dbl)
          }
        }
        n474 = local read "BD 1 Frq 2 (MHz)"() -> (w733:dbl)
        n475 = local write "BD 1 Frq 1 (MHz)"(w729) -> ()
        n476 = Select(t=w732, s=w746, f=w733) -> (s? t:f=w731:dbl)
        n477 = local read "Y RF Frequency Limits (MHz)"() -> (w734:T13)
        n478 = local read "X RF Freq Limits (MHz)"() -> (w735:T13)
        n479 = local read "BD 1 Frq 3 (MHz)"() -> (w744:dbl)
        n480 = local write "BD 1 Frq 2 (MHz)"(w731) -> ()
        n481 = local read "BD 2 Frq 1 (MHz)"() -> (w738:dbl)
        n482 = local read "BD 2 Frq 2 (MHz)"() -> (w737:dbl)
        n483 = local read "BD 2 Frq 3 (MHz)"() -> (w745:dbl)
        n484 = call "set RF board frequency - interlace.vi"("Board 2 Frequency Limits"=w734, "Board 1 Frequency Limits"=w735, "error in"=w749, "FPGA VI Reference In"=w751, "Board 2 Frequency 3 (MHz)"=w745, "Board 1 Frequency 3 (MHz)"=w744, "Board 2 Frequency 2 (MHz)"=w737, "Board 2 Frequency 1 (MHz)"=w738, "Board 1 Frequency 2 (MHz)"=w731, "Board 1 Frequency 1  (MHz)"=w729) -> ("error out"=w750:errorcluster)  [unwired: 1 out]
        n485 = Subtract(x=w738, y=w737) -> (x-y=w742:dbl)
        n486 = Subtract(x=w731, y=w729) -> (x-y=w743:dbl)
        n487 = Square(x=w742) -> (x^2=w740:dbl)
        n488 = Square(x=w743) -> (x^2=w741:dbl)
        n489 = Add(x=w741, y=w740) -> (x+y=w739:dbl)
        n490 = Square Root(x=w739) -> (sqrt(x)=w736:dbl)
        n491 = local write "Trap Delta (MHz)"(w736) -> ()
        n492 = property on="Initial delta (MHz)" class="DigNum (strict)"("Val(Sgnl)"=w736) -> ()  [unwired: 2 in, 2 out]
      }
      event "Stop All": Value Change {
        n493 = event-data() -> ()  [unwired: 7 out]
        n494 = call "hamilton_controller.vi"("action"=T19."DISCONNECT") -> ()  [unwired: 10 in, 1 out]
        n495 = local read "Stop All"() -> (w762:bool)
      }
      event "Delayed Interlace Start": Value Change {
        n496 = event-data() -> ()  [unwired: 7 out]
        n497 = flat-sequence {
          frame #0 {
            n498 = Multiply(x="Delay to Interlace (s)", y=1000.0) -> (x*y=w765:dbl)
            n499 = Wait (ms)(milliseconds to wait=w765) -> ()  [unwired: 1 out]
          }
          frame #1 {
            n500 = property on="Green laser mode" class="RadioBtnsControl (strict)"("Val(Sgnl)"=enum32{"Laser ON", "Laser OFF", "Interlace"}."Interlace" ("Value (Signaling)")) -> ()  [unwired: 2 in, 2 out]
          }
        }
      }
      event "BD 1 Amp 1 (%)", "BD 1 Amp 2 (%)", "BD 1 Amp 3 (%)", "BD 2 Amp 1 (%)", "BD 2 Amp 2 (%)", "BD 2 Amp 3 (%)", "Trap 1 ON", "Trap 2 ON", "Trap 3 ON", "Feedback On/Off", "All FB On/Off": Value Change {
        w789 = i16 1 ("f")
        n501 = event-data() -> ()  [unwired: 7 out]
        n502 = local write "Trap 1 (E)"("Trap 1 ON") -> ()
        n503 = local write "Trap 2 (R)"("Trap 2 ON") -> ()
        n504 = Boolean To (0,1)(Boolean="Trap 3 ON") -> (0, 1=w790:i16)
        n505 = Boolean To (0,1)(Boolean="Trap 1 ON") -> (0, 1=w791:i16)
        n506 = Boolean To (0,1)(Boolean="Trap 2 ON") -> (0, 1=w792:i16)
        n507 = Select(t=w792, s="Trap ON/OFF X or Y Amp?", f=w789) -> (s? t:f=w787:i16)
        n508 = Select(t=w791, s="Trap ON/OFF X or Y Amp?", f=w789) -> (s? t:f=w788:i16)
        n509 = Select(t=w790, s="Trap ON/OFF X or Y Amp?", f=w789) -> (s? t:f=w786:i16)
        n510 = Select(t=w789, s="Trap ON/OFF X or Y Amp?", f=w792) -> (s? t:f=w784:i16)
        n511 = Select(t=w789, s="Trap ON/OFF X or Y Amp?", f=w791) -> (s? t:f=w785:i16)
        n512 = Select(t=w789, s="Trap ON/OFF X or Y Amp?", f=w790) -> (s? t:f=w783:i16)
        n513 = And(x="All FB On/Off", y="Feedback On/Off") -> (x .and. y?=w781:cluster{"Set 1":bool, "Set 2":bool})
        n514 = Unbundle By Name(w781) -> ("Set 1"=w777:bool, "Set 2"=w774:bool)
        n515 = local read "BD 1 Amp 1 (%)"() -> (w801:dbl)
        n516 = local read "BD 1 Amp 2 (%)"() -> (w800:dbl)
        n517 = local read "BD 1 Amp 3 (%)"() -> (w799:dbl)
        n518 = local read "Y RF Amplitude Limits (%)"() -> (w770:T13)
        n519 = local read "X RF Amp Limits (%)"() -> (w771:T13)
        n520 = local read "BD 2 Amp 1 (%)"() -> (w802:dbl)
        n521 = local read "BD 2 Amp 2 (%)"() -> (w803:dbl)
        n522 = local read "BD 2 Amp 3 (%)"() -> (w804:dbl)
        n523 = And(x="Trap 2 ON", y=w774) -> (x .and. y?=w772:bool)
        n524 = And(x="Trap 1 ON", y=w777) -> (x .and. y?=w775:bool)
        n525 = Multiply(x=w788, y=w801) -> (x*y=w796:dbl)
        n526 = Multiply(x=w800, y=w787) -> (x*y=w794:dbl)
        n527 = Multiply(x=w799, y=w786) -> (x*y=w795:dbl)
        n528 = Multiply(x=w802, y=w785) -> (x*y=w805:dbl)
        n529 = Multiply(x=w803, y=w784) -> (x*y=w806:dbl)
        n530 = Multiply(x=w804, y=w783) -> (x*y=w807:dbl)
        n531 = call "set RF board amplitude - interlace.vi"("Board 2 Amplitude Limits"=w770, "Board 1 Amplitude Limits"=w771, "error in"=w797, "FPGA VI Reference In"=w798, "Board 2 Amplitude 3 (%)"=w807, "Board 1 Amplitude 3 (%)"=w795, "Board 2 Amplitude 2 (%)"=w806, "Board 2 Amplitude 1 (%)"=w805, "Board 1 Amplitude 2 (%)"=w794, "Board 1 Amplitude 1 (%)"=w796) -> ("error out"=w779:errorcluster, "FPGA VI Reference Out"=w780:T18)
        n532 = xnode "Read/Write Control"("FPGA VI Reference In"=w780, "error in"=w779, "FB On/Off Set 1"=w775, "FB On/Off Set 2"=w772) -> ("error out"=w778:errorcluster)  [unwired: 1 out]
        n533 = case shown="True" "All FB On/Off" {
          frame False {
          }
          frame True {
            n534 = local write "Feedback \noverload"(FALSE) -> ()
          }
        }
      }
      event "Load parameters": Value Change {
        n535 = event-data() -> ()  [unwired: 7 out]
        n536 = property on="Saved AOD Raster Scan Parameter Sets" class="Arr (strict)"() -> ("Index Values"=w819:u32[])  [unwired: 2 in, 2 out]
        n537 = Index Array(array=w819, index=0) -> (element=w816:u32)
        n538 = local write "Load parameters"(FALSE ("Load parameters")) -> ()
        n539 = Index Array(array="Saved AOD Raster Scan Parameter Sets", index=w816) -> (element=w815:T26)
        n540 = Unbundle By Name(w815) -> ("Scan Range AOD (nm) 2"=w814:dbl, "Step Size AOD (nm) 2"=w813:dbl, "Scan Speed AOD (nm/s) 2"=w812:dbl, "Number of scans (AOD) 2"=w811:u16)
        n541 = flat-sequence {
          tunnel: w814 -> [w822]
          tunnel: w813 -> [w821]
          tunnel: w812 -> [w820]
          tunnel: w811 -> [w823]
          frame #0 {
            n542 = local write "Scan Speed (nm/s)"(w820) -> ()
            n543 = local write "Scan Range (nm)"(w822) -> ()
            n544 = local write "Step Size (nm)"(w821) -> ()
          }
          frame #1 {
            n545 = property on="N F/B Scans (AOD)" class="DigNum (strict)"("Val(Sgnl)"=w823) -> ()  [unwired: 2 in, 2 out]
          }
        }
      }
      event "Trap 1 (E)", "Trap 2 (R)": Value Change {
        n546 = event-data() -> ()  [unwired: 7 out]
        n547 = property on="Trap 1 ON" class="Bool (strict)"("Val(Sgnl)"="Trap 1 (E)") -> ()  [unwired: 2 in, 2 out]
        n548 = property on="Trap 2 ON" class="Bool (strict)"("Val(Sgnl)"="Trap 2 (R)") -> ()  [unwired: 2 in, 2 out]
      }
      event "DIO count 1 (ticks)", "DIO count 2 (ticks)", "DIO count 3 (ticks)", "Interlace", "Number Interlace Sets", "Not-Interlacing Set": Value Change {
        n549 = event-data() -> ()  [unwired: 7 out]
        n550 = local read "DIO count 3 (ticks)"() -> (w836:u32)
        n551 = local read "DIO count 1 (ticks)"() -> (w838:u32)
        n552 = local read "DIO count 2 (ticks)"() -> (w837:u32)
        n553 = To Unsigned Byte Integer(number="Not-Interlacing Set") -> (unsigned 8bit integer=w827:u8)
        n554 = Add(x=w827, y=u8 1) -> (x+y=w831:u8)
        n555 = xnode "Read/Write Control"("FPGA VI Reference In"=w842, "error in"=w840, "DIO count 1 (ticks)"=w838, "DIO count 2 (ticks)"=w837, "DIO count 3 (ticks)"=w836, "Interlace ON/OFF"="Interlace", "Number Interlace Cycles"="Number Interlace Sets", "Interlace Off Parameters"=w831) -> ("error out"=w841:errorcluster)  [unwired: 1 out]
        n556 = Build Array(w838, w837, w836) -> (w829:u32[])
        n557 = Split 1D Array(array=w829, index="Number Interlace Sets") -> (first subarray=w839:u32[])  [unwired: 1 out]
        n558 = Index Array(array=w829, index=w827) -> (element=w828:u32)
        n559 = Add Array Elements(numeric array=w839) -> (sum=w833:u32)
        n560 = Select(t=w833, s="Interlace", f=w828) -> (s? t:f=→"Total Counts (ticks)":u32)
      }
      event "Reset Feedback": Value Change {
        n561 = event-data() -> ()  [unwired: 7 out]
        n562 = Unbundle By Name("Reset Feedback") -> ("Set 1"=w846:bool, "Set 2"=w845:bool)
        n563 = xnode "Read/Write Control"("FPGA VI Reference In"=w848, "error in"=w843, "FB Reset Set 1"=w846, "FB Reset Set 2"=w845) -> ("error out"=w844:errorcluster)  [unwired: 1 out]
      }
      event "PID gains": Value Change {
        n564 = event-data() -> ()  [unwired: 7 out]
        n565 = local read "PID gains"() -> (w849:T6)
        n566 = xnode "Read/Write Control"("FPGA VI Reference In"=w852, "error in"=w850, "FB Gains"=w849) -> ("error out"=w851:errorcluster)  [unwired: 1 out]
      }
      event "AI2 to Setpoint", "Trap Powers (V)": Value Change {
        n567 = event-data() -> ()  [unwired: 7 out]
        n568 = xnode "Read/Write Control"("FPGA VI Reference In"=w857, "error in"=w853) -> ("FPGA VI Reference Out"=w856:T18, "error out"=w855:errorcluster, "AI2 Y Sum Set 1"=w864:i16, "AI2 Y Sum Set 2"=w863:i16)
        n569 = Cluster To Array(cluster="AI2 to Setpoint") -> (array=w867:bool[])
        n570 = local read "AI2 (V)"() -> (w865:cluster{"Set 1":dbl, "Set 2":dbl})
        n571 = Or Array Elements(Boolean array=w867) -> (logical OR=w868:bool)
        n572 = Bundle By Name(cluster=w865, "Set 1"=w864, "Set 2"=w863) -> (w862:cluster{"Set 1":dbl, "Set 2":dbl})
        n573 = Divide(x=w862, y=3276.7) -> (x/y=w861:cluster{"Set 1":dbl, "Set 2":dbl})
        "AI2 (V)" <- w861
        n574 = case shown="False" w868 {
          tunnel: [w871 w888] -> w860
          tunnel: "AI2 to Setpoint" -> [_ w884]
          tunnel: "Trap Powers (V)" -> [w872 w887]
          tunnel: w861 -> [_ w881]
          frame False {
            n575 = Multiply(x=3276.7, y=w872) -> (x*y=w873:cluster{"Set 1":dbl, "Set 2":dbl})
            n576 = To Word Integer(number=w873) -> (16bit integer=w871:cluster{"Set 1":i16, "Set 2":i16})
          }
          frame True {
            n577 = Unbundle By Name(w881) -> ("Set 1"=w880:dbl, "Set 2"=w879:dbl)
            n578 = Unbundle By Name(w887) -> ("Set 1"=w886:dbl, "Set 2"=w885:dbl)
            n579 = Unbundle By Name(w884) -> ("Set 1"=w883:bool, "Set 2"=w882:bool)
            n580 = Select(t=w880, s=w883, f=w886) -> (s? t:f=w878:dbl)
            n581 = Select(t=w879, s=w882, f=w885) -> (s? t:f=w877:dbl)
            n582 = Bundle By Name(cluster=w887, "Set 1"=w878, "Set 2"=w877) -> (w875:cluster{"Set 1":dbl, "Set 2":dbl})
            n583 = local write "Trap Powers (V)"(w875) -> ()
            n584 = Multiply(x=3276.7, y=w875) -> (x*y=w876:cluster{"Set 1":dbl, "Set 2":dbl})
            n585 = To Word Integer(number=w876) -> (16bit integer=w888:cluster{"Set 1":i16, "Set 2":i16})
          }
        }
        n586 = Unbundle By Name(w860) -> ("Set 1"=w859:i16, "Set 2"=w858:i16)
        n587 = xnode "Read/Write Control"("FPGA VI Reference In"=w856, "error in"=w855, "FB Setpoint Set 1"=w859, "FB Setpoint Set 2"=w858) -> ("error out"=w854:errorcluster)  [unwired: 1 out]
      }
      event "Invert GI": Value Change {
        n588 = event-data() -> ()  [unwired: 7 out]
        n589 = xnode "Read/Write Control"("FPGA VI Reference In"=w893, "error in"=w891, "Invert GI"="Invert GI", "Invert GI 2"="Invert GI") -> ("error out"=w892:errorcluster)  [unwired: 1 out]
      }
      event "Green FB Setpoint (mV)", "Green FB Gains", "Green FB On/Off", "Current (%)", "Green int current ON count adj": Value Change {
        n590 = event-data() -> ()  [unwired: 7 out]
        n591 = local read "Green FB Setpoint (mV)"() -> (w900:dbl)
        n592 = local read "Current (%)"() -> (w903:dbl)
        n593 = Multiply(x=w900, y=3.2767) -> (x*y=w899:dbl)
        n594 = Multiply(x=w903, y=655.35) -> (x*y=w904:dbl)
        n595 = To Unsigned Word Integer(number=w904) -> (unsigned 16bit integer=w902:u16)
        n596 = local read "Green int current ON count adj"() -> (w907:u32)
        n597 = local read "Green FB Gains"() -> (w906:T6)
        n598 = local read "Green laser mode"() -> (w896:enum32{"Laser ON", "Laser OFF", "Interlace"})
        n599 = local read "Green Laser"() -> (w897:bool)
        n600 = local read "Green FB On/Off"() -> (w908:bool)
        n601 = Equal?(x=w896, y=enum32{"Laser ON", "Laser OFF", "Interlace"}."Interlace") -> (x = y?=w894:bool)
        n602 = Compound Arithmetic op=AND(w894, w908, w897) -> (w898:bool)
        n603 = xnode "Read/Write Control"("FPGA VI Reference In"=w911, "error in"=w910, "Green FB Setpoint"=w899, "Green FB On/Off"=w898, "Current Out"=w902, "Green int current ON count adj"=w907, "Green FB Gains"=w906) -> ("error out"=w909:errorcluster)  [unwired: 1 out]
      }
      event "Green laser mode", "Green Laser": Value Change {
        n604 = event-data() -> ()  [unwired: 7 out]
        n605 = case shown="True" "Green Laser" {
          tunnel: "Green laser mode" -> [_ w925]
          tunnel: [enum32{"Laser ON", "Laser OFF", "Interlace"}."Laser OFF" ("Green laser mode") w925] -> w913
          tunnel: [FALSE w921] -> w912
          frame False {
          }
          frame True {
            n606 = local read "Green FB On/Off"() -> (w922:bool)
            n607 = Equal?(x=w925, y=enum32{"Laser ON", "Laser OFF", "Interlace"}."Interlace") -> (x = y?=w923:bool)
            n608 = And(x=w923, y=w922) -> (x .and. y?=w921:bool)
          }
        }
        n609 = xnode "Read/Write Control"("FPGA VI Reference In"=w918, "error in"=w916, "Operating Mode"=w913, "Operating Mode 2"=w913, "Green FB On/Off"=w912) -> ("error out"=w917:errorcluster)  [unwired: 1 out]
      }
      event "Feedback \noverload": Value Change {
        # "Click the FB Overload button to turn on FB"
        n610 = event-data() -> ()  [unwired: 7 out]
        n611 = local write "Feedback \noverload"(FALSE ("Value (Signaling)")) -> ()
        n612 = property on="All FB On/Off" class="Bool (strict)"("Val(Sgnl)"=TRUE ("Value (Signaling)")) -> ()  [unwired: 2 in, 2 out]
      }
      event "- phase (APD 1 Gate)", "+ phase (APD 1 Gate)": Value Change {
        n613 = event-data() -> ()  [unwired: 7 out]
        n614 = local read "Phase Adj. (APD 1 Gate)"() -> (w928:i16)
        n615 = Negate(x=w928) -> (-x=w936:i16)
        n616 = Select(t=w936, s="- phase (APD 1 Gate)", f=w928) -> (s? t:f=w935:i16)
        n617 = Or(x="- phase (APD 1 Gate)", y="+ phase (APD 1 Gate)") -> (x .or. y?=w931:bool)
        n618 = xnode "Read/Write Control"("FPGA VI Reference In"=w938, "error in"=w937, "Phase count adjustment (APD 1 Gate)"=w935) -> ("FPGA VI Reference Out"=w933:T18, "error out"=w934:errorcluster)
        n619 = xnode "Read/Write Control"("FPGA VI Reference In"=w933, "error in"=w934, "+ phase (APD 1 Gate)"=w931) -> ("error out"=w932:errorcluster)  [unwired: 1 out]
      }
      event "+ phase (APD 2 Gate)", "- phase (APD 2 Gate)": Value Change {
        n620 = event-data() -> ()  [unwired: 7 out]
        n621 = local read "Phase Adj. (APD 2 Gate)"() -> (w939:i16)
        n622 = Negate(x=w939) -> (-x=w947:i16)
        n623 = Select(t=w947, s="- phase (APD 2 Gate)", f=w939) -> (s? t:f=w946:i16)
        n624 = Or(x="- phase (APD 2 Gate)", y="+ phase (APD 2 Gate)") -> (x .or. y?=w942:bool)
        n625 = xnode "Read/Write Control"("FPGA VI Reference In"=w949, "error in"=w948, "Phase count adjustment (APD 2 Gate)"=w946) -> ("FPGA VI Reference Out"=w944:T18, "error out"=w945:errorcluster)
        n626 = xnode "Read/Write Control"("FPGA VI Reference In"=w944, "error in"=w945, "+ phase (APD 2 Gate)"=w942) -> ("error out"=w943:errorcluster)  [unwired: 1 out]
      }
      event "Phase Adj. (APD Acq)", "+ phase (APD Acq)", "- phase (APD Acq)": Value Change {
        n627 = event-data() -> ()  [unwired: 7 out]
        n628 = local read "Phase Adj. (APD Acq)"() -> (w952:i16)
        n629 = Negate(x=w952) -> (-x=w958:i16)
        n630 = Select(t=w958, s="+ phase (APD Acq)", f=w952) -> (s? t:f=w957:i16)
        n631 = Or(x="+ phase (APD Acq)", y="- phase (APD Acq)") -> (x .or. y?=w953:bool)
        n632 = xnode "Read/Write Control"("FPGA VI Reference In"=w960, "error in"=w959, "Phase Count Adjustment (APD Acq)"=w957) -> ("FPGA VI Reference Out"=w955:T18, "error out"=w956:errorcluster)
        n633 = xnode "Read/Write Control"("FPGA VI Reference In"=w955, "error in"=w956, "+ phase (APD Acq)"=w953) -> ("error out"=w954:errorcluster)  [unwired: 1 out]
      }
      event "Phase adj. (GI)", "+ phase (GI)", "- phase (GI)": Value Change {
        n634 = event-data() -> ()  [unwired: 7 out]
        n635 = Negate(x="Phase adj. (GI)") -> (-x=w969:i16)
        n636 = Select(t=w969, s="+ phase (GI)", f="Phase adj. (GI)") -> (s? t:f=w968:i16)
        n637 = Or(x="+ phase (GI)", y="- phase (GI)") -> (x .or. y?=w964:bool)
        n638 = xnode "Read/Write Control"("FPGA VI Reference In"=w971, "error in"=w970, "Phase count adjustment (GI)"=w968) -> ("FPGA VI Reference Out"=w966:T18, "error out"=w967:errorcluster)
        n639 = xnode "Read/Write Control"("FPGA VI Reference In"=w966, "error in"=w967, "+ phase (GI)"=w964) -> ("error out"=w965:errorcluster)  [unwired: 1 out]
      }
      event "Phase adj. (GI) 2", "+ phase (GI) 2", "- phase (GI) 2": Value Change {
        n640 = event-data() -> ()  [unwired: 7 out]
        n641 = Negate(x="Phase adj. (GI) 2") -> (-x=w980:i16)
        n642 = Select(t=w980, s="+ phase (GI) 2", f="Phase adj. (GI) 2") -> (s? t:f=w979:i16)
        n643 = Or(x="+ phase (GI) 2", y="- phase (GI) 2") -> (x .or. y?=w975:bool)
        n644 = xnode "Read/Write Control"("FPGA VI Reference In"=w982, "error in"=w981, "Phase count adjustment (GI) 2"=w979) -> ("FPGA VI Reference Out"=w977:T18, "error out"=w978:errorcluster)
        n645 = xnode "Read/Write Control"("FPGA VI Reference In"=w977, "error in"=w978, "+ phase (GI) 2"=w975) -> ("error out"=w976:errorcluster)  [unwired: 1 out]
      }
      event "Phase adj. (Green FB)", "- phase (Green FB)", "+ phase (Green FB)": Value Change {
        n646 = event-data() -> ()  [unwired: 7 out]
        n647 = Negate(x="Phase adj. (Green FB)") -> (-x=w991:i16)
        n648 = Select(t=w991, s="+ phase (Green FB)", f="Phase adj. (Green FB)") -> (s? t:f=w990:i16)
        n649 = Or(x="+ phase (Green FB)", y="- phase (Green FB)") -> (x .or. y?=w986:bool)
        n650 = xnode "Read/Write Control"("FPGA VI Reference In"=w993, "error in"=w992, "Phase count adjustment (Green FB)"=w990) -> ("FPGA VI Reference Out"=w988:T18, "error out"=w989:errorcluster)
        n651 = xnode "Read/Write Control"("FPGA VI Reference In"=w988, "error in"=w989, "+ phase (Green FB)"=w986) -> ("error out"=w987:errorcluster)  [unwired: 1 out]
      }
      event "Invert APD Gate", "APD Gate ON Count", "APD Gate OFF Count", "APD Gate", "APD Integration Time (s)", "APD 1 AO Mult.", "APD 2 AO Mult.": Value Change {
        n652 = event-data() -> ()  [unwired: 7 out]
        n653 = local read "APD Integration Time (s)"() -> (w995:dbl)
        n654 = local read "APD Gate ON Count"() -> (w1007:u32)
        n655 = local read "APD Gate OFF Count"() -> (w1006:u32)
        n656 = local read "Invert APD Gate"() -> (w1008:bool)
        n657 = local read "APD Gate"() -> (w1005:enum32{"ON", "OFF", "Interlace"})
        n658 = local write "Reset"(TRUE ("Reset")) -> ()
        n659 = Multiply(x=w995, y=40000000.0) -> (x*y=w1003:dbl)
        n660 = To Unsigned Long Integer(number=w1003) -> (unsigned 32bit integer=w1002:u32)
        n661 = local read "DMA Update Period (s)"() -> (w996:dbl)
        n662 = Divide(x=w996, y=w995) -> (x/y=w999:dbl)
        n663 = local read "APD 1 AO Mult."() -> (w1001:i16)
        n664 = local read "APD 2 AO Mult."() -> (w1000:i16)
        n665 = Multiply(x=2.0, y=w999) -> (x*y=w998:dbl)
        n666 = local write "APD Samples/FIFO Acq."(w999) -> ()
        n667 = local write "APD FIFO El/Read"(w998) -> ()
        n668 = xnode "Read/Write Control"("FPGA VI Reference In"=w1011, "error in"=w1010, "Invert APD Gate"=w1008, "APD Gate ON Count"=w1007, "APD Gate OFF Count"=w1006, "APD Acq Rate Count"=w1002, "APD Gate Operating Mode"=w1005, "APD 1 AO scale factor"=w1001, "APD 2 AO scale factor"=w1000) -> ("error out"=w1009:errorcluster)  [unwired: 1 out]
      }
      event "GI Frequency, ON count", "Green FB Count", "GI Frequency, OFF count": Value Change {
        n669 = event-data() -> ()  [unwired: 7 out]
        n670 = xnode "Read/Write Control"("FPGA VI Reference In"=w1017, "error in"=w1015, "Green interlace ON count"="GI Frequency, ON count", "Green interlace OFF count"="GI Frequency, OFF count", "Green interlace ON count 2"="GI Frequency, ON count", "Green interlace OFF count 2"="GI Frequency, OFF count", "Green FB Count"="Green FB Count") -> ("error out"=w1016:errorcluster)  [unwired: 1 out]
      }
      event "N F/B Scans (AOD)", "Scan Speed (nm/s)", "Scan BD", "Initial delta (MHz)", "Step Size (nm)", "Scan Range (nm)": Value Change {
        n671 = event-data() -> ()  [unwired: 7 out]
        n672 = local read "AOM X Cal (nm/MHz)"() -> (w1054:dbl)
        n673 = local read "Y RF Frequency Limits (MHz)"() -> (w1062:T13)
        n674 = local read "X RF Freq Limits (MHz)"() -> (w1065:T13)
        n675 = local read "BD 1 Frq 1 (MHz)"() -> (w1061:dbl)
        n676 = local read "BD 2 Frq 1 (MHz)"() -> (w1067:dbl)
        n677 = Negate(x="Scan Range (nm)") -> (-x=w1032:dbl)
        n678 = Divide(x=w1032, y=w1054) -> (x/y=w1036:dbl)
        n679 = Select(t=w1065, s="Scan BD", f=w1062) -> (s? t:f=w1064:T13)
        n680 = Select(t=w1061, s="Scan BD", f=w1067) -> (s? t:f=w1066:dbl)
        n681 = Unbundle By Name(w1064) -> ("Maximum"=w1073:dbl, "Minimum"=w1072:dbl)
        n682 = Add(x=w1036, y=w1066) -> (x+y=w1070:dbl)
        n683 = Divide(x=w1032, y="Step Size (nm)") -> (x/y=w1051:dbl)
        n684 = Divide(x="Step Size (nm)", y=w1054) -> (x/y=w1059:dbl)
        n685 = Absolute Value(x=w1051) -> (abs(x)=w1035:dbl)
        n686 = Sign(1:w1032) -> (0:w1033:dbl)
        n687 = In Range and Coerce(upper limit=w1073, x=w1070, lower limit=w1072) -> (coerced(x)=w1069:dbl, In Range?=w1071:bool)
        n688 = To Unsigned Quad Integer(1:w1035) -> (0:w1050:u64)
        "Scan steps (AOD)" <- w1050
        n689 = call "IR AOM freq to word.vi"("Frequency In (MHz)"=w1059) -> ("Frequency Word Out (double)"=w1057:dbl)
        n690 = Multiply(x=w1033, y=w1057) -> (x*y=w1034:dbl)
        n691 = Subtract(x=w1070, y=w1069) -> (x-y=w1068:dbl)
        n692 = To Quad Integer(1:w1034) -> (0:w1056:i64)
        n693 = Subtract(x=w1036, y=w1068) -> (x-y=w1055:dbl)
        "Scan Range (MHz)" <- w1055
        n694 = Select(t=w1036, s=w1071, f=w1055) -> (s? t:f=w1074:dbl)
        n695 = Multiply(x=w1055, y=w1054) -> (x*y=w1053:dbl)
        n696 = Decrement(x=w1050) -> (x-1=w1089:u64)
        n697 = Negate(x=w1053) -> (-x=w1049:dbl)
        n698 = local write "Scan Range (nm)"(w1049) -> ()
        n699 = Divide(x=w1074, y=w1089) -> (x/y=→"Scan Step (MHz)":dbl)
        n700 = Divide(x="Step Size (nm)", y="Scan Speed (nm/s)") -> (x/y=w1046:dbl)
        n701 = local read "Number Interlace Sets"() -> (w1030:u8)
        n702 = local read "AI Count (ticks)"() -> (w1031:u32)
        n703 = local read "Total Counts (ticks)"() -> (w1029:u32)
        n704 = local read "# Samples/trap"() -> (w1060:u32)
        n705 = Multiply(x=w1031, y=w1030) -> (x*y=w1028:u32)
        n706 = Divide(x=w1029, y=w1028) -> (x/y=w1027:dbl)
        n707 = Divide(x=w1029, y=40000000.0) -> (x/y=w1045:dbl)
        n708 = Divide(x=w1046, y=w1045) -> (x/y=w1044:dbl)
        n709 = To Unsigned Quad Integer(1:w1044) -> (0:w1019:u64)
        n710 = Quotient & Remainder(x=w1019, y=u64 2) -> (x-y*floor(x/y)=w1023:u64)  [unwired: 1 out]
        n711 = Equal?(x=w1023, y=u64 0) -> (x = y?=w1021:bool)
        n712 = Decrement(x=w1019) -> (x-1=w1020:u64)
        n713 = Select(t=w1019, s=w1021, f=w1020) -> (s? t:f=w1018:u64)
        "Cycles/step (AOD)" <- w1018
        n714 = xnode "Read/Write Control"("FPGA VI Reference In"=w1097, "error in"=w1096, "Scan steps"=w1050, "Number of scans"="N F/B Scans (AOD)", "Cycles per step"=w1018, "Scan freq.  increment"=w1056, "Scan BD"="Scan BD") -> ("error out"=w1095:errorcluster)  [unwired: 1 out]
        n715 = Multiply(x=w1050, y=w1018) -> (x*y=w1090:u64)
        n716 = Multiply(x=w1090, y=u64 2) -> (x*y=w1026:u64)
        n717 = Multiply(x=w1027, y=w1026) -> (x*y=w1025:dbl)
        n718 = Multiply(x=w1025, y="N F/B Scans (AOD)") -> (x*y=w1093:dbl)
        n719 = Divide(x=w1093, y=w1060) -> (x/y=→"Trap Raster N Sets":dbl)
        n720 = Multiply(x=w1090, y=w1045) -> (x*y=w1043:dbl)
        "Time/Scan (s) (AOD)" <- w1043
        n721 = Select(t=w1074, s="Scan BD", f=0.0) -> (s? t:f=w1088:dbl)
        n722 = Select(t=0.0, s="Scan BD", f=w1074) -> (s? t:f=w1085:dbl)
        n723 = local read "BD 2 Frq 2 (MHz)"() -> (w1081:dbl)
        n724 = local read "BD 1 Frq 2 (MHz)"() -> (w1084:dbl)
        n725 = Add(x=w1085, y=w1067) -> (x+y=w1082:dbl)
        n726 = Add(x=w1061, y=w1088) -> (x+y=w1083:dbl)
        n727 = Multiply(x=w1043, y=2.0) -> (x*y=w1042:dbl)
        n728 = Multiply(x=w1042, y="N F/B Scans (AOD)") -> (x*y=w1039:dbl)
        n729 = Divide(x=w1039, y=60.0) -> (x/y=→"Time to Finish All (min)":dbl)
        n730 = Subtract(x=w1082, y=w1081) -> (x-y=w1079:dbl)
        n731 = Subtract(x=w1083, y=w1084) -> (x-y=w1080:dbl)
        n732 = Square(x=w1079) -> (x^2=w1078:dbl)
        n733 = Square(x=w1080) -> (x^2=w1077:dbl)
        n734 = Add(x=w1077, y=w1078) -> (x+y=w1076:dbl)
        n735 = Square Root(x=w1076) -> (sqrt(x)=→"Final delta (MHz)":dbl)
      }
      event "Raster Scanning...": Value Change {
        n736 = event-data() -> ("NewVal"=w1098:bool)  [unwired: 6 out]
        n737 = case shown="True" w1098 {
          frame False {
          }
          frame True {
            n738 = property on="BD 1 Frq 1 (MHz)" class="DigNum (strict)"("Val(Sgnl)"=65.0 ("Value (Signaling)")) -> ()  [unwired: 2 in, 2 out]
          }
        }
      }
      event "Phase increment trap 1", "Swap F1 and F2", "Freq switch delay", "Amp switch delay", "Phase increment trap 2", "RF phase reset before cycles", "Phase offset method": Value Change {
        n739 = event-data() -> ()  [unwired: 7 out]
        n740 = local read "Amp switch delay"() -> (w1104:u16)
        n741 = local read "Phase increment trap 1"() -> (w1103:fxp<+/-,64,32>)
        n742 = local read "Freq switch delay"() -> (w1106:u16)
        n743 = local read "Phase increment trap 2"() -> (w1102:fxp<+/-,64,32>)
        n744 = local read "RF phase reset before cycles"() -> (w1101:bool)
        n745 = local read "Swap F1 and F2"() -> (w1105:bool)
        n746 = local read "Phase offset method"() -> (w1100:u8)
        n747 = xnode "Read/Write Control"("FPGA VI Reference In"=w1109, "error in"=w1108, "BD 1 Delay (ticks)"=w1106, "Swap F1 and F2"=w1105, "Amp switch delay"=w1104, "Phase Trap 1"=w1103, "Phase Trap 2"=w1102, "RF phase reset before cycles"=w1101, "Phase offset method"=w1100) -> ("error out"=w1107:errorcluster)  [unwired: 1 out]
      }
      event "Scan steps (x)", "Number of scans (MCL)", "Scan Range (V)", "2D or 1D Scan", "N APD Samp/step", "Fast Scan Dir", "Continuous MCL Scanning", "Scan lines (y)": Value Change {
        w1111 = 32767.0 ("y")
        n748 = event-data() -> ()  [unwired: 7 out]
        n749 = Select(t="Scan lines (y)", s="2D or 1D Scan", f="Number of scans (MCL)") -> (s? t:f=w1116:u64)
        n750 = Decrement(x="Scan steps (x)") -> (x-1=w1132:u64)
        n751 = Divide(x="Scan Range (V)", y=w1132) -> (x/y=w1131:dbl)
        "Desired Scan Incr (V)" <- w1131
        n752 = local read "APD Integration Time (s)"() -> (w1124:dbl)
        n753 = Multiply(x=w1131, y=w1111) -> (x*y=w1140:dbl)
        n754 = Divide(x=w1140, y=10.0) -> (x/y=w1130:dbl)
        "Desired incr (int)" <- w1130
        n755 = local read "Update Count (MCL)"() -> (w1136:u32)
        n756 = Round Toward -Infinity(1:w1130) -> (0:w1139:dbl)
        n757 = To Word Integer(number=w1139) -> (16bit integer=w1114:i16)
        n758 = Multiply(x=w1124, y=40000000.0) -> (x*y=w1137:dbl)
        n759 = Divide(x=w1137, y=w1136) -> (x/y=w1135:dbl)
        n760 = Multiply(x=i16 10, y=w1114) -> (x*y=w1112:i16)
        n761 = Multiply(x="N APD Samp/step", y=w1135) -> (x*y=w1134:dbl)
        "Cycles/step (MCL)" <- w1134
        n762 = Divide(x=w1112, y=w1111) -> (x/y=→"Actual MCL Inc (V)":dbl)
        n763 = Multiply(x="N APD Samp/step", y="Scan steps (x)") -> (x*y=w1126:u64)
        n764 = local read "APD Samples/FIFO Acq."() -> (w1123:dbl)
        n765 = Multiply(x=w1126, y=u64 2) -> (x*y=w1125:u64)
        n766 = Multiply(x=w1125, y=w1116) -> (x*y=w1143:u64)
        "Data points/scans (MCL)" <- w1143
        n767 = Multiply(x=w1124, y=w1125) -> (x*y=w1117:dbl)
        n768 = Divide(x=w1143, y=w1123) -> (x/y=→"MCL Scan N Sets":dbl)
        n769 = Multiply(x=w1117, y=w1116) -> (x*y=→"MCL Scan Time (s)":dbl)
        n770 = Not(x="Fast Scan Dir") -> (.not. x?=w1121:bool)
        n771 = xnode "Read/Write Control"("FPGA VI Reference In"=w1147, "error in"=w1146, "Scan steps (MCL)"="Scan steps (x)", "Number of scans (MCL)"=w1116, "Cycles per step (MCL)"=w1134, "Scan freq.  increment (MCL)"=w1114, "1D or 2D Scan?"="2D or 1D Scan", "MCL Scan Axis"=w1121, "Cont. Scan (MCL)"="Continuous MCL Scanning") -> ("error out"=w1145:errorcluster)  [unwired: 1 out]
      }
      event "Read Cal": Value Change {
        w1174 = T25."big-endian, network order" ("byte order (0:big-endian, network order)")
        w1175 = -1 ("count (1)")
        n772 = event-data() -> ()  [unwired: 7 out]
        n773 = local read "Save file name"() -> (w1199:path)
        n774 = local write "Read Cal"(FALSE ("Read Cal")) -> ()
        n775 = Strip Path(path=w1199) -> (stripped path=w1198:path)  [unwired: 1 out]
        n776 = Path To String(path=w1198) -> (string=w1184:string)
        n777 = Concatenate Strings(w1184, "\\current.off" ("string")) -> (w1182:string)
        n778 = Concatenate Strings(w1184, "\\current.cal" ("string")) -> (w1196:string)
        n779 = local read "Scale intensities (Q)"() -> (w1154:bool)
        n780 = String To Path(string=w1196) -> (path=w1195:path)
        n781 = String To Path(string=w1182) -> (path=w1181:path)
        n782 = Open/Create/Replace File(file path (use dialog)=w1195, operation (0:open)=T24."open", access (0:read/write)=enum16{"read/write", "read-only", "write-only"}."read-only") -> (refnum out=w1202:refnum<file>, error out=w1191:errorcluster)  [unwired: 1 in, 3 out]
        n783 = Deny Access(4:w1191, 7:w1202) -> (0:w1190:errorcluster, 3:w1194:refnum<file>)  [unwired: 1 out]
        n784 = Open/Create/Replace File(file path (use dialog)=w1181, operation (0:open)=T24."open", access (0:read/write)=enum16{"read/write", "read-only", "write-only"}."read-only") -> (refnum out=w1178:refnum<file>)  [unwired: 1 in, 4 out]
        n785 = Deny Access(7:w1178) -> (3:w1176:refnum<file>)  [unwired: 1 in, 2 out]
        n786 = Read from Binary File(5:0.0, 8:w1190, 9:w1174, 10:w1175, 11:w1194) -> (0:w1189:errorcluster, 2:w1187:dbl[], 3:w1192:refnum<file>)  [unwired: 2 out]
        n787 = Array To Cluster(array=w1187) -> (cluster=w1186:T27)
        n788 = Unbundle(w1186) -> ("[0]"=w1165:dbl, "[1]"=w1164:dbl, "[2]"=w1151:dbl, "[3]"=w1153:dbl, "[4]"=w1149:dbl, "[5]"=w1148:dbl)
        n789 = case "Cal is OK if you load a cal with scale intensities on - Alex 081418" shown="True" w1154 {
          tunnel: w1153 -> [w1204 w1207]
          tunnel: [w1204 w1206] -> w1152
          tunnel: w1151 -> [w1203 w1209]
          tunnel: [w1203 w1208] -> w1150
          frame False {
          }
          frame True {
            n790 = local read "Scale factor"() -> (w1205:dbl)
            n791 = Multiply(x=w1207, y=w1205) -> (x*y=w1206:dbl)
            n792 = Multiply(x=w1209, y=w1205) -> (x*y=w1208:dbl)
          }
        }
        n793 = Close File(refnum=w1192, error in=w1189) -> (error out=→"Read cal error":errorcluster)  [unwired: 1 out]
        n794 = local write "T2 kaX (pN/nm)"(w1152) -> ()
        n795 = local write "T1 kaX (pN/nm)"(w1150) -> ()
        n796 = local write "T1 alX (nm/V)"(w1165) -> ()
        n797 = local write "T2 alX (nm/V)"(w1164) -> ()
        n798 = Read from Binary File(5:0.0, 9:w1174, 10:w1175, 11:w1176) -> (2:w1170:dbl[], 3:w1173:refnum<file>)  [unwired: 1 in, 3 out]
        n799 = local write "T1 offX (V)"(w1149) -> ()
        n800 = local write "T2 offX (V)"(w1148) -> ()
        n801 = Close File(refnum=w1173) -> ()  [unwired: 1 in, 2 out]
        n802 = Array Subset(array=w1170, index=3) -> (w1168:dbl[])  [unwired: 1 in]
        n803 = Index Array(array=w1170, index=0) -> (element=→"Offset file step size":dbl)
        n804 = Multiply(x=w1165, y=w1151) -> (x*y=w1162:dbl)
        n805 = Multiply(x=w1164, y=w1153) -> (x*y=w1163:dbl)
        n806 = Divide(x=w1163, y=w1162) -> (x/y=w1156:dbl)
        n807 = Decimate 1D Array(w1168) -> (w1160:dbl[], w1161:dbl[])  [unwired: 1 out]
        n808 = disable-structure "Removed B factor to improve position FB -Alex 081418 2of3" shown="Enabled" {
          disable-tunnel: w1156 -> [w1210 _]
          disable-tunnel: [w1210 1.0] -> w1155
          frame Disabled {
          }
          frame Enabled {
          }
        }
        n809 = Bundle By Name(cluster="Offset Values", "Trap 1X offset"=w1160, "Trap 2X offset"=w1161) -> (w1166:T14)
        n810 = Multiply(x=w1161, y=w1155) -> (x*y=w1159:dbl[])
        n811 = Subtract(x=w1160, y=w1159) -> (x-y=w1158:dbl[])
        n812 = local write "Offset Values"(w1166) -> ()
        n813 = case shown="True" "Auto read offset\ncorrection" {
          tunnel: w1158 -> [_ w1212]
          frame False {
          }
          frame True {
            n814 = property on="Setpoint offset\nCorrection values" class="Arr (strict)"("Val(Sgnl)"=w1212) -> ()  [unwired: 2 in, 2 out]
          }
        }
        n815 = property on="B factor" class="DigNum (strict)"("Val(Sgnl)"=w1155) -> ()  [unwired: 2 in, 2 out]
      }
      event "Symmetric?": Value Change {
        n816 = event-data() -> ()  [unwired: 7 out]
        n817 = xnode "Read/Write Control"("FPGA VI Reference In"=w1214, "Symmetric FB/Raster"="Symmetric?") -> ()  [unwired: 1 in, 2 out]
      }
      event "Abort MCL Scan": Value Change {
        n818 = event-data() -> ()  [unwired: 7 out]
        n819 = local write "MCL Scanning"(FALSE ("MCL Scanning")) -> ()
        n820 = xnode "Read/Write Control"("FPGA VI Reference In"=w1219, "error in"=w1218, "Abort scan (MCL)"="Abort MCL Scan") -> ("error out"=w1217:errorcluster)  [unwired: 1 out]
      }
      event "Update Count (MCL)": Value Change {
        n821 = event-data() -> ()  [unwired: 7 out]
        n822 = xnode "Read/Write Control"("FPGA VI Reference In"=w1223, "error in"=w1222, "MCL count"="Update Count (MCL)") -> ("error out"=w1221:errorcluster)  [unwired: 1 out]
      }
      event "Phase adjust (MCL)", "+ phase (MCL)", "- phase (MCL)": Value Change {
        n823 = event-data() -> ()  [unwired: 7 out]
        n824 = Negate(x="Phase adjust (MCL)") -> (-x=w1232:i16)
        n825 = Select(t=w1232, s="- phase (MCL)", f="Phase adjust (MCL)") -> (s? t:f=w1230:i16)
        n826 = Or(x="- phase (MCL)", y="+ phase (MCL)") -> (x .or. y?=w1225:bool)
        n827 = xnode "Read/Write Control"("FPGA VI Reference In"=w1234, "error in"=w1233, "Phase count adjustment (MCL)"=w1230) -> ("FPGA VI Reference Out"=w1226:T18, "error out"=w1227:errorcluster)
        n828 = xnode "Read/Write Control"("FPGA VI Reference In"=w1226, "error in"=w1227, "+ phase (MCL)"=w1225) -> ("error out"=w1224:errorcluster)  [unwired: 1 out]
      }
      event "Abort AOD Scan": Value Change {
        n829 = event-data() -> ()  [unwired: 7 out]
        n830 = flat-sequence {
          tunnel: w1239 -> [w1246]
          tunnel: w1238 -> [w1245]
          tunnel: [w1244] -> w1236
          tunnel: [w1240] -> w1235
          tunnel: [w1259] -> w1237
          tunnel: w1236 -> [w1259]
          tunnel: w1235 -> [w1258]
          frame #0 {
            n831 = local read "Save scans"() -> (w1242:bool)
            n832 = xnode "Read/Write Control"("FPGA VI Reference In"=w1246, "error in"=w1245, "Abort scan"="Abort AOD Scan") -> ("FPGA VI Reference Out"=w1240:T18, "error out"=w1244:errorcluster)
            n833 = case shown="True" w1242 {
              frame False {
              }
              frame True {
                n834 = local write "Stop Saving"(TRUE) -> ()
              }
            }
            n835 = local write "Raster Scanning..."(FALSE) -> ()
          }
          frame #1 {
            n836 = xnode "Read/Write Control"("FPGA VI Reference In"=w1258) -> ("BD1 Frequency Out 1"=w1249:u64)  [unwired: 1 in, 2 out]
            n837 = To Double Precision Float(number=w1249) -> (double precision float=w1255:dbl)
            n838 = Multiply(x=49125000.0, y=6.0) -> (x*y=w1254:dbl)
            n839 = Multiply(x=w1255, y=w1254) -> (x*y=w1252:dbl)
            n840 = Scale By Power Of 2(n=-48, x=w1252) -> (x*2^n=w1251:dbl)
            n841 = Divide(x=w1251, y=1000000.0) -> (x/y=w1248:dbl)
            n842 = property on="BD 1 Frq 1 (MHz)" class="DigNum (strict)"("Val(Sgnl)"=w1248) -> ()  [unwired: 2 in, 2 out]
          }
        }
      }
      event "Continuous AOD Scanning": Value Change {
        n843 = event-data() -> ()  [unwired: 7 out]
        n844 = xnode "Read/Write Control"("FPGA VI Reference In"=w1263, "error in"=w1262, "Cont. Scan"="Continuous AOD Scanning") -> ("error out"=w1261:errorcluster)  [unwired: 1 out]
      }
      event "Index": Value Change {
        n845 = event-data() -> ()  [unwired: 7 out]
        n846 = call "Create new save file.vi"("Insert"="", "Ext"=".dat" ("string"), "Index In"="Index") -> ("Path Out"=→"Save file name":path, "Index Out"=w1264:dbl)
        "Save index" <- w1264
        n847 = local write "Index"(w1264) -> ()
      }
      event "MCL Y", "MCL X": Value Change {
        n848 = event-data() -> ()  [unwired: 7 out]
        n849 = call "V2int16.vi"("InV"="MCL Y") -> ("Out i16"=w1272:i16)  [unwired: 4 in]
        n850 = call "V2int16.vi"("InV"="MCL X") -> ("Out i16"=w1269:i16)  [unwired: 4 in]
        n851 = xnode "Read/Write Control"("FPGA VI Reference In"=w1275, "error in"=w1274, "AO1 (Y)"=w1272, "AO2 (X)"=w1269) -> ("error out"=w1273:errorcluster)  [unwired: 1 out]
      }
      event "Inject Top": Value Change {
        n852 = event-data() -> ()  [unwired: 7 out]
        n853 = disable-structure shown="Disabled" {
          disable-tunnel: "Inject Top" -> [w1277 w1317]
          frame Disabled {
            n854 = local read item#-1() -> (w1278)
            n855 = local read item#-1() -> (w1279)
            n856 = case shown="True" w1277 {
              tunnel: w1279 -> [w1285 w1299]
              tunnel: w1278 -> [w1282 w1298]
              frame False {
                n857 = flat-sequence {
                  tunnel: w1282 -> [w1286]
                  tunnel: [w1286] -> w1283
                  tunnel: w1285 -> [_]
                  tunnel: [w1289] -> w1284
                  tunnel: w1283 -> [w1289]
                  tunnel: w1284 -> [w1290]
                  tunnel: [w1290] -> w1280
                  tunnel: [w1292] -> w1281
                  tunnel: w1280 -> [w1292]
                  tunnel: w1281 -> [w1294]
                  frame #0 {
                    n858 = call "Write to pump.vi"("string"="enter pump1", "VISA resource name"=w1286) -> ()  [unwired: 1 out]
                  }
                  frame #1 {
                    n859 = Wait (ms)() -> (milliseconds to wait=w1288:u32)  [unwired: 1 out]
                  }
                  frame #2 {
                    n860 = call "Write to pump.vi"("string"="stop", "VISA resource name"=w1290) -> ()  [unwired: 1 out]
                  }
                  frame #3 {
                    n861 = Wait (ms)(milliseconds to wait=u32 500) -> ()  [unwired: 1 out]
                  }
                  frame #4 {
                    n862 = call "Write to pump.vi"("string"="stop", "VISA resource name"=w1294) -> ()  [unwired: 1 out]
                  }
                }
              }
              frame True {
                n863 = flat-sequence {
                  tunnel: w1298 -> [w1308]
                  tunnel: w1299 -> [w1303]
                  tunnel: w1299 -> [w1310]
                  tunnel: w1298 -> [w1311]
                  tunnel: [w1311] -> w1296
                  tunnel: [w1313] -> w1297
                  tunnel: w1296 -> [w1313]
                  tunnel: w1297 -> [w1315]
                  frame #0 {
                    n864 = local read item#-1() -> (w1302)
                    n865 = Unbundle By Name(w1302) -> ("Pump 1"=w1309)
                    n866 = call "Set pump parameters.vi"("Pump write delay (ms)"=w1303, "Units"=4.0, "Pump #"=1.0, "Pump Parameters In"=w1309, "VISA resource name"=w1308) -> ("Pump Parameters Out"=w1301:T28, "Volume (uL)"=w1305:dbl, "Rate (uL/h)"=w1304:dbl)  [unwired: 3 in]
                    n867 = Bundle By Name(cluster=w1302, "Pump 1"=w1301) -> (w1300:cluster{})
                    n868 = local write item#-1(w1300) -> ()
                  }
                  frame #1 {
                    n869 = Wait (ms)(milliseconds to wait=w1310) -> ()  [unwired: 1 out]
                  }
                  frame #2 {
                    n870 = call "Write to pump.vi"("string"="start", "VISA resource name"=w1311) -> ()  [unwired: 1 out]
                  }
                  frame #3 {
                    n871 = Wait (ms)(milliseconds to wait=u32 500) -> ()  [unwired: 1 out]
                  }
                  frame #4 {
                    n872 = call "Write to pump.vi"("string"="start", "VISA resource name"=w1315) -> ()  [unwired: 1 out]
                  }
                }
              }
            }
          }
          frame Enabled {
            n873 = call "hamilton_controller.vi"("Open?"=w1317, "valve"=enum16{"A", "B", "C", "D", "ALL"}."B", "action"=T19."MOVE VALVE") -> ()  [unwired: 8 in, 1 out]
          }
        }
      }
      event "Inject Main": Value Change {
        n874 = event-data() -> ()  [unwired: 7 out]
        n875 = disable-structure shown="Disabled" {
          disable-tunnel: "Inject Main" -> [_ w1361]
          frame Disabled {
            n876 = local read item#-1() -> (w1322)
            n877 = case shown="False" w1323 {
              tunnel: w1322 -> [w1329 w1343]
              tunnel: [w1326 w1342] -> w1321
              frame False {
                n878 = flat-sequence {
                  tunnel: w1326 -> [w1330]
                  tunnel: [w1330] -> w1327
                  tunnel: w1329 -> [_]
                  tunnel: [w1333] -> w1328
                  tunnel: w1327 -> [w1333]
                  tunnel: w1328 -> [w1334]
                  tunnel: [w1334] -> w1324
                  tunnel: [w1336] -> w1325
                  tunnel: w1324 -> [w1336]
                  tunnel: w1325 -> [w1338]
                  frame #0 {
                    n879 = call "Write to pump.vi"("string"="enter pump3", "VISA resource name"=w1330) -> ()  [unwired: 1 out]
                  }
                  frame #1 {
                    n880 = local read item#-1() -> (w1332)
                    n881 = Wait (ms)(milliseconds to wait=w1332) -> ()  [unwired: 1 out]
                  }
                  frame #2 {
                    n882 = call "Write to pump.vi"("string"="stop", "VISA resource name"=w1334) -> ()  [unwired: 1 out]
                  }
                  frame #3 {
                    n883 = Wait (ms)(milliseconds to wait=u32 0) -> ()  [unwired: 1 out]
                  }
                  frame #4 {
                    n884 = call "Write to pump.vi"("string"="stop", "VISA resource name"=w1338) -> ()  [unwired: 1 out]
                  }
                }
              }
              frame True {
                n885 = flat-sequence {
                  tunnel: w1342 -> [w1352]
                  tunnel: w1343 -> [w1347]
                  tunnel: w1343 -> [w1354]
                  tunnel: w1342 -> [w1355]
                  tunnel: [w1355] -> w1340
                  tunnel: [w1358] -> w1341
                  tunnel: w1340 -> [w1358]
                  tunnel: w1341 -> [w1359]
                  frame #0 {
                    n886 = local read item#-1() -> (w1346)
                    n887 = Unbundle By Name(w1346) -> ("Pump 3"=w1353)
                    n888 = call "Set pump parameters.vi"("Pump write delay (ms)"=w1347, "Units"=4.0, "Pump #"=3.0, "Pump Parameters In"=w1353, "VISA resource name"=w1352) -> ("Pump Parameters Out"=w1345:T28, "Volume (uL)"=w1349:dbl, "Rate (uL/h)"=w1348:dbl)  [unwired: 3 in]
                    n889 = Bundle By Name(cluster=w1346, "Pump 3"=w1345) -> (w1344:cluster{})
                    n890 = local write item#-1(w1344) -> ()
                  }
                  frame #1 {
                    n891 = Wait (ms)(milliseconds to wait=w1354) -> ()  [unwired: 1 out]
                  }
                  frame #2 {
                    n892 = call "Write to pump.vi"("string"="start", "VISA resource name"=w1355) -> ()  [unwired: 1 out]
                  }
                  frame #3 {
                    n893 = Wait (ms)(milliseconds to wait=u32 500) -> ()  [unwired: 1 out]
                  }
                  frame #4 {
                    n894 = call "Write to pump.vi"("string"="start", "VISA resource name"=w1359) -> ()  [unwired: 1 out]
                  }
                }
              }
            }
          }
          frame Enabled {
            n895 = call "hamilton_controller.vi"("Open?"=w1361, "valve"=enum16{"A", "B", "C", "D", "ALL"}."A", "action"=T19."MOVE VALVE") -> ()  [unwired: 8 in, 1 out]
          }
        }
      }
      event "Inject Bottom": Value Change {
        n896 = event-data() -> ()  [unwired: 7 out]
        n897 = call "hamilton_controller.vi"("Open?"="Inject Bottom", "valve"=enum16{"A", "B", "C", "D", "ALL"}."C", "action"=T19."MOVE VALVE") -> ()  [unwired: 8 in, 1 out]
      }
      event "Shunt 1": Value Change {
        n898 = event-data() -> ()  [unwired: 7 out]
        n899 = call "hamilton_controller.vi"("Open?"="Shunt 1", "valve"=enum16{"A", "B", "C", "D", "ALL"}."D", "action"=T19."MOVE VALVE") -> ()  [unwired: 8 in, 1 out]
      }
      event "Shunt 2": Value Change {
        n900 = event-data() -> ()  [unwired: 7 out]
        n901 = call "hamilton_controller_shunt2.vi"("Open?"="Shunt 2", "valve"=enum16{"A", "B", "C", "D", "ALL", "E"}."E", "action"=T19."MOVE VALVE") -> ()  [unwired: 8 in, 1 out]
      }
      event "Flip Green Filter": Value Change {
        n902 = event-data() -> ()  [unwired: 7 out]
        n903 = local write "Flip Green Filter"("Flip Green Filter") -> ()
        n904 = flat-sequence {
          tunnel: w1380 -> [w1385]
          tunnel: w1379 -> [w1384]
          tunnel: [w1382] -> w1377
          tunnel: [w1381] -> w1376
          tunnel: [w1387] -> w1375
          tunnel: w1377 -> [w1387]
          tunnel: [w1386] -> w1374
          tunnel: w1376 -> [w1386]
          tunnel: w1375 -> [w1391]
          tunnel: w1374 -> [w1390]
          tunnel: [w1389] -> w1378
          frame #0 {
            n905 = xnode "Read/Write Control"("FPGA VI Reference In"=w1385, "error in"=w1384, "Green Filter Flipper"=TRUE) -> ("FPGA VI Reference Out"=w1382:T18, "error out"=w1381:errorcluster)
          }
          frame #1 {
            n906 = Wait (ms)(milliseconds to wait=u32 100) -> ()  [unwired: 1 out]
          }
          frame #2 {
            n907 = xnode "Read/Write Control"("FPGA VI Reference In"=w1391, "error in"=w1390, "Green Filter Flipper"=FALSE) -> ("error out"=w1389:errorcluster)  [unwired: 1 out]
          }
        }
      }
      event "Reset Trap Pos. FB": Value Change {
        n908 = event-data() -> ()  [unwired: 7 out]
        n909 = xnode "Read/Write Control"("FPGA VI Reference In"=w1395, "error in"=w1394, "Trap Pos. FB Reset"="Reset Trap Pos. FB") -> ()  [unwired: 2 out]
      }
      event "Trap Pos. FB ON": Value Change {
        n910 = event-data() -> ()  [unwired: 7 out]
        n911 = xnode "Read/Write Control"("FPGA VI Reference In"=w1410, "error in"=w1409) -> ("FPGA VI Reference Out"=w1407:T18, "BD1 Frequency Out 1"=w1404:u64)  [unwired: 1 out]
        n912 = To Double Precision Float(number=w1404) -> (double precision float=w1403:dbl)
        n913 = Multiply(x=49125000.0, y=6.0) -> (x*y=w1402:dbl)
        n914 = Multiply(x=w1403, y=w1402) -> (x*y=w1400:dbl)
        n915 = Scale By Power Of 2(n=-48, x=w1400) -> (x*2^n=w1399:dbl)
        n916 = Divide(x=w1399, y=1000000.0) -> (x/y=w1396:dbl)
        n917 = flat-sequence {
          tunnel: [w1413] -> w1408
          tunnel: w1407 -> [w1414]
          tunnel: w1404 -> [w1412]
          tunnel: "Trap Pos. FB ON" -> [w1411]
          tunnel: "Trap Pos. FB ON" -> [w1420]
          tunnel: w1408 -> [w1419]
          tunnel: "Trap Pos. FB ON" -> [w1422]
          tunnel: w1396 -> [w1421]
          frame #0 {
            n918 = case shown="False" w1411 {
              tunnel: w1414 -> [w1417 w1418]
              tunnel: [w1416 w1418] -> w1413
              tunnel: w1412 -> [w1415 _]
              frame False {
                n919 = xnode "Read/Write Control"("FPGA VI Reference In"=w1417, "BD 1 Frequency 1"=w1415) -> ("FPGA VI Reference Out"=w1416:T18)  [unwired: 1 in, 1 out]
              }
              frame True {
              }
            }
          }
          frame #1 {
            n920 = xnode "Read/Write Control"("FPGA VI Reference In"=w1419, "Force feedback"=w1420) -> ()  [unwired: 1 in, 2 out]
          }
          frame #2 {
            n921 = case shown="False" w1422 {
              tunnel: w1421 -> [w1425 _]
              frame False {
                n922 = local read "Asym. T2 (MHz)"() -> (w1423:dbl)
                n923 = Subtract(x=w1423, y=w1425) -> (x-y=w1424:dbl)
                n924 = property on="Trap Delta (MHz)" class="Slide (strict)"("Val(Sgnl)"=w1424) -> ()  [unwired: 2 in, 2 out]
              }
              frame True {
              }
            }
          }
        }
      }
      event "Diff. FB.", "Trap Pos. FB Gains", "Trap Pos. FB Mult Factor", "Trap Pos. FB Offset Factor", "Trap Pos FB Negate Action", "Trap Pos FB Monitor\nT1 or T2", "Negate Diff?": Value Change {
        n925 = event-data() -> ()  [unwired: 7 out]
        n926 = xnode "Read/Write Control"("FPGA VI Reference In"=w1436, "error in"=w1435, "Trap pos. FB Range"="Trap Pos. FB Range", "Trap Pos. FB Gains"="Trap Pos. FB Gains", "Trap Pos. FB Mult Factor"="Trap Pos. FB Mult Factor", "Trap Pos. FB Offset Factor"="Trap Pos. FB Offset Factor", "Trap Pos FB Negate Action"="Trap Pos FB Negate Action", "Trap Pos FB Monitor T1 or T2"="Trap Pos FB Monitor\nT1 or T2", "AI1 X Scale"="Trap Pos. AI1 X Pre-scale", "Negate Diff?"="Negate Diff?", "Diff FB Measurement?"="Diff. FB.") -> ()  [unwired: 2 out]
      }
      event "Trap Pos FB SP": Value Change {
        n927 = event-data() -> ()  [unwired: 7 out]
        n928 = xnode "Read/Write Control"("FPGA VI Reference In"=w1439, "error in"=w1438, "Trap Pos. FB SP"="Trap Pos FB SP") -> ()  [unwired: 2 out]
      }
      event "Set SP to Current Frc": Value Change {
        n929 = event-data() -> ()  [unwired: 7 out]
        n930 = local read "Trap Pos FB Monitor\nT1 or T2"() -> (w1447:bool)
        n931 = local read "Trap X AI1 (DMA)"() -> (w1450:T9)
        n932 = local read "FFB AvgX"() -> (w1453:T10)
        n933 = Unbundle By Name(w1453) -> ("Trap 1"=w1452:fxp<+/-,16,1>, "Trap 2"=w1451:fxp<+/-,16,1>)
        n934 = Unbundle By Name(w1450) -> ("Set 1"=w1449:fxp<+/-,16,1>, "Set 2"=w1448:fxp<+/-,16,1>)
        n935 = Select(t=w1452, s=w1447, f=w1451) -> (s? t:f=w1446:fxp<+/-,16,1>)
        n936 = Select(t=w1449, s=w1447, f=w1448) -> (s? t:f=w1445:fxp<+/-,16,1>)
        n937 = Not(x="Set SP Using...") -> (.not. x?=w1440:bool)
        n938 = Select(t=w1446, s=w1440, f=w1445) -> (s? t:f=w1441:fxp<+/-,16,1>)
        n939 = xnode "Read/Write Control"("FPGA VI Reference In"=w1443, "error in"=w1442, "Trap Pos. FB SP"=w1441) -> ()  [unwired: 2 out]
        n940 = local write "Trap Pos FB SP"(w1441) -> ()
      }
      event "Trap Pos. FB Out Scale 2^n": Value Change {
        n941 = event-data() -> ()  [unwired: 7 out]
        n942 = Scale By Power Of 2(n="Trap Pos. FB Out Scale 2^n", x=ext 1.0) -> (x*2^n=w1455:ext)
        n943 = property on="Trap Pos. FB Mult Factor" class="DigNum (strict)"("Val(Sgnl)"=w1455) -> ()  [unwired: 2 in, 2 out]
      }
      event "Trap Pos FB Int Count": Value Change {
        n944 = event-data() -> ()  [unwired: 7 out]
        n945 = xnode "Read/Write Control"("FPGA VI Reference In"=w1460, "error in"=w1459, "Trap Pos FB Int Count"="Trap Pos FB Int Count") -> ()  [unwired: 2 out]
      }
      event "Target Force (pN)", "Setpoint offset\nCorrection values", "Raster target force (pN)": Value Change {
        w1469 = 2.0
        n946 = event-data() -> ()  [unwired: 7 out]
        n947 = disable-structure "Removed B Factor to improve position feedback - Alex 081418 1of3" shown="Enabled" {
          disable-tunnel: [w1499 fxp<+/-,32,16> 1.0 ("B factor")] -> w1461
          frame Disabled {
            n948 = local read "B factor"() -> (w1500:dbl)
            n949 = To Fixed-Point(number=w1500) -> (fixed-point=w1499:fxp<+/-,16,16>)  [unwired: 1 in]
          }
          frame Enabled {
          }
        }
        n950 = xnode "Read/Write Control"("FPGA VI Reference In"=w1463, "B factor"=w1461) -> ("BD1 Frequency Out 1"=w1490:u64)  [unwired: 1 in, 2 out]
        n951 = local read "BD 1 Frq 2 (MHz)"() -> (w1489:dbl)
        n952 = local read "Target Force (pN)"() -> (w1475:dbl)
        n953 = To Double Precision Float(number=w1490) -> (double precision float=w1496:dbl)
        n954 = Multiply(x=49125000.0, y=6.0) -> (x*y=w1495:dbl)
        n955 = Multiply(x=w1496, y=w1495) -> (x*y=w1493:dbl)
        n956 = Scale By Power Of 2(n=-48, x=w1493) -> (x*2^n=w1492:dbl)
        n957 = Divide(x=w1492, y=1000000.0) -> (x/y=w1488:dbl)
        n958 = Subtract(x=w1489, y=w1488) -> (x-y=w1487:dbl)
        n959 = local read "T1 kaX (pN/nm)"() -> (w1476:dbl)
        n960 = local read "T1 alX (nm/V)"() -> (w1477:dbl)
        n961 = local read "Negate offset difference"() -> (w1478:bool)
        n962 = local read "Offset file step size"() -> (w1486:dbl)
        n963 = Multiply(x="Raster target force (pN)", y=w1469) -> (x*y=w1468:dbl)
        n964 = Multiply(x=w1475, y=w1469) -> (x*y=w1474:dbl)
        n965 = local read "Setpoint offset\nCorrection values"() -> (w1483:dbl[])
        n966 = Divide(x=w1487, y=w1486) -> (x/y=w1485:dbl)
        n967 = Select(t=-1, s=w1478, f=1) -> (s? t:f=w1479:i32)
        n968 = To Long Integer(number=w1485) -> (32bit integer=w1484:i32)
        n969 = Multiply(x=w1477, y=w1476) -> (x*y=w1467:dbl)
        n970 = Divide(x=w1474, y=w1467) -> (x/y=w1473:dbl)
        n971 = Index Array(array=w1483, index=w1484) -> (element=w1482:dbl)
        n972 = Divide(x=w1468, y=w1467) -> (x/y=w1466:dbl)
        n973 = Multiply(x=w1479, y=w1482) -> (x*y=w1465:dbl)
        n974 = Add(x=w1473, y=w1465) -> (x+y=w1472:dbl)
        n975 = Add(x=w1466, y=w1465) -> (x+y=w1464:dbl)
        n976 = To Fixed-Point(number=w1464) -> (fixed-point=w1462:fxp<+/-,16,1>)  [unwired: 1 in]
        n977 = To Fixed-Point(number=w1472) -> (fixed-point=w1471:fxp<+/-,16,1>)  [unwired: 1 in]
        n978 = property on="Trap Pos FB SP" class="DigNum (strict)"("Val(Sgnl)"=w1471) -> ()  [unwired: 2 in, 2 out]
        n979 = xnode "Read/Write Control"("FPGA VI Reference In"=w1463, "Raster setpoint"=w1462) -> ()  [unwired: 1 in, 2 out]
      }
      event "Read setpoint correction": Value Change {
        n980 = event-data() -> ()  [unwired: 7 out]
        n981 = local write "Read setpoint correction"(FALSE) -> ()
        n982 = Open/Create/Replace File(file path (use dialog)="Setpoint correction\noffset file", operation (0:open)=T24."open", access (0:read/write)=enum16{"read/write", "read-only", "write-only"}."read-only") -> (refnum out=w1527:refnum<file>)  [unwired: 1 in, 4 out]
        n983 = Deny Access(7:w1527) -> (3:w1525:refnum<file>)  [unwired: 1 in, 2 out]
        n984 = Read from Binary File(5:0.0, 9:T25."big-endian, network order" ("byte order (0:big-endian, network order)"), 10:-1 ("count (1)"), 11:w1525) -> (2:w1518:dbl[], 3:w1524:refnum<file>)  [unwired: 1 in, 3 out]
        n985 = Close File(refnum=w1524) -> ()  [unwired: 1 in, 2 out]
        n986 = Index Array(array=w1518, index=0) -> (element=w1514:dbl)
        n987 = local write "Offset file step size"(w1514) -> ()
        n988 = Array Subset(array=w1518, index=3) -> (w1517:dbl[])  [unwired: 1 in]
        n989 = local read "T1 kaX (pN/nm)"() -> (w1512:dbl)
        n990 = local read "T1 alX (nm/V)"() -> (w1513:dbl)
        n991 = local read "T2 alX (nm/V)"() -> (w1511:dbl)
        n992 = local read "T2 kaX (pN/nm)"() -> (w1510:dbl)
        n993 = Decimate 1D Array(w1517) -> (w1506:dbl[], w1507:dbl[])  [unwired: 1 out]
        n994 = local read "Offset Values"() -> (w1516:T14)
        n995 = Multiply(x=w1513, y=w1512) -> (x*y=w1508:dbl)
        n996 = Multiply(x=w1511, y=w1510) -> (x*y=w1509:dbl)
        n997 = Bundle By Name(cluster=w1516, "Trap 1X offset"=w1506, "Trap 2X offset"=w1507) -> (w1515:T14)
        n998 = Divide(x=w1509, y=w1508) -> (x/y=w1503:dbl)
        n999 = disable-structure "Removed B Factor to better position FB - Alex 081418 3of3" shown="Enabled" {
          disable-tunnel: w1503 -> [w1531 _]
          disable-tunnel: [w1531 1.0] -> w1502
          frame Disabled {
          }
          frame Enabled {
          }
        }
        n1000 = Multiply(x=w1507, y=w1502) -> (x*y=w1505:dbl[])
        n1001 = local write "Offset Values"(w1515) -> ()
        n1002 = Subtract(x=w1506, y=w1505) -> (x-y=w1504:dbl[])
        n1003 = property on="B factor" class="DigNum (strict)"("Val(Sgnl)"=w1502) -> ()  [unwired: 2 in, 2 out]
        n1004 = property on="Setpoint offset\nCorrection values" class="Arr (strict)"("Val(Sgnl)"=w1504) -> ()  [unwired: 2 in, 2 out]
      }
      event "MCL Tracking": Value Change {
        n1005 = event-data() -> ()  [unwired: 7 out]
        n1006 = case shown="False" "MCL Tracking" {
          frame False {
            n1007 = local read "Current MCL (V)"() -> (w1534:dbl)
            n1008 = local write "MCL X"(w1534) -> ()
          }
          frame True {
            n1009 = local read "BD 1 Frq 1 (MHz)"() -> (→"Zero T1 position":dbl)
            n1010 = local read "MCL X"() -> (→"Zero MCL x position":dbl)
          }
        }
      }
      event "Scale intensities (Q)": Value Change {
        n1011 = event-data() -> ()  [unwired: 7 out]
        n1012 = local read "Trap Powers (V)"() -> (w1540:cluster{"Set 1":dbl, "Set 2":dbl})
        n1013 = local read "T1 kaX (pN/nm)"() -> (w1546:dbl)
        n1014 = local read "T2 kaX (pN/nm)"() -> (w1545:dbl)
        n1015 = Unbundle By Name(w1540) -> ("Set 1"=w1542:dbl, "Set 2"=w1541:dbl)
        n1016 = case shown="False" "Scale intensities (Q)" {
          tunnel: "Scale factor" -> [w1549 w1558]
          tunnel: w1546 -> [w1557 w1566]
          tunnel: w1545 -> [w1556 w1565]
          tunnel: [w1554 w1564] -> w1544
          tunnel: [w1555 w1563] -> w1543
          tunnel: w1542 -> [w1553 w1562]
          tunnel: w1541 -> [w1552 w1561]
          tunnel: [w1551 w1560] -> w1539
          tunnel: [w1550 w1559] -> w1538
          frame False {
            n1017 = Divide(x=w1553, y=w1549) -> (x/y=w1551:dbl)
            n1018 = Divide(x=w1552, y=w1549) -> (x/y=w1550:dbl)
            n1019 = Divide(x=w1557, y=w1549) -> (x/y=w1554:dbl)
            n1020 = Divide(x=w1556, y=w1549) -> (x/y=w1555:dbl)
          }
          frame True {
            n1021 = Multiply(x=w1562, y=w1558) -> (x*y=w1560:dbl)
            n1022 = Multiply(x=w1561, y=w1558) -> (x*y=w1559:dbl)
            n1023 = Multiply(x=w1566, y=w1558) -> (x*y=w1564:dbl)
            n1024 = Multiply(x=w1558, y=w1565) -> (x*y=w1563:dbl)
          }
        }
        n1025 = Bundle By Name(cluster=w1540, "Set 1"=w1539, "Set 2"=w1538) -> (w1537:cluster{"Set 1":dbl, "Set 2":dbl})
        n1026 = local write "T1 kaX (pN/nm)"(w1544) -> ()
        n1027 = local write "T2 kaX (pN/nm)"(w1543) -> ()
        n1028 = property on="Trap Powers (V)" class="Clust (strict)"("Val(Sgnl)"=w1537) -> ()  [unwired: 2 in, 2 out]
      }
    }
    "Error Events" <- w646
  }
  n1029 = timed-loop "Acquire Data" {
    tunnel: w46 -> [w1759]
    tunnel: w54 -> [w1758]
    tunnel: [w1781] -> w49
    tunnel: [w1775] -> w12
    timing: w162 -> [_]
    timing-out: [_] -> w161
    tunnel: w69 -> [w1700]
    stop <- "Stop All" stop-if-true
    w1597 = 0.0
    # "The uint48 AOM Freq is sent as 3 u16s,\nCombine into one u64 (cant do u48)"
    # "The FIFO Read is noticeably slower when subVI'd,\nso keep it on the diagram"
    # "[Semi-passive would go here?]"
    # "Read values from FPGA"
    # "Check if we're done scanning"
    n1030 = First Call?() -> (First Call?: T/F=w1686:bool)
    n1031 = Or(x="Reset", y=w1686) -> (x .or. y?=w1687:bool)
    n1032 = case "Reset FIFOs if asked" shown="True" w1687 {
      tunnel: w1759 -> [w1895 w1904]
      tunnel: w1758 -> [w1894 w1903]
      tunnel: [w1895 w1898] -> w1673
      tunnel: [w1894 w1897] -> w1754
      frame False {
      }
      frame True {
        w1901 = TRUE ("AI to FIFO")
        n1033 = call "reset FPGA DMA.vi"("error in"=w1903, "FPGA VI Reference In"=w1904) -> ("error out"=w1899:errorcluster, "FPGA VI Reference Out"=w1900:T18)
        n1034 = local write "Overflow (data lost)"(FALSE ("Overflow (data lost)")) -> ()
        n1035 = xnode "Read/Write Control"("FPGA VI Reference In"=w1900, "error in"=w1899, "AI to FIFO"=w1901, "APD to FIFO"=w1901) -> ("FPGA VI Reference Out"=w1898:T18, "error out"=w1897:errorcluster)
        n1036 = local write "Reset"(FALSE ("Reset")) -> ()
      }
    }
    n1037 = Compound Arithmetic op=OR("Start MCL Scan", "Confocal Image", "Confocal Linescan") -> (w1725:bool)
    n1038 = Or(x="Start AOD Scan", y="Trap Raster") -> (x .or. y?=w1727:bool)
    n1039 = And(x="Save Data (MCL)", y=w1725) -> (x .and. y?=w1751:bool)
    n1040 = And(x="Save scans", y=w1727) -> (x .and. y?=w1752:bool)
    n1041 = case "Start AOM raster scan" shown="True" w1727 {
      tunnel: w1673 -> [w2037 w2048]
      tunnel: w1754 -> [w2036 w2047]
      tunnel: [w2037 w2041] -> w1672
      tunnel: [w2036 w2040] -> w1753
      frame False {
      }
      frame True {
        n1042 = local write "Trap Raster"(FALSE ("Trap Raster Scan")) -> ()
        n1043 = case shown="True" "Restart DMA? (AOD)" {
          tunnel: [w2088 w2090] -> w2042
          tunnel: [w2087 w2089] -> w2043
          tunnel: w2048 -> [w2088 w2092]
          tunnel: w2047 -> [w2087 w2091]
          frame False {
          }
          frame True {
            n1044 = call "reset FPGA DMA.vi"("error in"=w2091, "FPGA VI Reference In"=w2092) -> ("error out"=w2089:errorcluster, "FPGA VI Reference Out"=w2090:T18)
            n1045 = local write "Overflow (data lost)"(FALSE ("Overflow (data lost)")) -> ()
          }
        }
        n1046 = case shown="True" "Move MCL Also?" {
          tunnel: w2043 -> [w2052 w2082]
          tunnel: w2042 -> [w2053 w2083]
          tunnel: [w2051 w2086] -> w2041
          tunnel: [w2050 w2085] -> w2040
          tunnel: "Raster to target force?" -> [w2049 w2055]
          frame False {
            w2054 = TRUE ("AI to FIFO")
            n1047 = xnode "Read/Write Control"("FPGA VI Reference In"=w2053, "error in"=w2052, "AI to FIFO"=w2054, "APD to FIFO"=w2054, "Start scan"=w2054, "Raster to target force"=w2049) -> ("FPGA VI Reference Out"=w2051:T18, "error out"=w2050:errorcluster)
          }
          frame True {
            w2079 = FALSE ("1D or 2D Scan?")
            w2084 = TRUE ("AI to FIFO")
            # "V_int"
            n1048 = local read "Scan Range (nm)"() -> (w2061:dbl)
            n1049 = local read "N F/B Scans (AOD)"() -> (w2078:u16)
            n1050 = Sign(1:w2061) -> (0:w2060:dbl)
            n1051 = Compound Arithmetic op=MULTIPLY(w2061, "MCL Step Position Ratio", "MCL/AOM Scale Tweak") -> (w2065:dbl)
            n1052 = Negate(x=w2060) -> (-x=w2057:dbl)
            n1053 = Multiply(x=w2057, y="MCL Step Increment (V_int)") -> (x*y=w2059:dbl)
            n1054 = local read "Total Counts (ticks)"() -> (w2062:u32)
            n1055 = Divide(x=w2065, y="MCL X Cal (nm/V)") -> (x/y=w2071:dbl)
            n1056 = local read "Cycles/step (AOD)"() -> (w2073:u64)
            n1057 = local read "Scan steps (AOD)"() -> (w2074:u64)
            n1058 = Multiply(x=32767.0 ("y"), y=w2071) -> (x*y=w2077:dbl)
            n1059 = Divide(x=w2077, y=10.0) -> (x/y=w2070:dbl)
            n1060 = Divide(x=w2070, y="MCL Step Increment (V_int)") -> (x/y=w2068:dbl)
            n1061 = Absolute Value(x=w2068) -> (abs(x)=w2056:dbl)
            n1062 = Compound Arithmetic op=MULTIPLY(w2074, w2073, w2062) -> (w2069:u64)
            n1063 = Divide(x=w2069, y=w2056) -> (x/y=w2066:dbl)
            n1064 = xnode "Read/Write Control"("FPGA VI Reference In"=w2083, "error in"=w2082, "Scan steps (MCL)"=w2056, "Number of scans (MCL)"=w2078, "Cycles per step (MCL)"=u64 1, "Scan freq.  increment (MCL)"=w2059, "1D or 2D Scan?"=w2079, "MCL Scan Axis"=w2079, "Cont. Scan (MCL)"=w2079, "MCL count"=w2066) -> ("FPGA VI Reference Out"=w2081:T18, "error out"=w2080:errorcluster)
            n1065 = local write "Reset MCL after scan"(w2084) -> ()
            n1066 = xnode "Read/Write Control"("FPGA VI Reference In"=w2081, "error in"=w2080, "AI to FIFO"=w2084, "APD to FIFO"=w2084, "Start scan"=w2084, "Start scan (MCL)"=w2084, "Raster to target force"=w2055) -> ("FPGA VI Reference Out"=w2086:T18, "error out"=w2085:errorcluster)
            n1067 = local write "MCL Scanning"(w2084) -> ()
          }
        }
        "Raster Scanning..." <- TRUE ("Scanning...")
      }
    }
    n1068 = case "Start MCL raster scan" shown="True" w1725 {
      tunnel: w1672 -> [w1959 w1973]
      tunnel: w1753 -> [w1958 w1972]
      tunnel: [w1959 w1968] -> w1584
      tunnel: [w1958 w1967] -> w1583
      tunnel: [FALSE w1966] -> w1738
      tunnel: "Start MCL Scan" -> [_ w1961]
      tunnel: "Confocal Image" -> [_ w1960]
      frame False {
      }
      frame True {
        w1966 = TRUE
        n1069 = case shown="True" "Restart DMA? (MCL)" {
          tunnel: [w2017 w2019] -> w1971
          tunnel: [w2016 w2018] -> w1970
          tunnel: w1973 -> [w2017 w2022]
          tunnel: w1972 -> [w2016 w2021]
          frame False {
          }
          frame True {
            n1070 = call "reset FPGA DMA.vi"("error in"=w2021, "FPGA VI Reference In"=w2022) -> ("error out"=w2018:errorcluster, "FPGA VI Reference Out"=w2019:T18)
            n1071 = local write "Overflow (data lost)"(FALSE ("Overflow (data lost)")) -> ()
          }
        }
        n1072 = case shown="False" w1961 {
          tunnel: w1960 -> [w1976 _]
          frame False {
            n1073 = property on="Confocal Image" class="Bool (strict)"("Value"=FALSE ("Start Confocal Map")) -> ()  [unwired: 2 in, 2 out]
            n1074 = property on="2D or 1D Scan" class="Bool (strict)"("Val(Sgnl)"=w1976) -> ()  [unwired: 2 in, 2 out]
          }
          frame True {
          }
        }
        n1075 = local read "MCL X"() -> (w1962:dbl)
        n1076 = local read "MCL Y"() -> (w1963:dbl)
        n1077 = local write "MCL Scanning"(w1966) -> ()
        n1078 = case shown="True" "Center Scan" {
          tunnel: w1971 -> [w1983 w2015]
          tunnel: w1970 -> [w1982 w2014]
          tunnel: [w1981 w2013] -> w1968
          tunnel: [w1980 w2012] -> w1967
          tunnel: [w1978 w1987] -> w1965
          tunnel: [w1977 w1984] -> w1964
          tunnel: w1963 -> [w1978 w2004]
          tunnel: w1962 -> [w1977 w2007]
          frame False {
            w1979 = TRUE ("AI to FIFO")
            n1079 = xnode "Read/Write Control"("FPGA VI Reference In"=w1983, "error in"=w1982, "AI to FIFO"=w1979, "APD to FIFO"=w1979, "Start scan (MCL)"=w1979) -> ("FPGA VI Reference Out"=w1981:T18, "error out"=w1980:errorcluster)
          }
          frame True {
            w2011 = TRUE ("AI to FIFO")
            n1080 = local read "Scan steps (x)"() -> (w1994:u64)
            n1081 = local read "Fast Scan Dir"() -> (w2001:bool)
            n1082 = local read "Scan lines (y)"() -> (w1990:u64)
            n1083 = local read "Actual MCL Inc (V)"() -> (w1991:dbl)
            n1084 = Decrement(x=w1990) -> (x-1=w1989:u64)
            n1085 = Decrement(x=w1994) -> (x-1=w1993:u64)
            n1086 = Multiply(x=w1991, y=w1989) -> (x*y=w1988:dbl)
            n1087 = Divide(x=w1988, y=2.0) -> (x/y=w1998:dbl)
            n1088 = local read "2D or 1D Scan"() -> (w2009:bool)
            n1089 = Multiply(x=w1991, y=w1993) -> (x*y=w1992:dbl)
            n1090 = Divide(x=w1992, y=2.0) -> (x/y=w1997:dbl)
            n1091 = Select(t=w1997, s=w2001, f=w1998) -> (s? t:f=w1996:dbl)
            n1092 = Select(t=w1998, s=w2001, f=w1997) -> (s? t:f=w2000:dbl)
            n1093 = Subtract(x=w2004, y=w2000) -> (x-y=w1999:dbl)
            n1094 = Subtract(x=w2007, y=w1996) -> (x-y=w1995:dbl)
            n1095 = Not(x=w2001) -> (.not. x?=w2003:bool)
            n1096 = Not(x=w2009) -> (.not. x?=w2005:bool)
            n1097 = And(x=w2001, y=w2005) -> (x .and. y?=w2006:bool)
            n1098 = And(x=w2005, y=w2003) -> (x .and. y?=w2008:bool)
            n1099 = Select(t=w2007, s=w2008, f=w1995) -> (s? t:f=w1984:dbl)
            n1100 = Select(t=w2004, s=w2006, f=w1999) -> (s? t:f=w1987:dbl)
            n1101 = call "V2int16.vi"("InV"=w1984) -> ("Out i16"=w1985:i16)  [unwired: 4 in]
            n1102 = call "V2int16.vi"("InV"=w1987) -> ("Out i16"=w1986:i16)  [unwired: 4 in]
            n1103 = xnode "Read/Write Control"("FPGA VI Reference In"=w2015, "error in"=w2014, "AI to FIFO"=w2011, "APD to FIFO"=w2011, "Start scan (MCL)"=w2011, "AO1 (Y)"=w1986, "AO2 (X)"=w1985) -> ("FPGA VI Reference Out"=w2013:T18, "error out"=w2012:errorcluster)
          }
        }
        "Initial Y" <- w1965
        "Initial X" <- w1964
        "Reset MCL after scan" <- w1966
      }
    }
    n1104 = local read "TPos FIFO El/Read"() -> (w1577:u32)
    n1105 = local read "Trap FIFO El/Read"() -> (w1579:u32)
    n1106 = local read "APD FIFO El/Read"() -> (w1578:u32)
    n1107 = xnode "Invoke Method"("FPGA VI Reference In"=w1584, "error in"=w1583, "Number of Elements"=w1579, "Timeout (ms)"=-1 ("Timeout")) -> ("FPGA VI Reference Out"=w1581:T18, "error out"=w1582:errorcluster, "Data"=w1585:i16[], "Elements Remaining"=w1580:u32)
    "Trap FIFO El. Left" <- w1580
    n1108 = xnode ("Get APD Data")("FPGA VI Reference In"=w1584, "Number of Elements"=w1578, "Timeout (ms)"=-1) -> ("Data"=w1586:u32[], "Elements Remaining"=→"APD FIFO El Left":u32)  [unwired: 1 in, 2 out]
    n1109 = xnode "Invoke Method"("FPGA VI Reference In"=w1584, "Number of Elements"=w1577, "Timeout (ms)"=-1) -> ("Data"=w1574:u16[], "Elements Remaining"=→"TPos FIFO El Left":u32)  [unwired: 1 in, 2 out]
    n1110 = local read "Trap AI FIFO Depth"() -> (w1790:u32)
    n1111 = xnode "Read/Write Control"("FPGA VI Reference In"=w1581, "error in"=w1582) -> ("FPGA VI Reference Out"=w1669:T18, "error out"=w1662:errorcluster, "BD1 Frequency Out 1"=w1658:u64)
    n1112 = Subtract(x=w1790, y=w1579) -> (x-y=w1789:u32)
    n1113 = flat-sequence "Save data" {
      tunnel: [w2217] -> w1792
      tunnel: [w2218] -> w1791
      tunnel: w1752 -> [w2213]
      tunnel: w1573 -> [w2216]
      tunnel: w1661 -> [w2192]
      tunnel: [w2211] -> w1763
      tunnel: [w2208] -> w1762
      tunnel: [w2205] -> w1761
      tunnel: w1751 -> [w2207]
      tunnel: [w2197] -> w1685
      tunnel: [w2196] -> w1684
      tunnel: w1629 -> [w2190]
      tunnel: w1792 -> [w2367]
      tunnel: w1791 -> [w2366]
      tunnel: w1656 -> [w2365]
      tunnel: w1763 -> [w2363]
      tunnel: w1762 -> [w2362]
      tunnel: w1761 -> [w2361]
      tunnel: w1685 -> [w2360]
      tunnel: w1684 -> [w2359]
      tunnel: w1587 -> [w2358]
      tunnel: w1586 -> [w2357]
      tunnel: w1629 -> [w2356]
      frame #0 {
        # "Channel Pattern, N Channels, dT"
        n1114 = Or(x="Save N Sets", y="Start Saving") -> (x .or. y?=w2202:bool)
        n1115 = Build Array(w2202, "Save Calibration", w2213, w2207) -> (w2215:bool[])
        n1116 = Boolean Array To Number(Boolean array=w2215) -> (number=w2194:u32)
        n1117 = Not Equal To 0?(x=w2194) -> (x != 0?=w2193:bool)
        n1118 = feedback #1(refnum<k0> refnum) -> (w2219:refnum<file>)
        n1119 = feedback #2(0) -> (w2221:i32)
        n1120 = feedback #3(u32 0 ("Cal sets to save")) -> (w2212:u32)
        n1121 = feedback #4(refnum<k0> refnum) -> (w2209:refnum<file>)
        n1122 = feedback #5(FALSE ("Save APD Data\nwith Trap Data")) -> (w2206:bool)
        n1123 = feedback #6(refnum<k0> refnum) -> (w2200:refnum<file>)
        n1124 = feedback #7(FALSE ("Save APD Data\nwith Trap Data")) -> (w2198:bool)
        n1125 = case shown="True" w2193 {
          tunnel: [w2229 1] -> w2217
          tunnel: w2221 -> [w2230 _]
          tunnel: [w2223 w2245] -> w2218
          tunnel: w2219 -> [w2223 _]
          tunnel: w2216 -> [_ w2239]
          tunnel: w2194 -> [_ w2241]
          tunnel: [w2228 w2256] -> w2211
          tunnel: w2212 -> [w2228 _]
          tunnel: [w2227 w2255] -> w2208
          tunnel: w2209 -> [w2227 _]
          tunnel: [w2226 w2254] -> w2205
          tunnel: w2206 -> [w2226 _]
          tunnel: [w2225 w2250] -> w2196
          tunnel: w2200 -> [w2225 _]
          tunnel: [w2224 w2249] -> w2197
          tunnel: w2198 -> [w2224 _]
          tunnel: "Start Saving" -> [_ w2248]
          tunnel: w2192 -> [_ w2235]
          tunnel: w2190 -> [_ w2233]
          frame False {
            n1126 = Increment(x=w2230) -> (x+1=w2229:i32)
          }
          frame True {
            w2253 = FALSE ("Start Saving")
            w2240 = 9.0  # File Ver.
            n1127 = To Double Precision Float(number=w2235) -> (double precision float=w2234:dbl)
            n1128 = To Double Precision Float(number=w2233) -> (double precision float=w2232:dbl)
            n1129 = case "File Info Header" shown="Default" w2241 {
              tunnel: w2240 -> [w2269 w2276]
              tunnel: w2239 -> [w2268 w2271]
              tunnel: w2232 -> [w2267 w2275]
              tunnel: w2234 -> [w2266 w2274]
              tunnel: [w2265 w2273] -> w2238
              frame 2 {
                n1130 = Build Array(w2269, w2268, w2268, w2267, w2266) -> (w2265:dbl[])
              }
              frame Default {
                n1131 = local read "Save ave N"() -> (w2272:i32)
                n1132 = Multiply(x=w2271, y=w2272) -> (x*y=w2270:dbl)
                n1133 = Build Array(w2276, w2271, w2270, w2275, w2274) -> (w2273:dbl[])
              }
            }
            n1134 = case "Scan Info Header" shown="1, Default" w2241 {
              tunnel: [w2294 "Cal sets" w2313 w2344] -> w2256
              tunnel: "Save APD" -> [w2288 _ w2308 w2331]
              tunnel: [w2288 w2300 w2308 w2331] -> w2254
              tunnel: [w2287 w2300 w2307 w2330] -> w2249
              tunnel: "Save TPos" -> [w2287 _ w2307 w2330]
              tunnel: w2248 -> [w2291 _ _ _]
              tunnel: [0.0 ("f") 1.0 ("t") 2.0 ("t") 3.0 ("t")] -> w2237
              tunnel: [w2285 w2297 w2303 w2326] -> w2231
              frame 1, Default {
                w2292 = 0.0 ("f")
                # "Regular Data"
                n1135 = Build Array(w2288, w2287) -> (w2289:bool[])
                n1136 = Boolean Array To Number(Boolean array=w2289) -> (number=w2286:u32)
                n1137 = To Double Precision Float(number=w2286) -> (double precision float=w2296:dbl)
                n1138 = Select(t=u32 4000000000, s=w2291, f="N sets to save") -> (s? t:f=w2294:u32)
                n1139 = Build Array(w2296, w2292, w2292, w2292, w2292) -> (w2285:dbl[])
              }
              frame 2 {
                w2298 = 0.0 ("f")
                w2300 = FALSE ("Save APD Data\nwith Trap Data")
                # "Calibration"
                n1140 = Build Array(w2298, w2298, w2298, w2298, w2298) -> (w2297:dbl[])
                "Calibrating..." <- TRUE ("Calibrating...")
              }
              frame 4 {
                w2311 = 0.0 ("f")
                # "Trap Raster"
                n1141 = local read "N F/B Scans (AOD)"() -> (w2317:u16)
                n1142 = Build Array(w2308, w2307) -> (w2306:bool[])
                n1143 = local read "Scan Range (MHz)"() -> (w2322:dbl)
                n1144 = local read "Cycles/step (AOD)"() -> (w2319:u64)
                n1145 = local read "Scan steps (AOD)"() -> (w2321:u64)
                n1146 = Boolean Array To Number(Boolean array=w2306) -> (number=w2309:u32)
                n1147 = To Double Precision Float(number=w2309) -> (double precision float=w2312:dbl)
                n1148 = local read "Scan BD"() -> (w2325:bool)
                n1149 = local read "Trap Raster N Sets"() -> (w2314:dbl)
                n1150 = Build Array(w2312, w2311, w2311, w2311, w2311) -> (w2305:dbl[])
                n1151 = Boolean To (0,1)(Boolean=w2325) -> (0, 1=w2324:i16)
                n1152 = To Double Precision Float(number=w2321) -> (double precision float=w2320:dbl)
                n1153 = To Double Precision Float(number=w2319) -> (double precision float=w2318:dbl)
                n1154 = To Double Precision Float(number=w2317) -> (double precision float=w2316:dbl)
                n1155 = To Double Precision Float(number=w2324) -> (double precision float=w2323:dbl)
                n1156 = Build Array(w2323, w2322, w2320, w2318, w2316) -> (w2304:dbl[])
                n1157 = Round Toward +Infinity(x=w2314) -> (ceil(x): smallest int >= x=w2315:dbl)
                n1158 = Build Array (concatenate)(w2305, w2304) -> (w2303:dbl[])
                n1159 = To Unsigned Long Integer(number=w2315) -> (unsigned 32bit integer=w2313:u32)
              }
              frame 8 {
                w2340 = 0.0 ("f")
                # "MCL raster scan"
                n1160 = local read "2D or 1D Scan"() -> (w2337:bool)
                n1161 = Build Array(w2331, w2330) -> (w2332:bool[])
                n1162 = local read "MCL Scan N Sets"() -> (w2345:dbl)
                n1163 = Boolean Array To Number(Boolean array=w2332) -> (number=w2329:u32)
                n1164 = To Double Precision Float(number=w2329) -> (double precision float=w2343:dbl)
                n1165 = local read "Number of scans (MCL)"() -> (w2335:u64)
                n1166 = Boolean To (0,1)(Boolean=w2337) -> (0, 1=w2339:i16)
                n1167 = local read "Scan Range (V)"() -> (w2352:dbl)
                n1168 = To Double Precision Float(number=w2339) -> (double precision float=w2338:dbl)
                n1169 = local read "Cycles/step (MCL)"() -> (w2349:u64)
                n1170 = Build Array(w2343, w2338, w2340, w2340, w2340) -> (w2328:dbl[])
                n1171 = local read "Scan steps (x)"() -> (w2351:u64)
                n1172 = local read "Scan lines (y)"() -> (w2334:u64)
                n1173 = local read "Fast Scan Dir"() -> (w2355:bool)
                n1174 = local read "Initial X"() -> (w2342:dbl)
                n1175 = local read "Initial Y"() -> (w2341:dbl)
                n1176 = Round Toward +Infinity(x=w2345) -> (ceil(x): smallest int >= x=w2346:dbl)
                n1177 = To Unsigned Long Integer(number=w2346) -> (unsigned 32bit integer=w2344:u32)
                n1178 = To Double Precision Float(number=w2351) -> (double precision float=w2350:dbl)
                n1179 = To Double Precision Float(number=w2349) -> (double precision float=w2348:dbl)
                n1180 = Select(t=w2334, s=w2337, f=w2335) -> (s? t:f=w2336:u64)
                n1181 = Boolean To (0,1)(Boolean=w2355) -> (0, 1=w2354:i16)
                n1182 = To Double Precision Float(number=w2354) -> (double precision float=w2353:dbl)
                n1183 = To Double Precision Float(number=w2336) -> (double precision float=w2347:dbl)
                n1184 = Build Array(w2353, w2352, w2350, w2348, w2347, w2342, w2341) -> (w2327:dbl[])
                n1185 = Build Array (concatenate)(w2328, w2327) -> (w2326:dbl[])
              }
            }
            n1186 = local read "BD 1 Frq 1 (MHz)"() -> (w2262:dbl)
            n1187 = local read "BD 2 Frq 1 (MHz)"() -> (w2261:dbl)
            n1188 = local read "BD 1 Frq 2 (MHz)"() -> (w2260:dbl)
            n1189 = local read "BD 2 Frq 2 (MHz)"() -> (w2259:dbl)
            n1190 = local read "BD 1 Frq 3 (MHz)"() -> (w2258:dbl)
            n1191 = local read "BD 2 Frq 3 (MHz)"() -> (w2257:dbl)
            n1192 = Build Array(w2262, w2261, w2260, w2259, w2258, w2257) -> (w2242:dbl[])
            n1193 = local write "Saving..."(TRUE ("Saving...")) -> ()
            n1194 = local write "Save Calibration"(w2253) -> ()
            n1195 = local write "Start Saving"(w2253) -> ()
            n1196 = Build Array (concatenate)(w2238, w2237) -> (w2236:dbl[])
            n1197 = local read "Index"() -> (w2247:dbl)
            n1198 = call "HeaderTrap.vi"("Index In"=w2247, "File Info"=w2236, "BD Frqs"=w2242, "Scan Data"=w2231, "Comment"="Comment") -> ("Index Out"=w2246:dbl, "Trap Path"=w2244:path, "Trap File Out"=w2245:refnum<file>)  [unwired: 12 in]
            n1199 = local write "Index"(w2246) -> ()
            n1200 = local write "Save index"(w2246) -> ()
            n1201 = local write "Save file name"(w2244) -> ()
            n1202 = case "Fluorescence Header" shown="True" w2254 {
              tunnel: w2244 -> [_ w2282]
              tunnel: [refnum<k0> refnum w2281] -> w2255
              frame False {
              }
              frame True {
                n1203 = local read "APD Integration Time (s)"() -> (w2284:dbl)
                n1204 = local read "N APD Samp/step"() -> (w2283:i32)
                n1205 = call "HeaderFluorescence.vi"("N APD Samp/step"=w2283, "APD Integration Time (s)"=w2284, "Trap Path"=w2282) -> ("Flu File"=w2281:refnum<file>)  [unwired: 8 in]
              }
            }
            n1206 = case "TPos Header" shown="True" w2249 {
              tunnel: w2244 -> [_ w2279]
              tunnel: [refnum<k0> refnum w2278] -> w2250
              frame False {
              }
              frame True {
                n1207 = call "HeaderTPos.vi"("Trap Path"=w2279) -> ("TPos File"=w2278:refnum<file>)  [unwired: 10 in]
              }
            }
          }
        }
        n1208 = feedback-in #1(w2218) -> ()
        n1209 = feedback-in #2(w2217) -> ()
        n1210 = feedback-in #3(w2211) -> ()
        n1211 = feedback-in #4(w2208) -> ()
        n1212 = feedback-in #5(w2205) -> ()
        n1213 = feedback-in #6(w2196) -> ()
        n1214 = feedback-in #7(w2197) -> ()
      }
      frame #1 {
        # "N Channels"
        # "TPos, APD, Trap Data"
        n1215 = local read "Saving..."() -> (w2364:bool)
        n1216 = case shown="True" w2364 {
          tunnel: w2367 -> [_ w2371]
          tunnel: w2366 -> [_ w2390]
          tunnel: w2365 -> [_ w2386]
          tunnel: w2363 -> [_ w2370]
          tunnel: w2362 -> [_ w2382]
          tunnel: w2361 -> [_ w2381]
          tunnel: w2360 -> [_ w2379]
          tunnel: w2359 -> [_ w2378]
          tunnel: w2358 -> [_ w2377]
          tunnel: w2357 -> [_ w2376]
          tunnel: w2356 -> [_ w2375]
          frame False {
          }
          frame True {
            n1217 = local read "DMA Update Period (s)"() -> (w2374:dbl)
            n1218 = Divide(x=w2371, y=w2370) -> (x/y=w2373:dbl)
            n1219 = Multiply(x=w2371, y=w2374) -> (x*y=→"Time (s)":dbl)
            n1220 = Less Or Equal?(x=w2371, y=w2370) -> (x <= y?=w2388:bool)
            n1221 = Multiply(x=w2373, y=100.0) -> (x*y=w2369:dbl)
            n1222 = Or(x="Stop Saving", y="Abort save 2") -> (x .or. y?=w2383:bool)
            n1223 = Not(x=w2383) -> (.not. x?=w2389:bool)
            n1224 = And(x=w2388, y=w2389) -> (x .and. y?=w2387:bool)
            n1225 = case shown="True" w2387 {
              tunnel: w2390 -> [w2397 w2418]
              tunnel: w2386 -> [_ w2415]
              tunnel: w2382 -> [w2396 w2411]
              tunnel: w2381 -> [w2395 w2412]
              tunnel: w2379 -> [w2393 w2410]
              tunnel: w2378 -> [w2394 w2409]
              tunnel: w2377 -> [_ w2407]
              tunnel: w2376 -> [_ w2405]
              tunnel: w2375 -> [_ w2404]
              tunnel: w2369 -> [_ w2400]
              tunnel: [0.0 w2400] -> w2368
              frame False {
                w2392 = FALSE
                n1226 = case shown="True" w2395 {
                  tunnel: w2396 -> [_ w2399]
                  frame False {
                  }
                  frame True {
                    n1227 = Close File(refnum=w2399) -> ()  [unwired: 1 in, 2 out]
                  }
                }
                n1228 = case shown="False" w2393 {
                  tunnel: w2394 -> [_ w2398]
                  frame False {
                  }
                  frame True {
                    n1229 = Close File(refnum=w2398) -> ()  [unwired: 1 in, 2 out]
                  }
                }
                n1230 = Close File(refnum=w2397) -> ()  [unwired: 1 in, 2 out]
                n1231 = call <vilib>:"Beep.vi"() -> ()  [unwired: 3 in, 9 out]
                n1232 = property on="Raster Scanning..." class="Bool (strict)"("Val(Sgnl)"=w2392) -> ()  [unwired: 2 in, 2 out]
                n1233 = local write "Stop Saving"(w2392) -> ()
                n1234 = local write "Calibrating..."(w2392) -> ()
                "Saving..." <- w2392
              }
              frame True {
                n1235 = local read "Calibrating..."() -> (w2403:bool)
                n1236 = Equal?(x=1 ("y"), y="Save ave N") -> (x = y?=w2414:bool)
                n1237 = Or(x=w2403, y=w2414) -> (x .or. y?=w2408:bool)
                n1238 = case "Downsample TPos" shown="False" w2408 {
                  tunnel: w2407 -> [w2429 w2433]
                  tunnel: [w2421 w2433] -> w2406
                  tunnel: "Save ave N" -> [w2422 _]
                  frame False {
                    w2419 = 2 ("dimension size")
                    n1239 = Array Size(array=w2429) -> (size(s)=w2423:i32)
                    n1240 = Divide(x=w2423, y=w2419) -> (x/y=w2427:dbl)
                    n1241 = Divide(x=w2423, y=w2422) -> (x/y=w2424:dbl)
                    n1242 = Reshape Array(w2429, w2427, w2419) -> (w2428:u64[][])
                    n1243 = Transpose 2D Array(2D array=w2428) -> (transposed array=w2426:u64[][])
                    n1244 = for {
                      tunnel: w2426 -> [w2431] mode=indexing
                      tunnel: [w2430] -> w2420 mode=indexing
                      tunnel: w2422 -> [w2432]
                      workers-P: _ -> [_]
                      n1245 = call "downsample 1D array - U64.vi"("Ave N"=w2432, "Array In"=w2431) -> ("Array Out"=w2430:u64[])  [unwired: 1 in]
                    }
                    n1246 = Transpose 2D Array(2D array=w2420) -> (transposed array=w2425:u64[][])
                    n1247 = Reshape Array(w2425, w2424) -> (w2421:u64[])
                  }
                  frame True {
                  }
                }
                n1248 = case "Downsample Trap" shown="False" w2408 {
                  tunnel: w2415 -> [w2452 w2456]
                  tunnel: [w2444 w2456] -> w2413
                  tunnel: "Save ave N" -> [w2445 _]
                  tunnel: w2404 -> [w2442 _]
                  frame False {
                    n1249 = Array Size(array=w2452) -> (size(s)=w2446:i32)
                    n1250 = Quotient & Remainder(x=w2446, y=w2442) -> (floor(x/y)=w2450:i32)  [unwired: 1 out]
                    n1251 = Quotient & Remainder(x=w2446, y=w2445) -> (floor(x/y)=w2447:i32)  [unwired: 1 out]
                    n1252 = Reshape Array(w2452, w2450, w2442) -> (w2451:i16[][])
                    n1253 = Transpose 2D Array(2D array=w2451) -> (transposed array=w2449:i16[][])
                    n1254 = for {
                      tunnel: w2449 -> [w2455] mode=indexing
                      tunnel: [w2454] -> w2443 mode=indexing
                      tunnel: w2445 -> [w2453]
                      workers-P: _ -> [_]
                      n1255 = call "downsample 1D array - I16.vi"("Ave N"=w2453, "Array In"=w2455) -> ("Array Out"=w2454:i16[])  [unwired: 1 out]
                    }
                    n1256 = Transpose 2D Array(2D array=w2443) -> (transposed array=w2448:i16[][])
                    n1257 = Reshape Array(w2448, w2447) -> (w2444:i16[])
                  }
                  frame True {
                    # "Don't downsample"
                  }
                }
                n1258 = case "Write fluorescene" shown="True" w2412 {
                  tunnel: w2411 -> [_ w2439]
                  tunnel: w2405 -> [_ w2438]
                  frame False {
                  }
                  frame True {
                    n1259 = Write to Binary File(file (use dialog)=w2439, data=w2438, 5:FALSE ("prepend array or string size? (T)"), 9:T25."big-endian, network order" ("byte order (0:big-endian, network order)")) -> ()  [unwired: 1 in, 4 out]
                  }
                }
                n1260 = case "Save TPos Data" shown="True" w2410 {
                  tunnel: w2409 -> [_ w2435]
                  tunnel: w2406 -> [_ w2434]
                  frame False {
                  }
                  frame True {
                    n1261 = Write to Binary File(file (use dialog)=w2435, data=w2434, 5:FALSE ("prepend array or string size? (T)"), 9:T25."big-endian, network order" ("byte order (0:big-endian, network order)")) -> ()  [unwired: 1 in, 4 out]
                  }
                }
                n1262 = Write to Binary File "Save Trap Data"(file (use dialog)=w2418, data=w2413, 5:FALSE ("prepend array or string size? (T)"), 9:T25."big-endian, network order" ("byte order (0:big-endian, network order)")) -> ()  [unwired: 1 in, 4 out]
              }
            }
            "Progress" <- w2368
            "Progress 2" <- w2368
          }
        }
      }
    }
    n1263 = local read "BD 1 Frq 2 (MHz)"() -> (w1679:dbl)
    n1264 = Divide(x=w1580, y=w1789) -> (x/y=w1788:dbl)
    "Buffer Status" <- w1788
    n1265 = local read "MCL Tracking"() -> (w1674:bool)
    n1266 = Equal?(x=w1788, y=1.0) -> (x = y?=w1786:bool)
    n1267 = call "AODuint642MHz.vi"("In u64"=w1658) -> ("Out MHz"=w1657:dbl)  [unwired: 4 in]
    n1268 = Decimate 1D Array(w1574) -> (w1590:u16[], w1591:u16[], w1592:u16[])
    n1269 = To Unsigned Long Integer(number=w1590) -> (unsigned 32bit integer=w1589:u32[])
    n1270 = Join Numbers(hi=w1591, lo=w1592) -> ((hi.lo)=w1588:u32[])
    n1271 = Subtract ("TD")(x=w1679, y=w1657) -> (x-y=w1670:dbl)
    "Current Trap Delta" <- w1670
    n1272 = case shown="True" w1674 {
      tunnel: w1657 -> [_ w1872]
      tunnel: w1672 -> [_ w1862]
      frame False {
      }
      frame True {
        n1273 = local read "Zero T1 position"() -> (w1871:dbl)
        n1274 = local read "AOM X Cal (nm/MHz)"() -> (w1869:dbl)
        n1275 = local read "MCL X Cal (nm/V)"() -> (w1865:dbl)
        n1276 = Subtract(x=w1872, y=w1871) -> (x-y=w1870:dbl)
        n1277 = local read "Zero MCL x position"() -> (w1864:dbl)
        n1278 = Multiply(x=w1870, y=w1869) -> (x*y=w1868:dbl)
        n1279 = Multiply(x=w1868, y="Tracking factor") -> (x*y=w1866:dbl)
        n1280 = Divide(x=w1866, y=w1865) -> (x/y=w1863:dbl)
        n1281 = Add(x=w1864, y=w1863) -> (x+y=w1861:dbl)
        "Current MCL (V)" <- w1861
        n1282 = call "V2int16.vi"("InV"=w1861) -> ("Out i16"=w1860:i16)  [unwired: 4 in]
        n1283 = xnode "Read/Write Control"("FPGA VI Reference In"=w1862, "AO2 (X)"=w1860) -> ()  [unwired: 1 in, 2 out]
      }
    }
    n1284 = case "Alert buffer overflow" shown="True" w1786 {
      frame False {
      }
      frame True {
        n1285 = call <vilib>:"Beep.vi"() -> ()  [unwired: 3 in, 9 out]
        "Overflow (data lost)" <- TRUE ("Overflow (data lost)")
      }
    }
    n1286 = Join Numbers(hi=w1589, lo=w1588) -> ((hi.lo)=w1587:u64[])
    n1287 = call "IR AOM word to freq - vec.vi"("Frequency Word In (double vec)"=w1587) -> ("Frequency Out"=w1698:dbl[])
    n1288 = Decimate 1D Array(w1698) -> (w1697:dbl[], w1696:dbl[])
    n1289 = Build Array(w1697, w1696) -> (w1644:dbl[][])
    n1290 = local read "Dynamic Force FB"() -> (w1678:bool)
    n1291 = local read "Trap Pos. FB ON"() -> (w1677:bool)
    n1292 = local read "Trap Sets"() -> (w1660:u32)
    n1293 = call "Trapu16toDbl.vi"("Detector Type"="Detector Type", "Trap Sets"=w1660, "Raw Trap Data In"=w1585) -> ("Channel pattern"=w1661:i32, "Channel Names"=w1630:string[], "Trap Data"=w1650:dbl[][], "Trap Data Out"=w1656:i16[])  [unwired: 5 in]
    "AI labels" <- w1630
    n1294 = Compound Arithmetic op=AND(w1678, w1677, "Use Offset in FFB?") -> (w1675:bool)
    n1295 = local read "Trap X AI1 (DMA)"() -> (w1692:T9)
    n1296 = case "Apply Offset to Force Feedback" shown="True" w1675 {
      tunnel: w1670 -> [_ w1875]
      tunnel: w1669 -> [_ w1874]
      frame False {
      }
      frame True {
        n1297 = local read "Setpoint offset\nCorrection values"() -> (w1890:dbl[])
        n1298 = local read "Offset file step size"() -> (w1893:dbl)
        n1299 = local read "Negate offset difference"() -> (w1885:bool)
        n1300 = local read "T1 kaX (pN/nm)"() -> (w1883:dbl)
        n1301 = local read "T1 alX (nm/V)"() -> (w1884:dbl)
        n1302 = Divide(x=w1875, y=w1893) -> (x/y=w1892:dbl)
        n1303 = Multiply(x="Target Force (pN)", y=2.0) -> (x*y=w1881:dbl)
        n1304 = Multiply(x=w1884, y=w1883) -> (x*y=w1880:dbl)
        n1305 = To Long Integer(number=w1892) -> (32bit integer=w1891:i32)
        n1306 = Divide(x=w1881, y=w1880) -> (x/y=w1879:dbl)
        n1307 = Select(t=-1, s=w1885, f=1) -> (s? t:f=w1886:i32)
        n1308 = Index Array(array=w1890, index=w1891) -> (element=w1889:dbl)
        n1309 = Multiply(x=w1886, y=w1889) -> (x*y=w1878:dbl)
        n1310 = Add(x=w1879, y=w1878) -> (x+y=w1877:dbl)
        n1311 = To Fixed-Point(number=w1877) -> (fixed-point=w1873:fxp<+/-,16,1>)  [unwired: 1 in]
        "Actual setpoint" <- w1873
        n1312 = xnode "Read/Write Control"("FPGA VI Reference In"=w1874, "Trap Pos. FB SP"=w1873) -> ()  [unwired: 1 in, 2 out]
      }
    }
    n1313 = Array Size(array=w1630) -> (size(s)=w1629:i32)
    n1314 = call "Trapi162FXP.vi"("N El. to Ave."="N El. to Ave.", "Trap Data"=w1656) -> ("Trap 2"=w1653:fxp<+/-,16,1>, "Trap 1"=w1654:fxp<+/-,16,1>)  [unwired: 8 in]
    n1315 = Bundle By Name(cluster=w1692, "Set 1"=w1654, "Set 2"=w1653) -> (→"Trap X AI1 (DMA)":T9)
    n1316 = case shown="True" "Read Lateness and Rel Phase" {
      tunnel: w1669 -> [w1906 w1927]
      tunnel: [w1906 w1926] -> w1717
      tunnel: [w1905 w1925] -> w1716
      tunnel: w1662 -> [w1905 w1909]
      frame False {
      }
      frame True {
        n1317 = xnode "Read/Write Control"("FPGA VI Reference In"=w1927, "error in"=w1909) -> ("FPGA VI Reference Out"=w1926:T18, "error out"=w1925:errorcluster, "GI Relative phase"=→"GI relative phase":i16, "Relative phase"=→"Relative phase (AI1)":i16, "AI Late Counter"=→"Late Counter (AI1)":u8, "GI Late Counter"=→"GI Late Counter":u8, "MCL Late Counter"=→"MCL Late Counter":u8, "MCL Relative Phase"=→"Relative Phase (MCL)":i16, "APD Acq Relative Phase"=→"APD Acq Relative Phase":i16, "APD 1 Gate Relative Phase"=→"APD 1 Gate Relative Phase":i16, "APD 2 Gate Relative Phase"=→"APD 2 Gate Relative Phase":i16, "APD Acq Late Counter"=→"APD Acq Late Counter":u16, "APD 1 Gate Late Counter"=→"APD 1 Gate Late Counter":u8, "APD 2 Gate Late Counter"=→"APD 2 Gate Late Counter":u8, "Green FB Relative Phase"=→"Relative phase (Green FB)":i16, "GI Relative phase"=→"GI relative phase 2":i16, "GI Late Counter 2"=→"GI Late Counter 2":u16, "Trap Pos FIFO Timeout"=→"Trap Pos FIFO Timeout":u16, "Trap AI FIFO Timeout"=→"Trap AI FIFO Timeout":u16)
      }
    }
    n1318 = xnode ("Read/Write Control")("FPGA VI Reference In"=w1717, "error in"=w1716) -> ("FPGA VI Reference Out"=w1782:T18, "error out"=w1776:errorcluster, "AI2 Y Sum Set 1"=w1772:i16, "AI2 Y Sum Set 2"=w1771:i16, "AI1 X Set 1"=w1690:fxp<+/-,16,1>, "AI1 X Set 2"=w1689:fxp<+/-,16,1>, "Trap Pos FB Int Signal"=→"Trap Pos FB Int Signal":fxp<+/-,24,9>, "Trap Pos FB Int-Norm Signal"=→"Trap Pos FB Int-Norm Signal":fxp<+/-,16,1>, "Trap Pos FB Action"=→"Trap Pos FB Action":i64, "Scanning"=→"AOD Scanning":bool, "Scan I"=→"AOD Scan I":u64, "Scanning MCL"=w1774:bool, "Scan I (MCL)"=→"MCL Scan I":u64, "Green FB Signals"=w1733:T32, "BD1 amplitude 1 out"=w1611:u16, "BD1 amplitude 2 out"=w1613:u16)  [unwired: 1 out]
    "MCL Scanning" <- w1774
    n1319 = local read "Data points/scans (MCL)"() -> (w1627:dbl)
    n1320 = Decimate 1D Array(w1586) -> (w1711:u32[], w1628:u32[])
    n1321 = local read "DMA Update Period (s)"() -> (w1714:dbl)
    n1322 = To Double Precision Float(number=w1711) -> (double precision float=w1602:dbl[])
    n1323 = To Double Precision Float(number=w1628) -> (double precision float=w1625:dbl[])
    n1324 = disable-structure shown="Disabled" {
      frame Disabled {
        n1325 = local read "BD 1 Frq 1 (MHz)"() -> ()  [unwired: 1 out]
        n1326 = local read "BD 1 Frq 2 (MHz)"() -> ()  [unwired: 1 out]
      }
      frame Enabled {
      }
    }
    n1327 = Array Size(array=w1625) -> (size(s)=w1749:i32)
    n1328 = call "Ampint162Dbl.vi"("In i16"=w1611) -> ("Amp (%)"=w1610:dbl)  [unwired: 4 in]
    "Trap 1 amp." <- w1610
    n1329 = call "Ampint162Dbl.vi"("In i16"=w1613) -> ("Amp (%)"=w1612:dbl)  [unwired: 4 in]
    "Trap 2 amp." <- w1612
    n1330 = Build Array(w1602, w1625) -> (w1626:dbl[][])
    n1331 = local read "APD Integration Time (s)"() -> (w1649:dbl)
    n1332 = local read "MCL Scanning"() -> (w1741:bool)
    n1333 = Increment(x=w1627) -> (x+1=w1747:dbl)
    n1334 = local read "Data Period (s)"() -> (w1573:dbl)
    n1335 = local read "AI2 (V)"() -> (w1773:cluster{"Set 1":dbl, "Set 2":dbl})
    n1336 = Bundle By Name(cluster=w1773, "Set 1"=w1772, "Set 2"=w1771) -> (w1769:cluster{"Set 1":dbl, "Set 2":dbl})
    n1337 = feedback #8(w1747) -> (w1750:dbl)
    n1338 = Select(t=0, s=w1738, f=w1750) -> (s? t:f=w1744:dbl)
    n1339 = Add(x=w1749, y=w1744) -> (x+y=w1745:dbl)
    n1340 = Greater?(x=w1745, y=w1627) -> (0:w1746:bool)
    n1341 = feedback #9(0.0) -> (w1695:dbl)
    n1342 = Add(x=w1714, y=w1695) -> (x+y=w1765:dbl)
    n1343 = feedback-in #9(w1765) -> ()
    n1344 = Select(t=w1744, s=w1746, f=w1745) -> (s? t:f=w1743:dbl)
    n1345 = feedback-in #8(w1743) -> ()
    n1346 = Not(x=w1746) -> (.not. x?=w1740:bool)
    n1347 = To Time Stamp(1:w1695) -> (0:w1643:timestamp)
    n1348 = Build Array(w1597, w1597) -> (w1645:dbl[])
    n1349 = And(x=w1740, y=w1741) -> (x .and. y?=w1742:bool)
    n1350 = Or(x=w1742, y=w1738) -> (x .or. y?=w1739:bool)
    n1351 = Divide(x=w1769, y=3276.7) -> (x/y=w1768:cluster{"Set 1":dbl, "Set 2":dbl})
    n1352 = Multiply(x=w1573, y="Trap Disp. Downsample") -> (x*y=w1641:dbl)
    "Display Period (s)" <- w1641
    n1353 = call "TPosDSamp.vi"("TPos Data"=w1644, "Data Period (s)"=w1573, "TPos Disp. Dsamp"="Trap Disp. Downsample", "Time Stamp"=w1643, "Trap Pos"=w1645) -> ("TPos dSampd"=w1618:waveform(dbl)[])  [unwired: 14 in]
    n1354 = Multiply(x=w1649, y="APD Disp. dSamp") -> (x*y=w1596:dbl)
    "APD Display Period (s)" <- w1596
    n1355 = call "APDDSamp.vi"("APD Data"=w1626, "Data Period (s)"=w1649, "APD Disp. dSamp"="APD Disp. dSamp", "Time Stamp"=w1643) -> ("APD dSampd"=w1603:waveform(dbl)[])  [unwired: 15 in]
    n1356 = call "TrapDSamp.vi"("Trap Data"=w1650, "Data Period (s)"=w1573, "Trap Disp. dSamp"="Trap Disp. Downsample", "Time Stamp"=w1643, "Channel Names"=w1630) -> ("Trap dSampd"=w1652:waveform(dbl)[], "Trap Raw"=w1651:waveform(dbl)[])  [unwired: 13 in]
    n1357 = Equal?(x="Tab Control Display", y=T29."FFT") -> (x = y?=w1631:bool)
    n1358 = local read "FFB AvgX"() -> (w1694:T10)
    n1359 = local read "All FB On/Off"() -> (w1666:bool)
    n1360 = local write "AI2 (V)"(w1768) -> ()
    n1361 = Reciprocal(x=w1641) -> (1/x=→"Trap Disp. Freq. (Hz)":dbl)
    n1362 = case "Update MCL Scan Images" shown="True" w1739 {
      tunnel: w1738 -> [_ w1934]
      tunnel: w1602 -> [_ w1950]
      tunnel: w1651 -> [_ w1952]
      tunnel: w1625 -> [_ w1946]
      tunnel: w1700 -> [_ w1951]
      frame False {
      }
      frame True {
        n1363 = local read "Cycles/step (MCL)"() -> (w1935:u64)
        n1364 = local read "N APD Samp/step"() -> (w1947:i32)
        n1365 = Index Array(array=w1952, index=10) -> (element=w1955:waveform(dbl))
        n1366 = local read "Scan steps (x)"() -> (w1937:u64)
        n1367 = Index Array(array=w1952, index=11) -> (element=w1953:waveform(dbl))
        n1368 = local read "Scan lines (y)"() -> (w1936:u64)
        n1369 = Unbundle By Name(w1955) -> ("Y"=w1938:dbl[])
        n1370 = Unbundle By Name(w1953) -> ("Y"=w1939:dbl[])
        n1371 = Unbundle(w1951) -> ("New Image"=w1949:T2, "New Image"=w1945:T2, "New Image"=w1943:T2, "New Image"=w1940:T2)
        n1372 = call "MCLScanAPD.vi"("Image In"=w1949, "APD Cts"=w1950, "Scan steps (MCL)"=w1937, "Scan lines (y)"=w1936, "N APD Samp/step"=w1947, "NewScan?"=w1934) -> ("Image Out"=→"APD 1":T2)  [unwired: 13 in]
        n1373 = call "MCLScanAPD.vi"("Image In"=w1945, "APD Cts"=w1946, "Scan steps (MCL)"=w1937, "Scan lines (y)"=w1936, "N APD Samp/step"=w1947, "NewScan?"=w1934) -> ("Image Out"=→"APD 2":T2)  [unwired: 13 in]
        n1374 = call "MCLScanPSD.vi"("In Image"=w1940, "Trap Detector"=w1938, "Scan steps (x)"=w1937, "Scan lines (y)"=w1936, "Cycles/step (MCL)"=w1935, "NewScan?"=w1934) -> ("Out Image"=→"Detection Laser Y":T2)  [unwired: 13 in]
        n1375 = call "MCLScanPSD.vi"("In Image"=w1943, "Trap Detector"=w1939, "Scan steps (x)"=w1937, "Scan lines (y)"=w1936, "Cycles/step (MCL)"=w1935, "NewScan?"=w1934) -> ("Out Image"=→"Detection Laser X":T2)  [unwired: 13 in]
      }
    }
    n1376 = case "Display FFT" shown="True" w1631 {
      tunnel: w1651 -> [_ w2121]
      frame False {
      }
      frame True {
        n1377 = Array Size(array=w2121) -> (size(s)=w2120:i32)
        n1378 = feedback-in #10("# Spectra to Ave.") -> ()
        n1379 = feedback #10("# Spectra to Ave.") -> (w2112:dbl)
        n1380 = Build Array("FFT 1 Choice 1", "FFT 1 Choice 2", "FFT 2 Choice 1", "FFT 2 Choice 2") -> (w2114:u16[])
        n1381 = Not Equal?(x="# Spectra to Ave.", y=w2112) -> (x != y?=w2111:bool)
        n1382 = feedback-in #11(w2114) -> ()
        n1383 = feedback #11(u16[] [100, 100, 100, 100]) -> (w2115:u16[])
        n1384 = Not Equal?(x=w2114, y=w2115) -> (x != y?=w2113:bool)
        n1385 = Compound Arithmetic op=OR("Reset FFT", w2113, w2111) -> (w2096:bool)
        n1386 = feedback #12(1.0) -> (w2098:dbl)
        n1387 = Select(t=1.0, s=w2096, f=w2098) -> (s? t:f=w2100:dbl)
        n1388 = Greater?(x=w2100, y="# Spectra to Ave.") -> (0:w2119:bool)
        n1389 = Increment(x=w2100) -> (x+1=w2099:dbl)
        n1390 = feedback-in #12(w2099) -> ()
        n1391 = local read "DMA Update Period (s)"() -> (w2094:dbl)
        n1392 = Multiply(x="# Spectra to Ave.", y=w2094) -> (x*y=→"Ave. Time (s)":dbl)
        n1393 = Build Array(cluster{"f0":dbl, "df":dbl, "magnitude":dbl[]} {"f0"=0.0, "df"=0.0, "magnitude"=[]} ("PSD")) -> (w2103:cluster{"f0":dbl, "df":dbl, "magnitude":dbl[]}[])
        n1394 = Build Array(w2103, w2103, w2103, w2103) -> (w2105:T33)
        n1395 = feedback #13(w2105) -> (w2110:T33)
        n1396 = for {
          N: 4 -> [_]
          tunnel: w2114 -> [w2143] mode=indexing
          tunnel: w2121 -> [w2144]
          tunnel: w2120 -> [w2146]
          tunnel: w2096 -> [w2139]
          tunnel: w2119 -> [w2138]
          tunnel: "# Spectra to Ave." -> [w2137]
          tunnel: [w2136] -> w2109 mode=indexing
          tunnel: w2110 -> [w2141] mode=indexing
          tunnel: [w2140] -> w2097 mode=indexing
          tunnel: w2100 -> [w2135]
          n1397 = Less?(x=w2143, y=w2146) -> (x < y?=w2145:bool)
          n1398 = Index Array(array=w2144, index=w2143) -> (element=w2142:waveform(dbl))
          n1399 = case shown="True" w2145 {
            tunnel: w2142 -> [_ w2163]
            tunnel: w2141 -> [w2148 w2161]
            tunnel: [w2148 w2149] -> w2140
            tunnel: w2139 -> [_ w2160]
            tunnel: w2138 -> [_ w2153]
            tunnel: w2137 -> [_ w2152]
            tunnel: [cluster{"f0":dbl, "df":dbl, "magnitude":dbl[]} {"f0"=0.0, "df"=0.0, "magnitude"=[]} ("PSD") w2154] -> w2136
            tunnel: w2135 -> [_ w2151]
            frame False {
            }
            frame True {
              n1400 = call-poly <vilib>:"Mean.vi"("X"=w2163) -> ("mean"=w2164:dbl)  [unwired: 1 out]
              n1401 = Subtract(x=w2163, y=w2164) -> (x-y=w2162:waveform(dbl))
              n1402 = xnode ("Spectral Measurements")("Signals"=w2162) -> ("PSD"=w2156:cluster{"f0":dbl, "df":dbl, "magnitude":dbl[]})  [unwired: 1 in, 1 out]
              n1403 = case shown="False" w2160 {
                tunnel: w2161 -> [w2173 _]
                tunnel: [w2169 w2178] -> w2149
                tunnel: w2156 -> [w2172 w2179]
                tunnel: w2153 -> [w2171 _]
                frame False {
                  n1404 = Build Array (concatenate)(w2173, w2172) -> (w2170:cluster{"f0":dbl, "df":dbl, "magnitude":dbl[]}[])
                  n1405 = case shown="True" w2171 {
                    tunnel: w2170 -> [w2174 w2177]
                    tunnel: [w2174 w2175] -> w2169
                    frame False {
                    }
                    frame True {
                      n1406 = Delete From Array(array=w2177, index=0) -> (array with subset deleted=w2175:cluster{"f0":dbl, "df":dbl, "magnitude":dbl[]}[])  [unwired: 1 in, 1 out]
                    }
                  }
                }
                frame True {
                  n1407 = Build Array(w2179) -> (w2178:cluster{"f0":dbl, "df":dbl, "magnitude":dbl[]}[])
                }
              }
              n1408 = for {
                tunnel: w2149 -> [w2168] mode=indexing
                tunnel: [w2167] -> w2159 mode=indexing
                workers-P: _ -> [_]
                n1409 = Unbundle By Name(w2168) -> ("magnitude"=w2167:dbl[])
              }
              n1410 = Transpose 2D Array(2D array=w2159) -> (transposed array=w2158:dbl[][])
              n1411 = for {
                tunnel: w2158 -> [w2166] mode=indexing
                tunnel: [w2165] -> w2157 mode=indexing
                workers-P: _ -> [_]
                n1412 = Add Array Elements(numeric array=w2166) -> (sum=w2165:dbl)
              }
              n1413 = Select(t=w2152, s=w2153, f=w2151) -> (s? t:f=w2150:dbl)
              n1414 = Divide(x=w2157, y=w2150) -> (x/y=w2155:dbl[])
              n1415 = Bundle By Name(cluster=w2156, "magnitude"=w2155) -> (w2154:cluster{"f0":dbl, "df":dbl, "magnitude":dbl[]})
            }
          }
        }
        n1416 = case shown="True" w2096 {
          tunnel: w2097 -> [w2128 w2134]
          tunnel: [w2128 w2129] -> w2095
          frame False {
          }
          frame True {
            n1417 = Array Subset(array=w2134, index (row)=0 ("index"), length (row)=4 ("length"), index (col)=0 ("index"), length (col)=1 ("length")) -> (w2129:T33)
          }
        }
        n1418 = feedback-in #13(w2095) -> ()
        n1419 = Split 1D Array(array=w2109, index=2) -> (first subarray=→"FFT 1":cluster{"f0":dbl, "df":dbl, "magnitude":dbl[]}[], second subarray=→"FFT 2":cluster{"f0":dbl, "df":dbl, "magnitude":dbl[]}[])
      }
    }
    n1420 = Reciprocal(x=w1596) -> (1/x=→"APD Display Freq. (Hz)":dbl)
    n1421 = Bundle(cluster=w1694, "Trap 1"=w1690, "Trap 2"=w1689) -> (→"FFB AvgX":T10)
    n1422 = Divide(x=w1733, y=3276.7) -> (x/y=w1730:T34)
    n1423 = case "Turn off TPowFB if over 50%" shown="True" w1666 {
      tunnel: w1610 -> [_ w1845]
      tunnel: w1612 -> [_ w1844]
      frame False {
      }
      frame True {
        w1846 = ext 50.0
        n1424 = Greater?(x=w1845, y=w1846) -> (0:w1843:bool)
        n1425 = Greater?(x=w1844, y=w1846) -> (0:w1842:bool)
        n1426 = Or(x=w1843, y=w1842) -> (x .or. y?=w1841:bool)
        n1427 = case shown="True" w1841 {
          frame False {
          }
          frame True {
            n1428 = property on="All FB On/Off" class="Bool (strict)"("Val(Sgnl)"=FALSE) -> ()  [unwired: 2 in, 2 out]
            n1429 = local write "Feedback \noverload"(TRUE) -> ()
          }
        }
      }
    }
    n1430 = Unbundle By Name(w1730) -> ("Green FB Ch 0"=w1732:dbl, "Green FB Ch 1"=w1731:dbl, "Green FB Ch 2"=w1569:dbl)
    "PD Sum" <- w1569
    n1431 = Multiply(x=w1603, y="APD Disp. Scale") -> (x*y=w1647:waveform(dbl)[])
    n1432 = Build Array (concatenate)(w1647, w1652) -> (w1709:waveform(dbl)[])
    "All Signals" <- w1709
    n1433 = case "Get Offset" shown="True" "Use Full Offset?" {
      tunnel: ["T1 offX (V)" w1852] -> w1634
      tunnel: ["T2 offX (V)" w1851] -> w1637
      tunnel: w1670 -> [_ w1858]
      frame False {
      }
      frame True {
        n1434 = local read "Offset file step size"() -> (w1857:dbl)
        n1435 = local read "Offset Values"() -> (w1859:T14)
        n1436 = Unbundle By Name(w1859) -> ("Trap 1X offset"=w1854:dbl[], "Trap 2X offset"=w1853:dbl[])
        n1437 = Divide(x=w1858, y=w1857) -> (x/y=w1856:dbl)
        n1438 = To Long Integer(number=w1856) -> (32bit integer=w1855:i32)
        n1439 = Index Array(array=w1854, index=w1855) -> (element=w1852:dbl)
        n1440 = Index Array(array=w1853, index=w1855) -> (element=w1851:dbl)
      }
    }
    n1441 = Divide(x=w1603, y=w1596) -> (x/y=w1699:waveform(dbl)[])
    n1442 = Divide(x=w1732, y=w1569) -> (x/y=w1729:dbl)
    n1443 = Divide(x=w1731, y=w1569) -> (x/y=w1728:dbl)
    n1444 = Index Array(array=w1699, index=0) -> (element=w1706:waveform(dbl))
    n1445 = Index Array(array=w1699, index=1) -> (element=w1704:waveform(dbl))
    n1446 = Bundle By Name(cluster=w1730, "Green FB Ch 0"=w1729, "Green FB Ch 1"=w1728) -> (→"Green FB Signals (V)":T34)
    n1447 = Subtract(x=w1704, y="APD 2 Offset") -> (x-y=w1601:waveform(dbl))
    n1448 = Subtract(x=w1706, y="APD 1 Offset") -> (x-y=w1702:waveform(dbl))
    n1449 = Index Array(array=w1709, index=3) -> (element=w1600:waveform(dbl))
    n1450 = Index Array(array=w1709, index=6) -> (element=w1640:waveform(dbl))
    n1451 = Build Array(w1702, w1601) -> (→"APD Chart":waveform(dbl)[])
    n1452 = local read "Fish Status"() -> (w1664:u16)
    n1453 = local read "Reset MCL after scan"() -> (w1777:bool)
    n1454 = local read "AOM X Cal (nm/MHz)"() -> (w1619:dbl)
    n1455 = Not(x=w1774) -> (.not. x?=w1778:bool)
    n1456 = feedback-in #14("Calibration") -> ()
    n1457 = feedback #14(u16 1 ("Calibration")) -> (w1724:u16)
    n1458 = Add(x="Trap 2 Bead Size (nm)", y="Trap 1 Bead Size (nm)") -> (x+y=w1680:dbl)
    n1459 = call "CalcForce.vi"("Trap 1X V"=w1600, "T1 alphaX (nm/V)"="T1 alX (nm/V)", "T1 kappaX (pN/nm)"="T1 kaX (pN/nm)", "T1 offset X"=w1634, "Trap 2X V"=w1640, "Calibration"="Calibration", "T2 alphaX (nm/V)"="T2 alX (nm/V)", "T2 kappaX (pN/nm)"="T2 kaX (pN/nm)", "T2 offsetX"=w1637) -> ("Force 1X"=w1615:waveform(dbl), "Force X"=w1617:waveform(dbl), "Force 2X"=w1614:waveform(dbl), "BeadDeflection"=w1623:waveform(dbl), "Out Names"=w1632:T35)  [unwired: 2 in]
    n1460 = And(x=w1778, y=w1777) -> (x .and. y?=w1779:bool)
    n1461 = Not Equal?(x=w1724, y="Calibration") -> (x != y?=w1712:bool)
    n1462 = Divide(x=w1680, y=2.0) -> (x/y=w1622:dbl)
    n1463 = Add(x=w1622, y="Ext Offset (nm)") -> (x+y=w1620:dbl)
    n1464 = case "Update Graph Labels" shown="True" w1712 {
      tunnel: w1632 -> [_ w1933]
      frame False {
      }
      frame True {
        n1465 = Unbundle(w1933) -> ("Label.Text"=w1928:string, "Label.Text"=w1932:string, "Label.Text"=w1931:string, "Label.Text"=w1930:string, "Label.Text"=w1929:string)
        n1466 = property on="T1 X" class="DigNum (strict)"("Caption.Text"=w1928) -> ()  [unwired: 2 in, 2 out]
        n1467 = property on="T2 X" class="DigNum (strict)"("Caption.Text"=w1932) -> ()  [unwired: 2 in, 2 out]
        n1468 = property on="Force" class="WFChart (strict)"("YScale.NameLbl.Text"=w1931) -> ()  [unwired: 2 in, 2 out]
        n1469 = property on="Difference" class="DigNum (strict)"("Caption.Text"=w1930) -> ()  [unwired: 2 in, 2 out]
        n1470 = property on="Mean" class="DigNum (strict)"("Caption.Text"=w1929) -> ()  [unwired: 2 in, 2 out]
      }
    }
    n1471 = case "Return MCL after MCL Raster" shown="True" w1779 {
      tunnel: w1782 -> [w2024 w2035]
      tunnel: [w2024 w2034] -> w1781
      tunnel: w1776 -> [w2023 w2033]
      tunnel: [w2023 w2032] -> w1775
      frame False {
      }
      frame True {
        n1472 = local read "Total Counts (ticks)"() -> (w2029:u32)
        n1473 = local read "MCL Y"() -> (w2028:dbl)
        n1474 = local read "MCL X"() -> (w2027:dbl)
        n1475 = local read "Scan Range (V)"() -> (w2030:dbl)
        n1476 = local write "Reset MCL after scan"(FALSE ("wait to reset values")) -> ()
        n1477 = call "V2int16.vi"("InV"=w2028) -> ("Out i16"=w2025:i16)  [unwired: 4 in]
        n1478 = call "V2int16.vi"("InV"=w2027) -> ("Out i16"=w2026:i16)  [unwired: 4 in]
        n1479 = xnode "Read/Write Control"("FPGA VI Reference In"=w2035, "error in"=w2033, "AO1 (Y)"=w2025, "AO2 (X)"=w2026, "MCL count"=w2029) -> ("FPGA VI Reference Out"=w2034:T18, "error out"=w2032:errorcluster)
        n1480 = property on="Scan Range (V)" class="DigNum (strict)"("Val(Sgnl)"=w2030) -> ()  [unwired: 2 in, 2 out]
      }
    }
    n1481 = call "CalcExtension.vi"("Offset"=w1620, "AOM X Cal"=w1619, "Trap Positions"=w1618, "BeadDeflection"=w1623) -> ("Extension"=w1616:waveform(dbl))  [unwired: 7 in]
    "Extension" <- w1616
    n1482 = Build Array(w1615, w1614, w1617) -> (→"Force":waveform(dbl)[])
    n1483 = Unbundle By Name(w1617) -> ("Y"=w1607:dbl[])
    n1484 = Unbundle By Name(w1616) -> ("Y"=w1608:dbl[])
    n1485 = call-poly <vilib>:"Mean.vi"("X"=w1607) -> ("mean"=w1598:dbl)  [unwired: 1 out]
    n1486 = call-poly <vilib>:"Mean.vi"("X"=w1608) -> ("mean"=w1599:dbl)  [unwired: 1 out]
    n1487 = Bundle("mean"=w1599, "mean"=w1598) -> (w1605:cluster{"mean":dbl, "mean":dbl})  [unwired: 1 in]
    n1488 = call "XY Chart Buffer V5.vi"("Clear History? (default: no)"="Clear FX", "History Length (default:1000)"=100, "New Point"=w1605) -> ("XY Chart Data"=→"Force-Extension":cluster{"x":dbl, "y":dbl}[])  [unwired: 8 in]
    n1489 = call-poly <vilib>:"Mean.vi"("X"=w1615) -> ("mean"=w1668:dbl)  [unwired: 1 out]
    "T1 X" <- w1668
    n1490 = call-poly <vilib>:"Mean.vi"("X"=w1614) -> ("mean"=w1667:dbl)  [unwired: 1 out]
    "T2 X" <- w1667
    n1491 = Add(x=w1668, y=w1667) -> (x+y=w1723:dbl)
    n1492 = Add(x=w1668, y=w1667) -> (x+y=→"Difference":dbl)
    n1493 = Divide(x=w1723, y=2.0) -> (x/y=w1665:dbl)
    "Mean" <- w1665
    n1494 = case "Autofishing" shown="False" "Toggle AFish" {
      tunnel: w1665 -> [w1794 _]
      tunnel: w1664 -> [w1793 w1837]
      frame False {
        n1495 = case "Autofishing - Alex" shown="3" w1793 {
          tunnel: w1794 -> [_ _ _ w1823 _]
          frame 0, Default {
            # "Off"
          }
          frame 1 {
            # "Approach"
            n1496 = local read "Trap Delta (MHz)"() -> (w1797:dbl)
            n1497 = Add(x=w1797, y="Approach dTD") -> (x+y=w1796:dbl)
            n1498 = In Range and Coerce(upper limit=inf, x=w1796, lower limit="Min TD") -> (coerced(x)=w1798:dbl, In Range?=w1799:bool)
            n1499 = case shown="False" w1799 {
              frame False {
                w1803 = u16 2 items=["Off", "Approach", "Wiggle", "Extend", "Tether Found"] ("Fish Status")
                n1500 = Tick Count (ms)() -> (millisecond timer value=→"AF Time":u32)
                n1501 = local write "Fish Status"(w1803) -> ()
              }
              frame True {
              }
            }
            n1502 = property on="Trap Delta (MHz)" class="Slide (strict)"("Val(Sgnl)"=w1798) -> ()  [unwired: 2 in, 2 out]
          }
          frame 2 {
            # "Wiggle"
            n1503 = local read "AF Time"() -> (w1814:u32)
            n1504 = Random Number (0-1)() -> (number: 0 to 1=w1809:dbl)
            n1505 = Tick Count (ms)() -> (millisecond timer value=w1815:u32)
            n1506 = local read "Min TD"() -> (w1806:dbl)
            n1507 = Subtract(x=w1815, y=w1814) -> (x-y=w1813:u32)
            n1508 = Multiply(x=w1809, y="Wiggle TD") -> (x*y=w1807:dbl)
            n1509 = Divide(x=w1813, y=u32 1000) -> (x/y=w1811:dbl)
            n1510 = Add(x=w1807, y=w1806) -> (x+y=w1804:dbl)
            n1511 = Greater?(x=w1811, y="Wiggle time") -> (0:w1805:bool)
            n1512 = property on="Trap Delta (MHz)" class="Slide (strict)"("Val(Sgnl)"=w1804) -> ()  [unwired: 2 in, 2 out]
            n1513 = case shown="True" w1805 {
              frame False {
              }
              frame True {
                w1816 = u16 3 items=["Off", "Approach", "Wiggle", "Extend", "Tether Found"] ("Fish Status")
                n1514 = local write "Fish Status"(w1816) -> ()
              }
            }
          }
          frame 3 {
            # "Extend"
            n1515 = local read "Trap Delta (MHz)"() -> (w1829:dbl)
            n1516 = Add(x=w1829, y="Extend dTD") -> (x+y=w1827:dbl)
            n1517 = In Range and Coerce(upper limit="Max TD", x=w1827, lower limit=0.0) -> (coerced(x)=w1818:dbl, In Range?=w1817:bool)
            n1518 = Greater?(x=w1818, y="Extend Min TD") -> (0:w1821:bool)
            n1519 = Greater?(x=w1823, y="Extend Min F") -> (0:w1822:bool)
            n1520 = property on="Trap Delta (MHz)" class="Slide (strict)"("Val(Sgnl)"=w1818) -> ()  [unwired: 2 in, 2 out]
            n1521 = And(x=w1821, y=w1822) -> (x .and. y?=w1820:bool)
            n1522 = case shown="False" w1820 {
              tunnel: w1817 -> [w1830 _]
              frame False {
                n1523 = case shown="False" w1830 {
                  frame False {
                    w1831 = u16 1 items=["Off", "Approach", "Wiggle", "Extend", "Tether Found"] ("Fish Status")
                    n1524 = local write "Fish Status"(w1831) -> ()
                  }
                  frame True {
                  }
                }
              }
              frame True {
                w1832 = u16 4 items=["Off", "Approach", "Wiggle", "Extend", "Tether Found"] ("Fish Status")
                n1525 = local write "Fish Status"(w1832) -> ()
              }
            }
          }
          frame 4 {
            w1833 = u16 0 items=["Off", "Approach", "Wiggle", "Extend", "Tether Found"] ("Fish Status")
            n1526 = local write "Fish Status"(w1833) -> ()
            n1527 = call <vilib>:"Beep.vi"("use system alert? (T)"=FALSE, "duration (msec)"=u32 100, "frequency (Hz)"=u32 466) -> ()  [unwired: 9 in]
          }
        }
      }
      frame True {
        n1528 = case shown="0" w1837 {
          frame 0 {
            w1839 = u16 1 items=["Off", "Approach", "Wiggle", "Extend", "Tether Found"] ("Fish Status")
            n1529 = local write "Fish Status"(w1839) -> ()
          }
          frame Default {
            w1840 = u16 0 items=["Off", "Approach", "Wiggle", "Extend", "Tether Found"] ("Fish Status")
            n1530 = local write "Fish Status"(w1840) -> ()
          }
        }
        n1531 = local write "Toggle AFish"(FALSE ("Toggle AFish")) -> ()
      }
    }
  }
  n1532 = timed-loop "Handle Mouse Events (Confocal spot, Trap Motion)" {
    tunnel: [w2461] -> w50
    tunnel: w46 -> [_]
    timing: w83 -> [_]
    timing-out: [_] -> w82
    tunnel: w1 -> [w2460]
    stop <- w2461 stop-if-true
    n1533 = event shown="[1] \"Pane\": Mouse Down" {
      selector: _ -> [_ _]
      dyn-events: _ -> [_ _]
      timeout: 10 -> [_ _]
      tunnel: w2460 -> [w2463 w2477]
      event Timeout {
        n1534 = event-data() -> ()  [unwired: 4 out]
        n1535 = local read "MouseMove Trap"() -> (w2462:bool)
        n1536 = case shown="True" w2462 {
          tunnel: w2463 -> [_ w2476]
          frame False {
          }
          frame True {
            n1537 = call-poly <vilib>:"Acquire Input Data.vi"("device ID"=w2476) -> ("axis info"=w2475:T36)  [unwired: 15 in, 3 out]
            n1538 = local read "Trap Delta (MHz)"() -> (w2472:dbl)
            n1539 = Unbundle By Name(w2475) -> ("Horizontal"=w2466:i32)
            n1540 = local read "MouseX"() -> (w2474:i32)
            n1541 = Unbundle By Name("MouseMove Speed") -> ("Horizontal"=w2469:dbl)
            n1542 = local write "MouseX"(w2466) -> ()
            n1543 = Subtract(x=w2466, y=w2474) -> (x-y=w2473:i32)
            n1544 = Multiply(x=w2473, y=w2469) -> (x*y=w2471:dbl)
            n1545 = property on="Trap Delta (MHz)" class="Slide (strict)"() -> ("Maximum"=w2465:dbl, "Minimum"=w2464:dbl)  [unwired: 2 in, 2 out]
            n1546 = Add(x=w2472, y=w2471) -> (x+y=w2468:dbl)
            n1547 = In Range and Coerce(upper limit=w2465, x=w2468, lower limit=w2464) -> (coerced(x)=w2467:dbl)  [unwired: 1 out]
            n1548 = property on="Trap Delta (MHz)" class="Slide (strict)"("Val(Sgnl)"=w2467) -> ()  [unwired: 2 in, 2 out]
          }
        }
      }
      event Mouse Down {
        n1549 = event-data() -> ("Time"=w2478:u32, "Coords"=w2479:T37, "Button"=w2480:u16)  [unwired: 1 out]
        n1550 = case shown="1" w2480 {
          tunnel: w2478 -> [_ _ _]
          tunnel: w2479 -> [_ w2515 _]
          tunnel: w2477 -> [_ _ w2558]
          frame 0, Default {
          }
          frame 1 {
            n1551 = property on="Detection Laser X" class="ImageControl"() -> ("Displayed Image Position"=w2513:cluster{"Left":i32, "Top":i32}, "Displayed Image Size"=w2488:cluster{"Width":u32, "Height":u32})  [unwired: 2 in, 2 out]
            n1552 = property on="Detection Laser Y" class="ImageControl"() -> ("Displayed Image Position"=w2512:cluster{"Left":i32, "Top":i32}, "Displayed Image Size"=w2487:cluster{"Width":u32, "Height":u32})  [unwired: 2 in, 2 out]
            n1553 = property on="APD 2" class="ImageControl"() -> ("Displayed Image Position"=w2495:cluster{"Left":i32, "Top":i32}, "Displayed Image Size"=w2490:cluster{"Width":u32, "Height":u32})  [unwired: 2 in, 2 out]
            n1554 = property on="APD 1" class="ImageControl"() -> ("Displayed Image Position"=w2514:cluster{"Left":i32, "Top":i32}, "Displayed Image Size"=w2489:cluster{"Width":u32, "Height":u32})  [unwired: 2 in, 2 out]
            n1555 = Unbundle By Name(w2490) -> ("Width"=w2492:u32, "Height"=w2491:u32)
            n1556 = Unbundle By Name(w2489) -> ("Width"=w2509:u32, "Height"=w2508:u32)
            n1557 = Unbundle By Name(w2488) -> ("Width"=w2505:u32, "Height"=w2504:u32)
            n1558 = Unbundle By Name(w2487) -> ("Width"=w2501:u32, "Height"=w2500:u32)
            n1559 = Unbundle By Name(w2495) -> ("Left"=w2494:i32, "Top"=w2493:i32)
            n1560 = Unbundle By Name(w2514) -> ("Left"=w2511:i32, "Top"=w2510:i32)
            n1561 = Unbundle By Name(w2513) -> ("Left"=w2507:i32, "Top"=w2506:i32)
            n1562 = Unbundle By Name(w2512) -> ("Left"=w2503:i32, "Top"=w2502:i32)
            n1563 = Bundle("Left"=w2494, "Top"=w2493, "Width"=w2492, "Height"=w2491) -> (w2485:T38)  [unwired: 1 in]
            n1564 = Bundle("Left"=w2511, "Top"=w2510, "Width"=w2509, "Height"=w2508) -> (w2484:T38)  [unwired: 1 in]
            n1565 = Bundle("Left"=w2507, "Top"=w2506, "Width"=w2505, "Height"=w2504) -> (w2483:T38)  [unwired: 1 in]
            n1566 = Bundle("Left"=w2503, "Top"=w2502, "Width"=w2501, "Height"=w2500) -> (w2482:T38)  [unwired: 1 in]
            n1567 = Build Array(w2485, w2484, w2483, w2482) -> (w2481:T39)
            n1568 = for "Check if the click is \nwithin any image..." {
              tunnel: w2515 -> [w2522]
              tunnel: w2481 -> [w2516] mode=indexing
              tunnel: [w2517] -> w2486
              tunnel: [w2521] -> w2499
              tunnel: [w2520] -> w2498
              tunnel: [w2519] -> w2497
              tunnel: [w2518] -> w2496
              stop <- w2517 stop-if-true
              n1569 = call "isclickinwindow.vi"("Image Param"=w2516, "Point32"=w2522) -> ("Y px"=w2518:i32, "Height"=w2519:i32, "X px"=w2520:i32, "Width"=w2521:i32, "In image?"=w2517:bool)  [unwired: 1 in]
            }
            n1570 = case "If so, update Confocal X/Y" shown="True" w2486 {
              tunnel: w2498 -> [_ w2535]
              tunnel: w2496 -> [_ w2534]
              tunnel: w2499 -> [_ w2533]
              tunnel: w2497 -> [_ w2532]
              frame False {
              }
              frame True {
                w2528 = FALSE ("Get Point")
                n1571 = local read "Actual MCL Inc (V)"() -> (w2529:dbl)
                n1572 = local read "Scan steps (x)"() -> (w2536:u64)
                n1573 = local read "Scan lines (y)"() -> (w2537:u64)
                n1574 = Divide "Y Pix/step"(x=w2532, y=w2537) -> (x/y=w2544:dbl)
                n1575 = Divide "X px/step"(x=w2533, y=w2536) -> (x/y=w2542:dbl)
                n1576 = Divide "Y V/pix"(x=w2529, y=w2544) -> (x/y=w2543:dbl)
                n1577 = local write "Set X Only"(w2528) -> ()
                n1578 = local write "Set Y Only"(w2528) -> ()
                n1579 = Divide "Y half step offset"(x=w2529, y=2.0) -> (x/y=w2545:dbl)
                n1580 = local write "Set Confocal Spot"(w2528) -> ()
                n1581 = Divide "X V/px"(x=w2529, y=w2542) -> (x/y=w2541:dbl)
                n1582 = Multiply(x=w2529, y=w2536) -> (x*y=w2548:dbl)
                n1583 = Negate(x=w2545) -> (-x=w2546:dbl)
                n1584 = local read "Initial Y"() -> (w2552:dbl)
                n1585 = Divide "X half step offset"(x=w2529, y=2.0) -> (x/y=w2539:dbl)
                n1586 = Multiply(x=w2534, y=w2543) -> (x*y=w2553:dbl)
                n1587 = Multiply(x=w2541, y=w2535) -> (x*y=w2550:dbl)
                n1588 = Negate(x=w2539) -> (-x=w2538:dbl)
                n1589 = local read "Initial X"() -> (w2551:dbl)
                n1590 = Compound Arithmetic op=ADD(w2546, w2553, w2552) -> (w2530:dbl)
                "Pointer Y (V)" <- w2530
                n1591 = Negate(x=w2550) -> (-x=w2549:dbl)
                n1592 = Compound Arithmetic op=ADD(w2538, w2548, w2551, w2549) -> (w2531:dbl)
                "Pointer X (V)" <- w2531
                n1593 = Or(x="Set X Only", y="Set Confocal Spot") -> (x .or. y?=w2524:bool)
                n1594 = Or(x="Set Confocal Spot", y="Set Y Only") -> (x .or. y?=w2523:bool)
                n1595 = case shown="True" w2524 {
                  tunnel: w2531 -> [_ w2554]
                  frame False {
                  }
                  frame True {
                    n1596 = property on="MCL X" class="Slide (strict)"("Val(Sgnl)"=w2554) -> ()  [unwired: 2 in, 2 out]
                  }
                }
                n1597 = case shown="True" w2523 {
                  tunnel: w2530 -> [_ w2555]
                  frame False {
                  }
                  frame True {
                    n1598 = property on="MCL Y" class="Slide (strict)"("Val(Sgnl)"=w2555) -> ()  [unwired: 2 in, 2 out]
                  }
                }
              }
            }
          }
          frame 3 {
            n1599 = local read "MouseMove Trap"() -> (w2560:bool)
            n1600 = call-poly <vilib>:"Acquire Input Data.vi"("device ID"=w2558) -> ("axis info"=w2557:T36)  [unwired: 15 in, 3 out]
            n1601 = Unbundle By Name(w2557) -> ("Horizontal"=→"MouseX":i32)
            n1602 = Not(x=w2560) -> (.not. x?=w2559:bool)
            n1603 = local write "MouseMove Trap"(w2559) -> ()
          }
        }
      }
    }
    n1604 = local read "Stop All"() -> (w2461:bool)
  }
  n1605 = while "Key Listener" {
    stop <- w2564 stop-if-true
    n1606 = event shown="[1] Key Down" {
      selector: _ -> [_ _]
      dyn-events: _ -> [_ _]
      timeout: 10 -> [_ _]
      event Timeout {
        n1607 = event-data() -> ()  [unwired: 1 in, 3 out]
      }
      event Key Down {
        # "02  = 1\n16 = q\n30 = a\n44 = z"
        n1608 = event-data() -> ("ScanCode"=w2568:i16, "PlatMods.Shift"=w2567:bool, "FocusObj"=w2566:refnum<vi>)  [unwired: 1 in]
        n1609 = Not A Number/Path/Refnum?(number/path/refnum=w2566) -> (NaN/Path/Refnum?=w2565:bool)
        n1610 = case shown="True" w2565 {
          tunnel: w2568 -> [_ w2570]
          tunnel: w2567 -> [_ w2569]
          frame False {
            # "If there is a FocusObj, let keystrokes play without firing an event"
          }
          frame True {
            n1611 = case shown="33" w2570 {
              tunnel: w2569 -> [_ _ _ _ _ _ _ _ _ _ _ w2587 w2590 w2593 _]
              frame 0, Default {
              }
              frame 1 {
              }
              frame 2 {
                # "1: Toggle TOP"
                n1612 = local read "Inject Top"() -> (w2572:bool)
                n1613 = Not(x=w2572) -> (.not. x?=w2571:bool)
                n1614 = property on="Inject Top" class="Bool (strict)"("Val(Sgnl)"=w2571) -> ()  [unwired: 2 in, 2 out]
              }
              frame 3 {
                # "2: Toggle MAIN"
                n1615 = local read "Inject Main"() -> (w2574:bool)
                n1616 = Not(x=w2574) -> (.not. x?=w2573:bool)
                n1617 = property on="Inject Main" class="Bool (strict)"("Val(Sgnl)"=w2573) -> ()  [unwired: 2 in, 2 out]
              }
              frame 4 {
                # "3: Toggle Bottom"
                n1618 = local read "Inject Bottom"() -> (w2575:bool)
                n1619 = Not(x=w2575) -> (.not. x?=w2576:bool)
                n1620 = property on="Inject Bottom" class="Bool (strict)"("Val(Sgnl)"=w2576) -> ()  [unwired: 2 in, 2 out]
              }
              frame 5 {
                # "4: Shunt 1"
                n1621 = local read "Shunt 1"() -> (w2578:bool)
                n1622 = Not(x=w2578) -> (.not. x?=w2577:bool)
                n1623 = property on="Shunt 1" class="Bool (strict)"("Val(Sgnl)"=w2577) -> ()  [unwired: 2 in, 2 out]
              }
              frame 6 {
                # "5: Shunt 2"
                n1624 = local read "Shunt 2"() -> (w2580:bool)
                n1625 = Not(x=w2580) -> (.not. x?=w2579:bool)
                n1626 = property on="Shunt 2" class="Bool (strict)"("Val(Sgnl)"=w2579) -> ()  [unwired: 2 in, 2 out]
              }
              frame 16 {
                # "Q: Scale Intensities"
                n1627 = local read "Scale intensities (Q)"() -> (w2582:bool)
                n1628 = Not(x=w2582) -> (.not. x?=w2581:bool)
                n1629 = property on="Scale intensities (Q)" class="Bool (strict)"("Val(Sgnl)"=w2581) -> ()  [unwired: 2 in, 2 out]
              }
              frame 17 {
                # "W: ???"
              }
              frame 18 {
                # "E: Trap 1"
                n1630 = local read "Trap 1 (E)"() -> (w2583:bool)
                n1631 = Not(x=w2583) -> (.not. x?=w2584:bool)
                n1632 = property on="Trap 1 (E)" class="Bool (strict)"("Val(Sgnl)"=w2584) -> ()  [unwired: 2 in, 2 out]
              }
              frame 19 {
                # "R: Trap 2"
                n1633 = local read "Trap 2 (R)"() -> (w2586:bool)
                n1634 = Not(x=w2586) -> (.not. x?=w2585:bool)
                n1635 = property on="Trap 2 (R)" class="Bool (strict)"("Val(Sgnl)"=w2585) -> ()  [unwired: 2 in, 2 out]
              }
              frame 30 {
                # "A: Go Top\nShift+A: Save Top"
                n1636 = case shown="True" w2587 {
                  frame False {
                    n1637 = property on="Go Top" class="Bool (strict)"("Val(Sgnl)"=TRUE ("Value (Signaling)")) -> ()  [unwired: 2 in, 2 out]
                  }
                  frame True {
                    n1638 = property on="Capture Top" class="Bool (strict)"("Val(Sgnl)"=FALSE ("Value (Signaling)")) -> ()  [unwired: 2 in, 2 out]
                  }
                }
              }
              frame 31 {
                # "S: Goto Bottom\nShift+S: Save Bottom"
                n1639 = case shown="True" w2590 {
                  frame False {
                    n1640 = property on="Go Bottom" class="Bool (strict)"("Val(Sgnl)"=TRUE ("Value (Signaling)")) -> ()  [unwired: 2 in, 2 out]
                  }
                  frame True {
                    n1641 = property on="Capture Exp" class="Bool (strict)"("Val(Sgnl)"=TRUE ("Value (Signaling)")) -> ()  [unwired: 2 in, 2 out]
                  }
                }
              }
              frame 32 {
                # "D: Go Bottom\nShift+D: Save Bottom"
                n1642 = case shown="False" w2593 {
                  frame False {
                    n1643 = property on="Go Exp (F8)" class="Bool (strict)"("Val(Sgnl)"=TRUE ("Value (Signaling)")) -> ()  [unwired: 2 in, 2 out]
                  }
                  frame True {
                    n1644 = property on="Capture Bottom" class="Bool (strict)"("Val(Sgnl)"=TRUE ("Value (Signaling)")) -> ()  [unwired: 2 in, 2 out]
                  }
                }
              }
              frame 33 {
                # "F: Toggle AFish"
              }
            }
          }
        }
      }
    }
    n1645 = local read "Stop All"() -> (w2564:bool)
  }
  n1646 = node-c288(w82) -> ()  [unwired: 1 out]
  n1647 = node-c288(w38) -> ()  [unwired: 1 out]
  n1648 = node-c288(w77) -> ()  [unwired: 1 out]
  n1649 = node-c288(w161) -> ()  [unwired: 1 out]
  n1650 = flat-sequence "@Alex - Set stage to 0,0,0 on exit" {
    tunnel: w12 -> [w2597]
    tunnel: [w2596] -> w11
    frame #0 {
      n1651 = local read "ESP Port"() -> (w2601:refnum<visa-resource-name>)
      n1652 = Concatenate Strings("1PA0;\n2PA0;\n3PA0" ("write buffer"), "\r") -> (w2598:string)
      n1653 = VISA Write(VISA resource name=w2601, write buffer=w2598, error in (no error)=w2597) -> (error out=w2596:errorcluster)  [unwired: 2 out]
    }
  }
  n1654 = flat-sequence {
    tunnel: w49 -> [w2606]
    tunnel: [w2605] -> w53
    tunnel: [w2602] -> w52
    tunnel: w51 -> [_]
    tunnel: w50 -> [_]
    tunnel: w11 -> [w2603]
    tunnel: w53 -> [w2611]
    tunnel: w52 -> [w2610]
    frame #0 {
      w2604 = FALSE ("APD to FIFO")
      n1655 = xnode "Read/Write Control"("FPGA VI Reference In"=w2606, "error in"=w2603, "APD to FIFO"=w2604, "AI to FIFO"=w2604) -> ("FPGA VI Reference Out"=w2605:T18, "error out"=w2602:errorcluster)
    }
    frame #1 {
      n1656 = xnode "Invoke Method"("FPGA VI Reference In"=w2611, "error in"=w2610) -> ("FPGA VI Reference Out"=w2609:T18, "error out"=w2608:errorcluster)
      n1657 = xnode "Close FPGA VI Reference"("FPGA VI Reference In"=w2609, "error in"=w2608) -> ("error out"=w2607:errorcluster)
      n1658 = call <vilib>:"Simple Error Handler.vi"("error in (no error)"=w2607) -> ()  [unwired: 4 in, 5 out]
    }
  }
  "Fish Status" <- w10
